vi "test Parse.vi"(11 "Test Case In":refnum<class "test EDS.lvclass">) -> (0 "error out":errorcluster, 3 "Test Case Out":refnum<class "test EDS.lvclass">)   [LabVIEW 2024, in "Test EDS.lvclass"]
uses:
  test EDS.lvclass
  C:/Program Files/National Instruments/LabVIEW 2024/vi.lib/Astemes/LUnit/Test Case.lvclass
  Core/EDS/EDS.lvclass
  <vilib>/PNR/JSONtext Object Serialization/Generic Object Serializer/Generic Object Serializer.lvclass
  C:/Program Files/National Instruments/LabVIEW 2024/vi.lib/JDP Science/JSONtext/LVClass Serializer/JSONtext LVClass Serializer.lvclass
  <vilib>/PNR/JSONtext Object Serialization/Generic Object Serializer/Type Name Handling.ctl
  <vilib>/PNR/JSONtext Object Serialization/Generic Object Serializer/Generic Object Serializer.lvclass/Generic Object Serializer.ctl
  Core/EDS/EDS.lvclass/EDS.ctl
  <vilib>/Astemes/LUnit/Test Case.lvclass/Test Case.ctl
  bdd25f00-0f07-479c-b713-0b173a884aa2.vi
  4993e8ee-a06a-463a-9684-69129f64d5ce.vi
  <vilib>/PNR/JSONtext Object Serialization/Generic Object Serializer/Write Type Name Handling.vi
  <vilib>/Astemes/LUnit/Append Pass Result.vi
  <vilib>/Astemes/LUnit/Append Fail Result.vi
  <vilib>/Astemes/LUnit/Describe Comparison.vi
  4993e8ee-a06a-463a-9684-69129f64d5ce.vi/9c5d11cd-9439-4240-a1ee-d9baace9c924.vi
  <vilib>/Astemes/LUnit/Run In UI.vi
  <vilib>/Utility/error.llb/Clear Errors.vi
  <vilib>/JDP Science/JSONtext/Variant to JSON Text.vi
  <vilib>/Astemes/LUnit/Describe Variant.vi
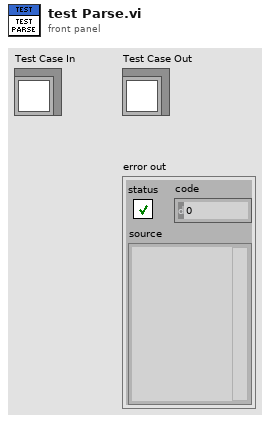
[diagram p1: front panel]
types:
  T1 = typedef "Generic Object Serializer.lvclass/Type Name Handling.ctl" = enum16{"None", "Inline"}
diagram:
  w9 = refnum<class "Generic Object Serializer.lvclass"> refnum  # Generic Object Serializer
  n1 = Current VI's Path() -> (path=w16:path)
  n2 = Strip Path(path=w16) -> (stripped path=w11:path)  [unwired: 1 out]
  n3 = Build Path(base path=w11, name or relative path=path "test.eds") -> (appended path=w12:path)
  n4 = Write to Text File(file (use dialog)=w12, text="[FileInfo]\nCreatedBy=Nanotec Electronic GmbH & Co. KG\nModifiedBy=Nanotec Electronic GmbH & Co. KG\nDescription=Motion controller\nCreationTime=00:00AM\nCreationDate=01-01-2000\nModificationTime=00:00AM\nModificationDate=01-01-2000\nFileName=C5-E-2-09.eds\nFileVersion=1\nFileRevision=1\nEDSVersion=4.0\n\n[DeviceInfo]\nVendorName=Nanotec Electronic GmbH & Co. KG\nVendorNumber=0x26C\nProductName=C5-E-2-09\nProductNumber=0x11\nRevisionNumber=0x8A50000\nOrderCode=na\nBaudRate_10=1\nBaudRate_20=1\nBaudRate_50=1\nBaudRate_125=1\nBaudRate_250=1\nBaudRate_500=1\nBaudRate_800=0\nBaudRate_1000=1\nSimpleBootUpMaster=0\nSimpleBootUpSlave=0\nGranularity=8\nDynamicChannelsSupported=0\nCompactPDO=0\nGroupMessaging=0\nNrOfRXPDO=8\nNrOfTXPDO=8\nLSS_Supported=0\n\n[DummyUsage]\nDummy0001=0\nDummy0002=1\nDummy0003=1\nDummy0004=1\nDummy0005=1\nDummy0006=1\nDummy0007=1\n\n[Comments]\nLines=0x00\n\n[MandatoryObjects]\nSupportedObjects=0x03\n1=0x1000\n2=0x1001\n3=0x1018\n\n[1000]\nParameterName=Device Type\nObjectType=0x7\nDataType=0x0007\nAccessType=ro\nDefaultValue=0x00060192\nPDOMapping=0\nObjFlags=1\n\n[1001]\nParameterName=Error Register\nObjectType=0x7\nDataType=0x0005\nAccessType=ro\nDefaultValue=0x00\nPDOMapping=1\nObjFlags=1\n\n[1018]\nParameterName=Identity Object\nObjectType=0x9\nSubNumber=0x05\n\n[1018sub0]\nParameterName=Number of entries\nObjectType=0x7\nDataType=0x0005\nAccessType=ro\nDefaultValue=0x04\nPDOMapping=0\nObjFlags=1\n\n[1018sub1]\nParameterName=Vendor-ID\nObjectType=0x7\nDataType=0x0007\nAccessType=ro\nDefaultValue=0x0000026C\nPDOMapping=0\nObjFlags=1\n\n[1018sub2]\nParameterName=Product code\nObjectType=0x7\nDataType=0x0007\nAccessType=ro\nDefaultValue=0x00000011\nPDOMapping=0\nObjFlags=1\n\n[1018sub3]\nParameterName=Revision number\nObjectType=0x7\nDataType=0x0007\nAccessType=ro\nDefaultValue=0x08A50000\nPDOMapping=0\nObjFlags=1\n\n[1018sub4]\nParameterName=Serial number\nObjectType=0x7\nDataType=0x0007\nAccessType=ro\nDefaultValue=\nPDOMapping=0\nObjFlags=1\n\n[OptionalObjects]\nSupportedObjects=0x91\n1=0x1003\n2=0x1005\n3=0x1006\n4=0x1007\n5=0x1008\n6=0x1009\n7=0x100A\n8=0x100C\n9=0x100D\n10=0x1010\n11=0x1011\n12=0x1014\n13=0x1016\n14=0x1017\n15=0x1019\n16=0x1020\n17=0x1029\n18=0x1400\n19=0x1401\n20=0x1402\n21=0x1403\n22=0x1404\n23=0x1405\n24=0x1406\n25=0x1407\n26=0x1600\n27=0x1601\n28=0x1602\n29=0x1603\n30=0x1604\n31=0x1605\n32=0x1606\n33=0x1607\n34=0x1800\n35=0x1801\n36=0x1802\n37=0x1803\n38=0x1804\n39=0x1805\n40=0x1806\n41=0x1807\n42=0x1A00\n43=0x1A01\n44=0x1A02\n45=0x1A03\n46=0x1A04\n47=0x1A05\n48=0x1A06\n49=0x1A07\n50=0x1F50\n51=0x1F51\n52=0x1F57\n53=0x1F80\n54=0x6007\n55=0x603F\n56=0x6040\n57=0x6041\n58=0x6042\n59=0x6043\n60=0x6044\n61=0x6046\n62=0x6048\n63=0x6049\n64=0x604A\n65=0x604C\n66=0x605A\n67=0x605B\n68=0x605C\n69=0x605D\n70=0x605E\n71=0x6060\n72=0x6061\n73=0x6062\n74=0x6063\n75=0x6064\n76=0x6065\n77=0x6066\n78=0x6067\n79=0x6068\n80=0x606B\n81=0x606C\n82=0x606D\n83=0x606E\n84=0x606F\n85=0x6070\n86=0x6071\n87=0x6072\n88=0x6073\n89=0x6074\n90=0x6075\n91=0x6077\n92=0x607A\n93=0x607B\n94=0x607C\n95=0x607D\n96=0x607E\n97=0x607F\n98=0x6080\n99=0x6081\n100=0x6082\n101=0x6083\n102=0x6084\n103=0x6085\n104=0x6086\n105=0x6087\n106=0x608F\n107=0x6090\n108=0x6091\n109=0x6092\n110=0x6096\n111=0x6097\n112=0x6098\n113=0x6099\n114=0x609A\n115=0x60A2\n116=0x60A4\n117=0x60A8\n118=0x60A9\n119=0x60B0\n120=0x60B1\n121=0x60B2\n122=0x60C1\n123=0x60C2\n124=0x60C4\n125=0x60C5\n126=0x60C6\n127=0x60E4\n128=0x60E5\n129=0x60E6\n130=0x60E8\n131=0x60E9\n132=0x60EB\n133=0x60ED\n134=0x60EE\n135=0x60F2\n136=0x60F4\n137=0x60F8\n138=0x60FA\n139=0x60FC\n140=0x60FD\n141=0x60FE\n142=0x60FF\n143=0x6502\n144=0x6503\n145=0x6505\n\n[1003]\nParameterName=Pre-defined error field\nObjectType=0x8\nSubNumber=0x09\n\n[1003sub0]\nParameterName=Number of errors\nObjectType=0x7\nDataType=0x0005\nAccessType=rw\nDefaultValue=0x00\nPDOMapping=0\nObjFlags=1\n\n[1003sub1]\nParameterName=1st Standard error field\nObjectType=0x7\nDataType=0x0007\nAccessType=ro\nPDOMapping=0\nObjFlags=1\n\n[1003sub2]\nParameterName=2nd Standard error field\nObjectType=0x7\nDataType=0x0007\nAccessType=ro\nPDOMapping=0\nObjFlags=1\n\n[1003sub3]\nParameterName=3th Standard error field\nObjectType=0x7\nDataType=0x0007\nAccessType=ro\nPDOMapping=0\nObjFlags=1\n\n[1003sub4]\nParameterName=4th Standard error field\nObjectType=0x7\nDataType=0x0007\nAccessType=ro\nPDOMapping=0\nObjFlags=1\n\n[1003sub5]\nParameterName=5th Standard error field\nObjectType=0x7\nDataType=0x0007\nAccessType=ro\nPDOMapping=0\nObjFlags=1\n\n[1003sub6]\nParameterName=6th Standard error field\nObjectType=0x7\nDataType=0x0007\nAccessType=ro\nPDOMapping=0\nObjFlags=1\n\n[1003sub7]\nParameterName=7th Standard error field\nObjectType=0x7\nDataType=0x0007\nAccessType=ro\nPDOMapping=0\nObjFlags=1\n\n[1003sub8]\nParameterName=8th Standard error field\nObjectType=0x7\nDataType=0x0007\nAccessType=ro\nPDOMapping=0\nObjFlags=1\n\n[1005]\nParameterName=COB-ID Sync\nObjectType=0x7\nDataType=0x0007\nAccessType=rw\nDefaultValue=0x00000080\nPDOMapping=0\n\n[1006]\nParameterName=Communication cycle period\nObjectType=0x7\nDataType=0x0007\nAccessType=rw\nDefaultValue=0x00000000\nPDOMapping=0\n\n[1007]\nParameterName=Synchronous Window Length\nObjectType=0x7\nDataType=0x0007\nAccessType=rw\nDefaultValue=0x00000000\nPDOMapping=0\n\n[1008]\nParameterName=Manufacturer Device Name\nObjectType=0x7\nDataType=0x0009\nAccessType=const\nDefaultValue=C5-E-2-09\nPDOMapping=0\nObjFlags=1\n\n[1009]\nParameterName=Manufacturer Hardware Version\nObjectType=0x7\nDataType=0x0009\nAccessType=const\nDefaultValue=\nPDOMapping=0\nObjFlags=1\n\n[100A]\nParameterName=Manufacturer Software Version\nObjectType=0x7\nDataType=0x0009\nAccessType=const\nDefaultValue=FIR-v2213-B1031134\nPDOMapping=0\nObjFlags=1\n\n[100C]\nParameterName=Guard Time\nObjectType=0x7\nDataType=0x0006\nAccessType=rw\nDefaultValue=0x0000\nPDOMapping=0\n\n[100D]\nParameterName=Live Time Factor\nObjectType=0x7\nDataType=0x0005\nAccessType=rw\nDefaultValue=0x00\nPDOMapping=0\n\n[1010]\nParameterName=Store parameters\nObjectType=0x8\nSubNumber=0x0E\n\n[1010sub0]\nParameterName=Number of entries\nObjectType=0x7\nDataType=0x0005\nAccessType=ro\nDefaultValue=0x0D\nPDOMapping=0\nObjFlags=1\n\n[1010sub1]\nParameterName=Save all parameters to non-volatile memory\nObjectType=0x7\nDataType=0x0007\nAccessType=rw\nDefaultValue=0x00000001\nPDOMapping=0\nObjFlags=1\n\n[1010sub2]\nParameterName=Save communication parameters to non-volatile memory\nObjectType=0x7\nDataType=0x0007\nAccessType=rw\nDefaultValue=0x00000001\nPDOMapping=0\nObjFlags=1\n\n[1010sub3]\nParameterName=Save application parameters to non-volatile memory\nObjectType=0x7\nDataType=0x0007\nAccessType=rw\nDefaultValue=0x00000001\nPDOMapping=0\nObjFlags=1\n\n[1010sub4]\nParameterName=Save customer parameters to non-volatile memory\nObjectType=0x7\nDataType=0x0007\nAccessType=rw\nDefaultValue=0x00000001\nPDOMapping=0\nObjFlags=1\n\n[1010sub5]\nParameterName=Save drive parameters to non-volatile memory\nObjectType=0x7\nDataType=0x0007\nAccessType=rw\nDefaultValue=0x00000001\nPDOMapping=0\nObjFlags=1\n\n[1010sub6]\nParameterName=Save tuning parameters to non-volatile memory\nObjectType=0x7\nDataType=0x0007\nAccessType=rw\nDefaultValue=0x00000001\nPDOMapping=0\nObjFlags=1\n\n[1010sub7]\nParameterName=Save miscellaneous configurations to non-volatile memory\nObjectType=0x7\nDataType=0x0007\nAccessType=rw\nDefaultValue=0x00000001\nPDOMapping=0\nObjFlags=1\n\n[1010sub8]\nParameterName=Save reserved1 configurations to non-volatile memory\nObjectType=0x7\nDataType=0x0007\nAccessType=rw\nDefaultValue=0x00000000\nPDOMapping=0\nObjFlags=1\n\n[1010sub9]\nParameterName=Save reserved2 configurations to non-volatile memory\nObjectType=0x7\nDataType=0x0007\nAccessType=rw\nDefaultValue=0x00000000\nPDOMapping=0\nObjFlags=1\n\n[1010subA]\nParameterName=Save CANopen configurations to non-volatile memory\nObjectType=0x7\nDataType=0x0007\nAccessType=rw\nDefaultValue=0x00000001\nPDOMapping=0\nObjFlags=1\n\n[1010subB]\nParameterName=Save Modbus RTU configurations to non-volatile memory\nObjectType=0x7\nDataType=0x0007\nAccessType=rw\nDefaultValue=0x00000001\nPDOMapping=0\nObjFlags=1\n\n[1010subC]\nParameterName=Save Ethernet configurations to non-volatile memory\nObjectType=0x7\nDataType=0x0007\nAccessType=rw\nDefaultValue=0x00000001\nPDOMapping=0\nObjFlags=1\n\n[1010subD]\nParameterName=Save Profibus configurations to non-volatile memory\nObjectType=0x7\nDataType=0x0007\nAccessType=rw\nDefaultValue=0x00000001\nPDOMapping=0\nObjFlags=1\n\n[1011]\nParameterName=Restore default parameters\nObjectType=0x8\nSubNumber=0x0E\n\n[1011sub0]\nParameterName=Number of entries\nObjectType=0x7\nDataType=0x0005\nAccessType=ro\nDefaultValue=0x0D\nPDOMapping=0\nObjFlags=1\n\n[1011sub1]\nParameterName=Restore all default parameters\nObjectType=0x7\nDataType=0x0007\nAccessType=rw\nDefaultValue=0x00000001\nPDOMapping=0\nObjFlags=1\n\n[1011sub2]\nParameterName=Restore communication default parameters\nObjectType=0x7\nDataType=0x0007\nAccessType=rw\nDefaultValue=0x00000001\nPDOMapping=0\nObjFlags=1\n\n[1011sub3]\nParameterName=Restore application default parameters\nObjectType=0x7\nDataType=0x0007\nAccessType=rw\nDefaultValue=0x00000001\nPDOMapping=0\nObjFlags=1\n\n[1011sub4]\nParameterName=Restore customer default parameters\nObjectType=0x7\nDataType=0x0007\nAccessType=rw\nDefaultValue=0x00000001\nPDOMapping=0\nObjFlags=1\n\n[1011sub5]\nParameterName=Restore drive default parameters\nObjectType=0x7\nDataType=0x0007\nAccessType=rw\nDefaultValue=0x00000001\nPDOMapping=0\nObjFlags=1\n\n[1011sub6]\nParameterName=Restore tuning default parameters\nObjectType=0x7\nDataType=0x0007\nAccessType=rw\nDefaultValue=0x00000001\nPDOMapping=0\nObjFlags=1\n\n[1011sub7]\nParameterName=Restore miscellaneous configurations\nObjectType=0x7\nDataType=0x0007\nAccessType=rw\nDefaultValue=0x00000001\nPDOMapping=0\nObjFlags=1\n\n[1011sub8]\nParameterName=Restore reserved1 configurations to non-volatile memory\nObjectType=0x7\nDataType=0x0007\nAccessType=rw\nDefaultValue=0x00000000\nPDOMapping=0\nObjFlags=1\n\n[1011sub9]\nParameterName=Restore reserved2 configurations to non-volatile memory\nObjectType=0x7\nDataType=0x0007\nAccessType=rw\nDefaultValue=0x00000000\nPDOMapping=0\nObjFlags=1\n\n[1011subA]\nParameterName=Restore CANopen configurations to non-volatile memory\nObjectType=0x7\nDataType=0x0007\nAccessType=rw\nDefaultValue=0x00000001\nPDOMapping=0\nObjFlags=1\n\n[1011subB]\nParameterName=Restore Modbus RTU configurations to non-volatile memory\nObjectType=0x7\nDataType=0x0007\nAccessType=rw\nDefaultValue=0x00000001\nPDOMapping=0\nObjFlags=1\n\n[1011subC]\nParameterName=Restore Ethernet configurations to non-volatile memory\nObjectType=0x7\nDataType=0x0007\nAccessType=rw\nDefaultValue=0x00000001\nPDOMapping=0\nObjFlags=1\n\n[1011subD]\nParameterName=Restore Profibus configurations to non-volatile memory\nObjectType=0x7\nDataType=0x0007\nAccessType=rw\nDefaultValue=0x00000001\nPDOMapping=0\nObjFlags=1\n\n[1014]\nParameterName=COB-ID EMCY\nObjectType=0x7\nDataType=0x0007\nAccessType=rw\nDefaultValue=$NODEID+0x80\nPDOMapping=0\n\n[1016]\nParameterName=Consumer heartbeat time\nObjectType=0x8\nSubNumber=0x02\n\n[1016sub0]\nParameterName=Number of entries\nObjectType=0x7\nDataType=0x0005\nAccessType=ro\nDefaultValue=0x01\nPDOMapping=0\n\n[1016sub1]\nParameterName=Consumer heartbeat time\nObjectType=0x7\nDataType=0x0007\nAccessType=rw\nDefaultValue=0x00000000\nPDOMapping=0\n\n[1017]\nParameterName=Producer heartbeat time\nObjectType=0x7\nDataType=0x0006\nAccessType=rw\nDefaultValue=0x0000\nPDOMapping=0\n\n[1019]\nParameterName=Synchronous counter overflow value\nObjectType=0x7\nDataType=0x0005\nAccessType=rw\nDefaultValue=0x00\nPDOMapping=0\n\n[1020]\nParameterName=Verify Configuration\nObjectType=0x8\nSubNumber=0x03\n\n[1020sub0]\nParameterName=Number of entries\nObjectType=0x7\nDataType=0x0005\nAccessType=ro\nDefaultValue=0x02\nPDOMapping=0\n\n[1020sub1]\nParameterName=Configuration date\nObjectType=0x7\nDataType=0x0007\nAccessType=rw\nDefaultValue=0x00000000\nPDOMapping=0\n\n[1020sub2]\nParameterName=Configuration time\nObjectType=0x7\nDataType=0x0007\nAccessType=rw\nDefaultValue=0x00000000\nPDOMapping=0\n\n[1029]\nParameterName=Error behavior\nObjectType=0x8\nSubNumber=0x03\n\n[1029sub0]\nParameterName=Number of entries\nObjectType=0x7\nDataType=0x0005\nAccessType=ro\nDefaultValue=0x02\nPDOMapping=0\n\n[1029sub1]\nParameterName=Communication error\nObjectType=0x7\nDataType=0x0005\nAccessType=rw\nDefaultValue=0x00\nPDOMapping=0\n\n[1029sub2]\nParameterName=Internal device error\nObjectType=0x7\nDataType=0x0005\nAccessType=rw\nDefaultValue=0x01\nPDOMapping=0\n\n[1400]\nParameterName=Receive PDO 1 Communication Parameter\nObjectType=0x9\nSubNumber=0x03\n\n[1400sub0]\nParameterName=Number of entries\nObjectType=0x7\nDataType=0x0005\nAccessType=ro\nDefaultValue=0x02\nPDOMapping=0\n\n[1400sub1]\nParameterName=COB-ID\nObjectType=0x7\nDataType=0x0007\nAccessType=rw\nDefaultValue=$NODEID+0x200\nPDOMapping=0\n\n[1400sub2]\nParameterName=Transmission Type\nObjectType=0x7\nDataType=0x0005\nAccessType=rw\nDefaultValue=0xFF\nPDOMapping=0\n\n[1401]\nParameterName=Receive PDO 2 Communication Parameter\nObjectType=0x9\nSubNumber=0x03\n\n[1401sub0]\nParameterName=Number of entries\nObjectType=0x7\nDataType=0x0005\nAccessType=ro\nDefaultValue=0x02\nPDOMapping=0\n\n[1401sub1]\nParameterName=COB-ID\nObjectType=0x7\nDataType=0x0007\nAccessType=rw\nDefaultValue=$NODEID+0x300\nPDOMapping=0\n\n[1401sub2]\nParameterName=Transmission Type\nObjectType=0x7\nDataType=0x0005\nAccessType=rw\nDefaultValue=0xFF\nPDOMapping=0\n\n[1402]\nParameterName=Receive PDO 3 Communication Parameter\nObjectType=0x9\nSubNumber=0x03\n\n[1402sub0]\nParameterName=Number of entries\nObjectType=0x7\nDataType=0x0005\nAccessType=ro\nDefaultValue=0x02\nPDOMapping=0\n\n[1402sub1]\nParameterName=COB-ID\nObjectType=0x7\nDataType=0x0007\nAccessType=rw\nDefaultValue=$NODEID+0x400\nPDOMapping=0\n\n[1402sub2]\nParameterName=Transmission Type\nObjectType=0x7\nDataType=0x0005\nAccessType=rw\nDefaultValue=0xFF\nPDOMapping=0\n\n[1403]\nParameterName=Receive PDO 4 Communication Parameter\nObjectType=0x9\nSubNumber=0x03\n\n[1403sub0]\nParameterName=Number of entries\nObjectType=0x7\nDataType=0x0005\nAccessType=ro\nDefaultValue=0x02\nPDOMapping=0\n\n[1403sub1]\nParameterName=COB-ID\nObjectType=0x7\nDataType=0x0007\nAccessType=rw\nDefaultValue=$NODEID+0x500\nPDOMapping=0\n\n[1403sub2]\nParameterName=Transmission Type\nObjectType=0x7\nDataType=0x0005\nAccessType=rw\nDefaultValue=0xFF\nPDOMapping=0\n\n[1404]\nParameterName=Receive PDO 5 Communication Parameter\nObjectType=0x9\nSubNumber=0x03\n\n[1404sub0]\nParameterName=Number of entries\nObjectType=0x7\nDataType=0x0005\nAccessType=ro\nDefaultValue=0x02\nPDOMapping=0\n\n[1404sub1]\nParameterName=COB-ID\nObjectType=0x7\nDataType=0x0007\nAccessType=rw\nDefaultValue=0x80000000\nPDOMapping=0\n\n[1404sub2]\nParameterName=Transmission Type\nObjectType=0x7\nDataType=0x0005\nAccessType=rw\nDefaultValue=0xFF\nPDOMapping=0\n\n[1405]\nParameterName=Receive PDO 6 Communication Parameter\nObjectType=0x9\nSubNumber=0x03\n\n[1405sub0]\nParameterName=Number of entries\nObjectType=0x7\nDataType=0x0005\nAccessType=ro\nDefaultValue=0x02\nPDOMapping=0\n\n[1405sub1]\nParameterName=COB-ID\nObjectType=0x7\nDataType=0x0007\nAccessType=rw\nDefaultValue=0x80000000\nPDOMapping=0\n\n[1405sub2]\nParameterName=Transmission Type\nObjectType=0x7\nDataType=0x0005\nAccessType=rw\nDefaultValue=0xFF\nPDOMapping=0\n\n[1406]\nParameterName=Receive PDO 7 Communication Parameter\nObjectType=0x9\nSubNumber=0x03\n\n[1406sub0]\nParameterName=Number of entries\nObjectType=0x7\nDataType=0x0005\nAccessType=ro\nDefaultValue=0x02\nPDOMapping=0\n\n[1406sub1]\nParameterName=COB-ID\nObjectType=0x7\nDataType=0x0007\nAccessType=rw\nDefaultValue=0x80000000\nPDOMapping=0\n\n[1406sub2]\nParameterName=Transmission Type\nObjectType=0x7\nDataType=0x0005\nAccessType=rw\nDefaultValue=0xFF\nPDOMapping=0\n\n[1407]\nParameterName=Receive PDO 8 Communication Parameter\nObjectType=0x9\nSubNumber=0x03\n\n[1407sub0]\nParameterName=Number of entries\nObjectType=0x7\nDataType=0x0005\nAccessType=ro\nDefaultValue=0x02\nPDOMapping=0\n\n[1407sub1]\nParameterName=COB-ID\nObjectType=0x7\nDataType=0x0007\nAccessType=rw\nDefaultValue=0x80000000\nPDOMapping=0\n\n[1407sub2]\nParameterName=Transmission Type\nObjectType=0x7\nDataType=0x0005\nAccessType=rw\nDefaultValue=0xFF\nPDOMapping=0\n\n[1600]\nParameterName=Receive PDO 1 Mapping Parameter\nObjectType=0x9\nSubNumber=0x09\n\n[1600sub0]\nParameterName=Number of entries\nObjectType=0x7\nDataType=0x0005\nAccessType=rw\nDefaultValue=0x02\nPDOMapping=0\n\n[1600sub1]\nParameterName=1st object to be mapped\nObjectType=0x7\nDataType=0x0007\nAccessType=rw\nDefaultValue=0x60400010\nPDOMapping=0\n\n[1600sub2]\nParameterName=2nd object to be mapped\nObjectType=0x7\nDataType=0x0007\nAccessType=rw\nDefaultValue=0x60600008\nPDOMapping=0\n\n[1600sub3]\nParameterName=3rd object to be mapped\nObjectType=0x7\nDataType=0x0007\nAccessType=rw\nDefaultValue=0x00000000\nPDOMapping=0\n\n[1600sub4]\nParameterName=4th object to be mapped\nObjectType=0x7\nDataType=0x0007\nAccessType=rw\nDefaultValue=0x00000000\nPDOMapping=0\n\n[1600sub5]\nParameterName=5th object to be mapped\nObjectType=0x7\nDataType=0x0007\nAccessType=rw\nDefaultValue=0x00000000\nPDOMapping=0\n\n[1600sub6]\nParameterName=6th object to be mapped\nObjectType=0x7\nDataType=0x0007\nAccessType=rw\nDefaultValue=0x00000000\nPDOMapping=0\n\n[1600sub7]\nParameterName=7th object to be mapped\nObjectType=0x7\nDataType=0x0007\nAccessType=rw\nDefaultValue=0x00000000\nPDOMapping=0\n\n[1600sub8]\nParameterName=8th object to be mapped\nObjectType=0x7\nDataType=0x0007\nAccessType=rw\nDefaultValue=0x00000000\nPDOMapping=0\n\n[1601]\nParameterName=Receive PDO 2 Mapping Parameter\nObjectType=0x9\nSubNumber=0x09\n\n[1601sub0]\nParameterName=Number of entries\nObjectType=0x7\nDataType=0x0005\nAccessType=rw\nDefaultValue=0x02\nPDOMapping=0\n\n[1601sub1]\nParameterName=1st object to be mapped\nObjectType=0x7\nDataType=0x0007\nAccessType=rw\nDefaultValue=0x607A0020\nPDOMapping=0\n\n[1601sub2]\nParameterName=2nd object to be mapped\nObjectType=0x7\nDataType=0x0007\nAccessType=rw\nDefaultValue=0x60810020\nPDOMapping=0\n\n[1601sub3]\nParameterName=3rd object to be mapped\nObjectType=0x7\nDataType=0x0007\nAccessType=rw\nDefaultValue=0x00000000\nPDOMapping=0\n\n[1601sub4]\nParameterName=4th object to be mapped\nObjectType=0x7\nDataType=0x0007\nAccessType=rw\nDefaultValue=0x00000000\nPDOMapping=0\n\n[1601sub5]\nParameterName=5th object to be mapped\nObjectType=0x7\nDataType=0x0007\nAccessType=rw\nDefaultValue=0x00000000\nPDOMapping=0\n\n[1601sub6]\nParameterName=6th object to be mapped\nObjectType=0x7\nDataType=0x0007\nAccessType=rw\nDefaultValue=0x00000000\nPDOMapping=0\n\n[1601sub7]\nParameterName=7th object to be mapped\nObjectType=0x7\nDataType=0x0007\nAccessType=rw\nDefaultValue=0x00000000\nPDOMapping=0\n\n[1601sub8]\nParameterName=8th object to be mapped\nObjectType=0x7\nDataType=0x0007\nAccessType=rw\nDefaultValue=0x00000000\nPDOMapping=0\n\n[1602]\nParameterName=Receive PDO 3 Mapping Parameter\nObjectType=0x9\nSubNumber=0x09\n\n[1602sub0]\nParameterName=Number of entries\nObjectType=0x7\nDataType=0x0005\nAccessType=rw\nDefaultValue=0x01\nPDOMapping=0\n\n[1602sub1]\nParameterName=1st object to be mapped\nObjectType=0x7\nDataType=0x0007\nAccessType=rw\nDefaultValue=0x60420010\nPDOMapping=0\n\n[1602sub2]\nParameterName=2nd object to be mapped\nObjectType=0x7\nDataType=0x0007\nAccessType=rw\nDefaultValue=0x00000000\nPDOMapping=0\n\n[1602sub3]\nParameterName=3rd object to be mapped\nObjectType=0x7\nDataType=0x0007\nAccessType=rw\nDefaultValue=0x00000000\nPDOMapping=0\n\n[1602sub4]\nParameterName=4th object to be mapped\nObjectType=0x7\nDataType=0x0007\nAccessType=rw\nDefaultValue=0x00000000\nPDOMapping=0\n\n[1602sub5]\nParameterName=5th object to be mapped\nObjectType=0x7\nDataType=0x0007\nAccessType=rw\nDefaultValue=0x00000000\nPDOMapping=0\n\n[1602sub6]\nParameterName=6th object to be mapped\nObjectType=0x7\nDataType=0x0007\nAccessType=rw\nDefaultValue=0x00000000\nPDOMapping=0\n\n[1602sub7]\nParameterName=7th object to be mapped\nObjectType=0x7\nDataType=0x0007\nAccessType=rw\nDefaultValue=0x00000000\nPDOMapping=0\n\n[1602sub8]\nParameterName=8th object to be mapped\nObjectType=0x7\nDataType=0x0007\nAccessType=rw\nDefaultValue=0x00000000\nPDOMapping=0\n\n[1603]\nParameterName=Receive PDO 4 Mapping Parameter\nObjectType=0x9\nSubNumber=0x09\n\n[1603sub0]\nParameterName=Number of entries\nObjectType=0x7\nDataType=0x0005\nAccessType=rw\nDefaultValue=0x01\nPDOMapping=0\n\n[1603sub1]\nParameterName=1st object to be mapped\nObjectType=0x7\nDataType=0x0007\nAccessType=rw\nDefaultValue=0x60FE0120\nPDOMapping=0\n\n[1603sub2]\nParameterName=2nd object to be mapped\nObjectType=0x7\nDataType=0x0007\nAccessType=rw\nDefaultValue=0x00000000\nPDOMapping=0\n\n[1603sub3]\nParameterName=3rd object to be mapped\nObjectType=0x7\nDataType=0x0007\nAccessType=rw\nDefaultValue=0x00000000\nPDOMapping=0\n\n[1603sub4]\nParameterName=4th object to be mapped\nObjectType=0x7\nDataType=0x0007\nAccessType=rw\nDefaultValue=0x00000000\nPDOMapping=0\n\n[1603sub5]\nParameterName=5th object to be mapped\nObjectType=0x7\nDataType=0x0007\nAccessType=rw\nDefaultValue=0x00000000\nPDOMapping=0\n\n[1603sub6]\nParameterName=6th object to be mapped\nObjectType=0x7\nDataType=0x0007\nAccessType=rw\nDefaultValue=0x00000000\nPDOMapping=0\n\n[1603sub7]\nParameterName=7th object to be mapped\nObjectType=0x7\nDataType=0x0007\nAccessType=rw\nDefaultValue=0x00000000\nPDOMapping=0\n\n[1603sub8]\nParameterName=8th object to be mapped\nObjectType=0x7\nDataType=0x0007\nAccessType=rw\nDefaultValue=0x00000000\nPDOMapping=0\n\n[1604]\nParameterName=Receive PDO 5 Mapping Parameter\nObjectType=0x9\nSubNumber=0x09\n\n[1604sub0]\nParameterName=Number of entries\nObjectType=0x7\nDataType=0x0005\nAccessType=rw\nDefaultValue=0x00\nPDOMapping=0\n\n[1604sub1]\nParameterName=1st object to be mapped\nObjectType=0x7\nDataType=0x0007\nAccessType=rw\nDefaultValue=0x00000000\nPDOMapping=0\n\n[1604sub2]\nParameterName=2nd object to be mapped\nObjectType=0x7\nDataType=0x0007\nAccessType=rw\nDefaultValue=0x00000000\nPDOMapping=0\n\n[1604sub3]\nParameterName=3rd object to be mapped\nObjectType=0x7\nDataType=0x0007\nAccessType=rw\nDefaultValue=0x00000000\nPDOMapping=0\n\n[1604sub4]\nParameterName=4th object to be mapped\nObjectType=0x7\nDataType=0x0007\nAccessType=rw\nDefaultValue=0x00000000\nPDOMapping=0\n\n[1604sub5]\nParameterName=5th object to be mapped\nObjectType=0x7\nDataType=0x0007\nAccessType=rw\nDefaultValue=0x00000000\nPDOMapping=0\n\n[1604sub6]\nParameterName=6th object to be mapped\nObjectType=0x7\nDataType=0x0007\nAccessType=rw\nDefaultValue=0x00000000\nPDOMapping=0\n\n[1604sub7]\nParameterName=7th object to be mapped\nObjectType=0x7\nDataType=0x0007\nAccessType=rw\nDefaultValue=0x00000000\nPDOMapping=0\n\n[1604sub8]\nParameterName=8th object to be mapped\nObjectType=0x7\nDataType=0x0007\nAccessType=rw\nDefaultValue=0x00000000\nPDOMapping=0\n\n[1605]\nParameterName=Receive PDO 6 Mapping Parameter\nObjectType=0x9\nSubNumber=0x09\n\n[1605sub0]\nParameterName=Number of entries\nObjectType=0x7\nDataType=0x0005\nAccessType=rw\nDefaultValue=0x00\nPDOMapping=0\n\n[1605sub1]\nParameterName=1st object to be mapped\nObjectType=0x7\nDataType=0x0007\nAccessType=rw\nDefaultValue=0x00000000\nPDOMapping=0\n\n[1605sub2]\nParameterName=2nd object to be mapped\nObjectType=0x7\nDataType=0x0007\nAccessType=rw\nDefaultValue=0x00000000\nPDOMapping=0\n\n[1605sub3]\nParameterName=3rd object to be mapped\nObjectType=0x7\nDataType=0x0007\nAccessType=rw\nDefaultValue=0x00000000\nPDOMapping=0\n\n[1605sub4]\nParameterName=4th object to be mapped\nObjectType=0x7\nDataType=0x0007\nAccessType=rw\nDefaultValue=0x00000000\nPDOMapping=0\n\n[1605sub5]\nParameterName=5th object to be mapped\nObjectType=0x7\nDataType=0x0007\nAccessType=rw\nDefaultValue=0x00000000\nPDOMapping=0\n\n[1605sub6]\nParameterName=6th object to be mapped\nObjectType=0x7\nDataType=0x0007\nAccessType=rw\nDefaultValue=0x00000000\nPDOMapping=0\n\n[1605sub7]\nParameterName=7th object to be mapped\nObjectType=0x7\nDataType=0x0007\nAccessType=rw\nDefaultValue=0x00000000\nPDOMapping=0\n\n[1605sub8]\nParameterName=8th object to be mapped\nObjectType=0x7\nDataType=0x0007\nAccessType=rw\nDefaultValue=0x00000000\nPDOMapping=0\n\n[1606]\nParameterName=Receive PDO 7 Mapping Parameter\nObjectType=0x9\nSubNumber=0x09\n\n[1606sub0]\nParameterName=Number of entries\nObjectType=0x7\nDataType=0x0005\nAccessType=rw\nDefaultValue=0x00\nPDOMapping=0\n\n[1606sub1]\nParameterName=1st object to be mapped\nObjectType=0x7\nDataType=0x0007\nAccessType=rw\nDefaultValue=0x00000000\nPDOMapping=0\n\n[1606sub2]\nParameterName=2nd object to be mapped\nObjectType=0x7\nDataType=0x0007\nAccessType=rw\nDefaultValue=0x00000000\nPDOMapping=0\n\n[1606sub3]\nParameterName=3rd object to be mapped\nObjectType=0x7\nDataType=0x0007\nAccessType=rw\nDefaultValue=0x00000000\nPDOMapping=0\n\n[1606sub4]\nParameterName=4th object to be mapped\nObjectType=0x7\nDataType=0x0007\nAccessType=rw\nDefaultValue=0x00000000\nPDOMapping=0\n\n[1606sub5]\nParameterName=5th object to be mapped\nObjectType=0x7\nDataType=0x0007\nAccessType=rw\nDefaultValue=0x00000000\nPDOMapping=0\n\n[1606sub6]\nParameterName=6th object to be mapped\nObjectType=0x7\nDataType=0x0007\nAccessType=rw\nDefaultValue=0x00000000\nPDOMapping=0\n\n[1606sub7]\nParameterName=7th object to be mapped\nObjectType=0x7\nDataType=0x0007\nAccessType=rw\nDefaultValue=0x00000000\nPDOMapping=0\n\n[1606sub8]\nParameterName=8th object to be mapped\nObjectType=0x7\nDataType=0x0007\nAccessType=rw\nDefaultValue=0x00000000\nPDOMapping=0\n\n[1607]\nParameterName=Receive PDO 8 Mapping Parameter\nObjectType=0x9\nSubNumber=0x09\n\n[1607sub0]\nParameterName=Number of entries\nObjectType=0x7\nDataType=0x0005\nAccessType=rw\nDefaultValue=0x00\nPDOMapping=0\n\n[1607sub1]\nParameterName=1st object to be mapped\nObjectType=0x7\nDataType=0x0007\nAccessType=rw\nDefaultValue=0x00000000\nPDOMapping=0\n\n[1607sub2]\nParameterName=2nd object to be mapped\nObjectType=0x7\nDataType=0x0007\nAccessType=rw\nDefaultValue=0x00000000\nPDOMapping=0\n\n[1607sub3]\nParameterName=3rd object to be mapped\nObjectType=0x7\nDataType=0x0007\nAccessType=rw\nDefaultValue=0x00000000\nPDOMapping=0\n\n[1607sub4]\nParameterName=4th object to be mapped\nObjectType=0x7\nDataType=0x0007\nAccessType=rw\nDefaultValue=0x00000000\nPDOMapping=0\n\n[1607sub5]\nParameterName=5th object to be mapped\nObjectType=0x7\nDataType=0x0007\nAccessType=rw\nDefaultValue=0x00000000\nPDOMapping=0\n\n[1607sub6]\nParameterName=6th object to be mapped\nObjectType=0x7\nDataType=0x0007\nAccessType=rw\nDefaultValue=0x00000000\nPDOMapping=0\n\n[1607sub7]\nParameterName=7th object to be mapped\nObjectType=0x7\nDataType=0x0007\nAccessType=rw\nDefaultValue=0x00000000\nPDOMapping=0\n\n[1607sub8]\nParameterName=8th object to be mapped\nObjectType=0x7\nDataType=0x0007\nAccessType=rw\nDefaultValue=0x00000000\nPDOMapping=0\n\n[1800]\nParameterName=Transmit PDO 1 Communication Parameter\nObjectType=0x9\nSubNumber=0x07\n\n[1800sub0]\nParameterName=Number of entries\nObjectType=0x7\nDataType=0x0005\nAccessType=ro\nDefaultValue=0x06\nPDOMapping=0\n\n[1800sub1]\nParameterName=COB-ID\nObjectType=0x7\nDataType=0x0007\nAccessType=rw\nDefaultValue=$NODEID+0x180\nPDOMapping=0\n\n[1800sub2]\nParameterName=Transmission Type\nObjectType=0x7\nDataType=0x0005\nAccessType=rw\nDefaultValue=0xFF\nPDOMapping=0\n\n[1800sub3]\nParameterName=Inhibit Time\nObjectType=0x7\nDataType=0x0006\nAccessType=rw\nDefaultValue=0x0064\nPDOMapping=0\n\n[1800sub4]\nParameterName=Compatibility Entry\nObjectType=0x7\nDataType=0x0005\nAccessType=rw\nDefaultValue=0x00\nPDOMapping=0\n\n[1800sub5]\nParameterName=Event Timer\nObjectType=0x7\nDataType=0x0006\nAccessType=rw\nDefaultValue=0x0000\nPDOMapping=0\n\n[1800sub6]\nParameterName=SYNC start value\nObjectType=0x7\nDataType=0x0005\nAccessType=rw\nDefaultValue=0x00\nPDOMapping=0\n\n[1801]\nParameterName=Transmit PDO 2 Communication Parameter\nObjectType=0x9\nSubNumber=0x07\n\n[1801sub0]\nParameterName=Number of entries\nObjectType=0x7\nDataType=0x0005\nAccessType=ro\nDefaultValue=0x06\nPDOMapping=0\n\n[1801sub1]\nParameterName=COB-ID\nObjectType=0x7\nDataType=0x0007\nAccessType=rw\nDefaultValue=$NODEID+0x280\nPDOMapping=0\n\n[1801sub2]\nParameterName=Transmission Type\nObjectType=0x7\nDataType=0x0005\nAccessType=rw\nDefaultValue=0xFF\nPDOMapping=0\n\n[1801sub3]\nParameterName=Inhibit Time\nObjectType=0x7\nDataType=0x0006\nAccessType=rw\nDefaultValue=0x0064\nPDOMapping=0\n\n[1801sub4]\nParameterName=Compatibility Entry\nObjectType=0x7\nDataType=0x0005\nAccessType=rw\nDefaultValue=0x00\nPDOMapping=0\n\n[1801sub5]\nParameterName=Event Timer\nObjectType=0x7\nDataType=0x0006\nAccessType=rw\nDefaultValue=0x0000\nPDOMapping=0\n\n[1801sub6]\nParameterName=SYNC start value\nObjectType=0x7\nDataType=0x0005\nAccessType=rw\nDefaultValue=0x00\nPDOMapping=0\n\n[1802]\nParameterName=Transmit PDO 3 Communication Parameter\nObjectType=0x9\nSubNumber=0x07\n\n[1802sub0]\nParameterName=Number of entries\nObjectType=0x7\nDataType=0x0005\nAccessType=ro\nDefaultValue=0x06\nPDOMapping=0\n\n[1802sub1]\nParameterName=COB-ID\nObjectType=0x7\nDataType=0x0007\nAccessType=rw\nDefaultValue=$NODEID+0x380\nPDOMapping=0\n\n[1802sub2]\nParameterName=Transmission Type\nObjectType=0x7\nDataType=0x0005\nAccessType=rw\nDefaultValue=0xFF\nPDOMapping=0\n\n[1802sub3]\nParameterName=Inhibit Time\nObjectType=0x7\nDataType=0x0006\nAccessType=rw\nDefaultValue=0x0064\nPDOMapping=0\n\n[1802sub4]\nParameterName=Compatibility Entry\nObjectType=0x7\nDataType=0x0005\nAccessType=rw\nDefaultValue=0x00\nPDOMapping=0\n\n[1802sub5]\nParameterName=Event Timer\nObjectType=0x7\nDataType=0x0006\nAccessType=rw\nDefaultValue=0x0000\nPDOMapping=0\n\n[1802sub6]\nParameterName=SYNC start value\nObjectType=0x7\nDataType=0x0005\nAccessType=rw\nDefaultValue=0x00\nPDOMapping=0\n\n[1803]\nParameterName=Transmit PDO 4 Communication Parameter\nObjectType=0x9\nSubNumber=0x07\n\n[1803sub0]\nParameterName=Number of entries\nObjectType=0x7\nDataType=0x0005\nAccessType=ro\nDefaultValue=0x06\nPDOMapping=0\n\n[1803sub1]\nParameterName=COB-ID\nObjectType=0x7\nDataType=0x0007\nAccessType=rw\nDefaultValue=$NODEID+0x480\nPDOMapping=0\n\n[1803sub2]\nParameterName=Transmission Type\nObjectType=0x7\nDataType=0x0005\nAccessType=rw\nDefaultValue=0xFF\nPDOMapping=0\n\n[1803sub3]\nParameterName=Inhibit Time\nObjectType=0x7\nDataType=0x0006\nAccessType=rw\nDefaultValue=0x0064\nPDOMapping=0\n\n[1803sub4]\nParameterName=Compatibility Entry\nObjectType=0x7\nDataType=0x0005\nAccessType=rw\nDefaultValue=0x00\nPDOMapping=0\n\n[1803sub5]\nParameterName=Event Timer\nObjectType=0x7\nDataType=0x0006\nAccessType=rw\nDefaultValue=0x0000\nPDOMapping=0\n\n[1803sub6]\nParameterName=SYNC start value\nObjectType=0x7\nDataType=0x0005\nAccessType=rw\nDefaultValue=0x00\nPDOMapping=0\n\n[1804]\nParameterName=Transmit PDO 5 Communication Parameter\nObjectType=0x9\nSubNumber=0x07\n\n[1804sub0]\nParameterName=Number of entries\nObjectType=0x7\nDataType=0x0005\nAccessType=ro\nDefaultValue=0x06\nPDOMapping=0\n\n[1804sub1]\nParameterName=COB-ID\nObjectType=0x7\nDataType=0x0007\nAccessType=rw\nDefaultValue=0xC0000000\nPDOMapping=0\n\n[1804sub2]\nParameterName=Transmission Type\nObjectType=0x7\nDataType=0x0005\nAccessType=rw\nDefaultValue=0xFF\nPDOMapping=0\n\n[1804sub3]\nParameterName=Inhibit Time\nObjectType=0x7\nDataType=0x0006\nAccessType=rw\nDefaultValue=0x0064\nPDOMapping=0\n\n[1804sub4]\nParameterName=Compatibility Entry\nObjectType=0x7\nDataType=0x0005\nAccessType=rw\nDefaultValue=0x00\nPDOMapping=0\n\n[1804sub5]\nParameterName=Event Timer\nObjectType=0x7\nDataType=0x0006\nAccessType=rw\nDefaultValue=0x0000\nPDOMapping=0\n\n[1804sub6]\nParameterName=SYNC start value\nObjectType=0x7\nDataType=0x0005\nAccessType=rw\nDefaultValue=0x00\nPDOMapping=0\n\n[1805]\nParameterName=Transmit PDO 6 Communication Parameter\nObjectType=0x9\nSubNumber=0x07\n\n[1805sub0]\nParameterName=Number of entries\nObjectType=0x7\nDataType=0x0005\nAccessType=ro\nDefaultValue=0x06\nPDOMapping=0\n\n[1805sub1]\nParameterName=COB-ID\nObjectType=0x7\nDataType=0x0007\nAccessType=rw\nDefaultValue=0xC0000000\nPDOMapping=0\n\n[1805sub2]\nParameterName=Transmission Type\nObjectType=0x7\nDataType=0x0005\nAccessType=rw\nDefaultValue=0xFF\nPDOMapping=0\n\n[1805sub3]\nParameterName=Inhibit Time\nObjectType=0x7\nDataType=0x0006\nAccessType=rw\nDefaultValue=0x0064\nPDOMapping=0\n\n[1805sub4]\nParameterName=Compatibility Entry\nObjectType=0x7\nDataType=0x0005\nAccessType=rw\nDefaultValue=0x00\nPDOMapping=0\n\n[1805sub5]\nParameterName=Event Timer\nObjectType=0x7\nDataType=0x0006\nAccessType=rw\nDefaultValue=0x0000\nPDOMapping=0\n\n[1805sub6]\nParameterName=SYNC start value\nObjectType=0x7\nDataType=0x0005\nAccessType=rw\nDefaultValue=0x00\nPDOMapping=0\n\n[1806]\nParameterName=Transmit PDO 7 Communication Parameter\nObjectType=0x9\nSubNumber=0x07\n\n[1806sub0]\nParameterName=Number of entries\nObjectType=0x7\nDataType=0x0005\nAccessType=ro\nDefaultValue=0x06\nPDOMapping=0\n\n[1806sub1]\nParameterName=COB-ID\nObjectType=0x7\nDataType=0x0007\nAccessType=rw\nDefaultValue=0xC0000000\nPDOMapping=0\n\n[1806sub2]\nParameterName=Transmission Type\nObjectType=0x7\nDataType=0x0005\nAccessType=rw\nDefaultValue=0xFF\nPDOMapping=0\n\n[1806sub3]\nParameterName=Inhibit Time\nObjectType=0x7\nDataType=0x0006\nAccessType=rw\nDefaultValue=0x0064\nPDOMapping=0\n\n[1806sub4]\nParameterName=Compatibility Entry\nObjectType=0x7\nDataType=0x0005\nAccessType=rw\nDefaultValue=0x00\nPDOMapping=0\n\n[1806sub5]\nParameterName=Event Timer\nObjectType=0x7\nDataType=0x0006\nAccessType=rw\nDefaultValue=0x0000\nPDOMapping=0\n\n[1806sub6]\nParameterName=SYNC start value\nObjectType=0x7\nDataType=0x0005\nAccessType=rw\nDefaultValue=0x00\nPDOMapping=0\n\n[1807]\nParameterName=Transmit PDO 8 Communication Parameter\nObjectType=0x9\nSubNumber=0x07\n\n[1807sub0]\nParameterName=Number of entries\nObjectType=0x7\nDataType=0x0005\nAccessType=ro\nDefaultValue=0x06\nPDOMapping=0\n\n[1807sub1]\nParameterName=COB-ID\nObjectType=0x7\nDataType=0x0007\nAccessType=rw\nDefaultValue=0xC0000000\nPDOMapping=0\n\n[1807sub2]\nParameterName=Transmission Type\nObjectType=0x7\nDataType=0x0005\nAccessType=rw\nDefaultValue=0xFF\nPDOMapping=0\n\n[1807sub3]\nParameterName=Inhibit Time\nObjectType=0x7\nDataType=0x0006\nAccessType=rw\nDefaultValue=0x0064\nPDOMapping=0\n\n[1807sub4]\nParameterName=Compatibility Entry\nObjectType=0x7\nDataType=0x0005\nAccessType=rw\nDefaultValue=0x00\nPDOMapping=0\n\n[1807sub5]\nParameterName=Event Timer\nObjectType=0x7\nDataType=0x0006\nAccessType=rw\nDefaultValue=0x0000\nPDOMapping=0\n\n[1807sub6]\nParameterName=SYNC start value\nObjectType=0x7\nDataType=0x0005\nAccessType=rw\nDefaultValue=0x00\nPDOMapping=0\n\n[1A00]\nParameterName=Transmit PDO 1 Mapping Parameter\nObjectType=0x9\nSubNumber=0x09\n\n[1A00sub0]\nParameterName=Number of entries\nObjectType=0x7\nDataType=0x0005\nAccessType=rw\nDefaultValue=0x02\nPDOMapping=0\n\n[1A00sub1]\nParameterName=1st object to be mapped\nObjectType=0x7\nDataType=0x0007\nAccessType=rw\nDefaultValue=0x60410010\nPDOMapping=0\n\n[1A00sub2]\nParameterName=2nd object to be mapped\nObjectType=0x7\nDataType=0x0007\nAccessType=rw\nDefaultValue=0x60610008\nPDOMapping=0\n\n[1A00sub3]\nParameterName=3rd object to be mapped\nObjectType=0x7\nDataType=0x0007\nAccessType=rw\nDefaultValue=0x00000000\nPDOMapping=0\n\n[1A00sub4]\nParameterName=4th object to be mapped\nObjectType=0x7\nDataType=0x0007\nAccessType=rw\nDefaultValue=0x00000000\nPDOMapping=0\n\n[1A00sub5]\nParameterName=5th object to be mapped\nObjectType=0x7\nDataType=0x0007\nAccessType=rw\nDefaultValue=0x00000000\nPDOMapping=0\n\n[1A00sub6]\nParameterName=6th object to be mapped\nObjectType=0x7\nDataType=0x0007\nAccessType=rw\nDefaultValue=0x00000000\nPDOMapping=0\n\n[1A00sub7]\nParameterName=7th object to be mapped\nObjectType=0x7\nDataType=0x0007\nAccessType=rw\nDefaultValue=0x00000000\nPDOMapping=0\n\n[1A00sub8]\nParameterName=8th object to be mapped\nObjectType=0x7\nDataType=0x0007\nAccessType=rw\nDefaultValue=0x00000000\nPDOMapping=0\n\n[1A01]\nParameterName=Transmit PDO 2 Mapping Parameter\nObjectType=0x9\nSubNumber=0x09\n\n[1A01sub0]\nParameterName=Number of entries\nObjectType=0x7\nDataType=0x0005\nAccessType=rw\nDefaultValue=0x01\nPDOMapping=0\n\n[1A01sub1]\nParameterName=1st object to be mapped\nObjectType=0x7\nDataType=0x0007\nAccessType=rw\nDefaultValue=0x60640020\nPDOMapping=0\n\n[1A01sub2]\nParameterName=2nd object to be mapped\nObjectType=0x7\nDataType=0x0007\nAccessType=rw\nDefaultValue=0x00000000\nPDOMapping=0\n\n[1A01sub3]\nParameterName=3rd object to be mapped\nObjectType=0x7\nDataType=0x0007\nAccessType=rw\nDefaultValue=0x00000000\nPDOMapping=0\n\n[1A01sub4]\nParameterName=4th object to be mapped\nObjectType=0x7\nDataType=0x0007\nAccessType=rw\nDefaultValue=0x00000000\nPDOMapping=0\n\n[1A01sub5]\nParameterName=5th object to be mapped\nObjectType=0x7\nDataType=0x0007\nAccessType=rw\nDefaultValue=0x00000000\nPDOMapping=0\n\n[1A01sub6]\nParameterName=6th object to be mapped\nObjectType=0x7\nDataType=0x0007\nAccessType=rw\nDefaultValue=0x00000000\nPDOMapping=0\n\n[1A01sub7]\nParameterName=7th object to be mapped\nObjectType=0x7\nDataType=0x0007\nAccessType=rw\nDefaultValue=0x00000000\nPDOMapping=0\n\n[1A01sub8]\nParameterName=8th object to be mapped\nObjectType=0x7\nDataType=0x0007\nAccessType=rw\nDefaultValue=0x00000000\nPDOMapping=0\n\n[1A02]\nParameterName=Transmit PDO 3 Mapping Parameter\nObjectType=0x9\nSubNumber=0x09\n\n[1A02sub0]\nParameterName=Number of entries\nObjectType=0x7\nDataType=0x0005\nAccessType=rw\nDefaultValue=0x01\nPDOMapping=0\n\n[1A02sub1]\nParameterName=1st object to be mapped\nObjectType=0x7\nDataType=0x0007\nAccessType=rw\nDefaultValue=0x60440010\nPDOMapping=0\n\n[1A02sub2]\nParameterName=2nd object to be mapped\nObjectType=0x7\nDataType=0x0007\nAccessType=rw\nDefaultValue=0x00000000\nPDOMapping=0\n\n[1A02sub3]\nParameterName=3rd object to be mapped\nObjectType=0x7\nDataType=0x0007\nAccessType=rw\nDefaultValue=0x00000000\nPDOMapping=0\n\n[1A02sub4]\nParameterName=4th object to be mapped\nObjectType=0x7\nDataType=0x0007\nAccessType=rw\nDefaultValue=0x00000000\nPDOMapping=0\n\n[1A02sub5]\nParameterName=5th object to be mapped\nObjectType=0x7\nDataType=0x0007\nAccessType=rw\nDefaultValue=0x00000000\nPDOMapping=0\n\n[1A02sub6]\nParameterName=6th object to be mapped\nObjectType=0x7\nDataType=0x0007\nAccessType=rw\nDefaultValue=0x00000000\nPDOMapping=0\n\n[1A02sub7]\nParameterName=7th object to be mapped\nObjectType=0x7\nDataType=0x0007\nAccessType=rw\nDefaultValue=0x00000000\nPDOMapping=0\n\n[1A02sub8]\nParameterName=8th object to be mapped\nObjectType=0x7\nDataType=0x0007\nAccessType=rw\nDefaultValue=0x00000000\nPDOMapping=0\n\n[1A03]\nParameterName=Transmit PDO 4 Mapping Parameter\nObjectType=0x9\nSubNumber=0x09\n\n[1A03sub0]\nParameterName=Number of entries\nObjectType=0x7\nDataType=0x0005\nAccessType=rw\nDefaultValue=0x01\nPDOMapping=0\n\n[1A03sub1]\nParameterName=1st object to be mapped\nObjectType=0x7\nDataType=0x0007\nAccessType=rw\nDefaultValue=0x60FD0020\nPDOMapping=0\n\n[1A03sub2]\nParameterName=2nd object to be mapped\nObjectType=0x7\nDataType=0x0007\nAccessType=rw\nDefaultValue=0x00000000\nPDOMapping=0\n\n[1A03sub3]\nParameterName=3rd object to be mapped\nObjectType=0x7\nDataType=0x0007\nAccessType=rw\nDefaultValue=0x00000000\nPDOMapping=0\n\n[1A03sub4]\nParameterName=4th object to be mapped\nObjectType=0x7\nDataType=0x0007\nAccessType=rw\nDefaultValue=0x00000000\nPDOMapping=0\n\n[1A03sub5]\nParameterName=5th object to be mapped\nObjectType=0x7\nDataType=0x0007\nAccessType=rw\nDefaultValue=0x00000000\nPDOMapping=0\n\n[1A03sub6]\nParameterName=6th object to be mapped\nObjectType=0x7\nDataType=0x0007\nAccessType=rw\nDefaultValue=0x00000000\nPDOMapping=0\n\n[1A03sub7]\nParameterName=7th object to be mapped\nObjectType=0x7\nDataType=0x0007\nAccessType=rw\nDefaultValue=0x00000000\nPDOMapping=0\n\n[1A03sub8]\nParameterName=8th object to be mapped\nObjectType=0x7\nDataType=0x0007\nAccessType=rw\nDefaultValue=0x00000000\nPDOMapping=0\n\n[1A04]\nParameterName=Transmit PDO 5 Mapping Parameter\nObjectType=0x9\nSubNumber=0x09\n\n[1A04sub0]\nParameterName=Number of entries\nObjectType=0x7\nDataType=0x0005\nAccessType=rw\nDefaultValue=0x00\nPDOMapping=0\n\n[1A04sub1]\nParameterName=1st object to be mapped\nObjectType=0x7\nDataType=0x0007\nAccessType=rw\nDefaultValue=0x00000000\nPDOMapping=0\n\n[1A04sub2]\nParameterName=2nd object to be mapped\nObjectType=0x7\nDataType=0x0007\nAccessType=rw\nDefaultValue=0x00000000\nPDOMapping=0\n\n[1A04sub3]\nParameterName=3rd object to be mapped\nObjectType=0x7\nDataType=0x0007\nAccessType=rw\nDefaultValue=0x00000000\nPDOMapping=0\n\n[1A04sub4]\nParameterName=4th object to be mapped\nObjectType=0x7\nDataType=0x0007\nAccessType=rw\nDefaultValue=0x00000000\nPDOMapping=0\n\n[1A04sub5]\nParameterName=5th object to be mapped\nObjectType=0x7\nDataType=0x0007\nAccessType=rw\nDefaultValue=0x00000000\nPDOMapping=0\n\n[1A04sub6]\nParameterName=6th object to be mapped\nObjectType=0x7\nDataType=0x0007\nAccessType=rw\nDefaultValue=0x00000000\nPDOMapping=0\n\n[1A04sub7]\nParameterName=7th object to be mapped\nObjectType=0x7\nDataType=0x0007\nAccessType=rw\nDefaultValue=0x00000000\nPDOMapping=0\n\n[1A04sub8]\nParameterName=8th object to be mapped\nObjectType=0x7\nDataType=0x0007\nAccessType=rw\nDefaultValue=0x00000000\nPDOMapping=0\n\n[1A05]\nParameterName=Transmit PDO 6 Mapping Parameter\nObjectType=0x9\nSubNumber=0x09\n\n[1A05sub0]\nParameterName=Number of entries\nObjectType=0x7\nDataType=0x0005\nAccessType=rw\nDefaultValue=0x00\nPDOMapping=0\n\n[1A05sub1]\nParameterName=1st object to be mapped\nObjectType=0x7\nDataType=0x0007\nAccessType=rw\nDefaultValue=0x00000000\nPDOMapping=0\n\n[1A05sub2]\nParameterName=2nd object to be mapped\nObjectType=0x7\nDataType=0x0007\nAccessType=rw\nDefaultValue=0x00000000\nPDOMapping=0\n\n[1A05sub3]\nParameterName=3rd object to be mapped\nObjectType=0x7\nDataType=0x0007\nAccessType=rw\nDefaultValue=0x00000000\nPDOMapping=0\n\n[1A05sub4]\nParameterName=4th object to be mapped\nObjectType=0x7\nDataType=0x0007\nAccessType=rw\nDefaultValue=0x00000000\nPDOMapping=0\n\n[1A05sub5]\nParameterName=5th object to be mapped\nObjectType=0x7\nDataType=0x0007\nAccessType=rw\nDefaultValue=0x00000000\nPDOMapping=0\n\n[1A05sub6]\nParameterName=6th object to be mapped\nObjectType=0x7\nDataType=0x0007\nAccessType=rw\nDefaultValue=0x00000000\nPDOMapping=0\n\n[1A05sub7]\nParameterName=7th object to be mapped\nObjectType=0x7\nDataType=0x0007\nAccessType=rw\nDefaultValue=0x00000000\nPDOMapping=0\n\n[1A05sub8]\nParameterName=8th object to be mapped\nObjectType=0x7\nDataType=0x0007\nAccessType=rw\nDefaultValue=0x00000000\nPDOMapping=0\n\n[1A06]\nParameterName=Transmit PDO 7 Mapping Parameter\nObjectType=0x9\nSubNumber=0x09\n\n[1A06sub0]\nParameterName=Number of entries\nObjectType=0x7\nDataType=0x0005\nAccessType=rw\nDefaultValue=0x00\nPDOMapping=0\n\n[1A06sub1]\nParameterName=1st object to be mapped\nObjectType=0x7\nDataType=0x0007\nAccessType=rw\nDefaultValue=0x00000000\nPDOMapping=0\n\n[1A06sub2]\nParameterName=2nd object to be mapped\nObjectType=0x7\nDataType=0x0007\nAccessType=rw\nDefaultValue=0x00000000\nPDOMapping=0\n\n[1A06sub3]\nParameterName=3rd object to be mapped\nObjectType=0x7\nDataType=0x0007\nAccessType=rw\nDefaultValue=0x00000000\nPDOMapping=0\n\n[1A06sub4]\nParameterName=4th object to be mapped\nObjectType=0x7\nDataType=0x0007\nAccessType=rw\nDefaultValue=0x00000000\nPDOMapping=0\n\n[1A06sub5]\nParameterName=5th object to be mapped\nObjectType=0x7\nDataType=0x0007\nAccessType=rw\nDefaultValue=0x00000000\nPDOMapping=0\n\n[1A06sub6]\nParameterName=6th object to be mapped\nObjectType=0x7\nDataType=0x0007\nAccessType=rw\nDefaultValue=0x00000000\nPDOMapping=0\n\n[1A06sub7]\nParameterName=7th object to be mapped\nObjectType=0x7\nDataType=0x0007\nAccessType=rw\nDefaultValue=0x00000000\nPDOMapping=0\n\n[1A06sub8]\nParameterName=8th object to be mapped\nObjectType=0x7\nDataType=0x0007\nAccessType=rw\nDefaultValue=0x00000000\nPDOMapping=0\n\n[1A07]\nParameterName=Transmit PDO 8 Mapping Parameter\nObjectType=0x9\nSubNumber=0x09\n\n[1A07sub0]\nParameterName=Number of entries\nObjectType=0x7\nDataType=0x0005\nAccessType=rw\nDefaultValue=0x00\nPDOMapping=0\n\n[1A07sub1]\nParameterName=1st object to be mapped\nObjectType=0x7\nDataType=0x0007\nAccessType=rw\nDefaultValue=0x00000000\nPDOMapping=0\n\n[1A07sub2]\nParameterName=2nd object to be mapped\nObjectType=0x7\nDataType=0x0007\nAccessType=rw\nDefaultValue=0x00000000\nPDOMapping=0\n\n[1A07sub3]\nParameterName=3rd object to be mapped\nObjectType=0x7\nDataType=0x0007\nAccessType=rw\nDefaultValue=0x00000000\nPDOMapping=0\n\n[1A07sub4]\nParameterName=4th object to be mapped\nObjectType=0x7\nDataType=0x0007\nAccessType=rw\nDefaultValue=0x00000000\nPDOMapping=0\n\n[1A07sub5]\nParameterName=5th object to be mapped\nObjectType=0x7\nDataType=0x0007\nAccessType=rw\nDefaultValue=0x00000000\nPDOMapping=0\n\n[1A07sub6]\nParameterName=6th object to be mapped\nObjectType=0x7\nDataType=0x0007\nAccessType=rw\nDefaultValue=0x00000000\nPDOMapping=0\n\n[1A07sub7]\nParameterName=7th object to be mapped\nObjectType=0x7\nDataType=0x0007\nAccessType=rw\nDefaultValue=0x00000000\nPDOMapping=0\n\n[1A07sub8]\nParameterName=8th object to be mapped\nObjectType=0x7\nDataType=0x0007\nAccessType=rw\nDefaultValue=0x00000000\nPDOMapping=0\n\n[1F50]\nParameterName=Program data\nObjectType=0x8\nSubNumber=0x03\n\n[1F50sub0]\nParameterName=Number of entries\nObjectType=0x7\nDataType=0x0005\nAccessType=ro\nDefaultValue=0x02\nPDOMapping=0\nObjFlags=1\n\n[1F50sub1]\nParameterName=Program data bootloader/firmware\nObjectType=0x7\nDataType=0x000F\nAccessType=rw\nDefaultValue=\nPDOMapping=0\nObjFlags=1\n\n[1F50sub2]\nParameterName=Program data NanoJ\nObjectType=0x7\nDataType=0x000F\nAccessType=rw\nDefaultValue=\nPDOMapping=0\nObjFlags=1\n\n[1F51]\nParameterName=Program control\nObjectType=0x8\nSubNumber=0x03\n\n[1F51sub0]\nParameterName=Number of entries\nObjectType=0x7\nDataType=0x0005\nAccessType=ro\nDefaultValue=0x02\nPDOMapping=0\nObjFlags=1\n\n[1F51sub1]\nParameterName=Program control bootloader/firmware\nObjectType=0x7\nDataType=0x0005\nAccessType=rw\nDefaultValue=0x00\nPDOMapping=0\nObjFlags=1\n\n[1F51sub2]\nParameterName=Program control NanoJ\nObjectType=0x7\nDataType=0x0005\nAccessType=rw\nDefaultValue=0x00\nPDOMapping=0\nObjFlags=1\n\n[1F57]\nParameterName=Program status\nObjectType=0x8\nSubNumber=0x03\n\n[1F57sub0]\nParameterName=Number of entries\nObjectType=0x7\nDataType=0x0005\nAccessType=ro\nDefaultValue=0x02\nPDOMapping=0\nObjFlags=1\n\n[1F57sub1]\nParameterName=Program status bootloader/firmware\nObjectType=0x7\nDataType=0x0007\nAccessType=ro\nDefaultValue=0x00000000\nPDOMapping=0\nObjFlags=1\n\n[1F57sub2]\nParameterName=Program status NanoJ\nObjectType=0x7\nDataType=0x0007\nAccessType=ro\nDefaultValue=0x00000000\nPDOMapping=0\nObjFlags=1\n\n[1F80]\nParameterName=NMT startup\nObjectType=0x7\nDataType=0x0007\nAccessType=rw\nDefaultValue=0x00000000\nPDOMapping=0\n\n[6007]\nParameterName=Abort connection option code\nObjectType=0x7\nDataType=0x0003\nAccessType=rw\nDefaultValue=0x0001\nPDOMapping=0\n\n[603F]\nParameterName=Error code\nObjectType=0x7\nDataType=0x0006\nAccessType=ro\nDefaultValue=\nPDOMapping=1\nObjFlags=1\n\n[6040]\nParameterName=Controlword\nObjectType=0x7\nDataType=0x0006\nAccessType=rww\nDefaultValue=0x0000\nPDOMapping=1\n\n[6041]\nParameterName=Statusword\nObjectType=0x7\nDataType=0x0006\nAccessType=ro\nDefaultValue=\nPDOMapping=1\nObjFlags=1\n\n[6042]\nParameterName=vl target velocity\nObjectType=0x7\nDataType=0x0003\nAccessType=rww\nDefaultValue=200\nPDOMapping=1\n\n[6043]\nParameterName=vl velocity demand\nObjectType=0x7\nDataType=0x0003\nAccessType=ro\nDefaultValue=0x0000\nPDOMapping=1\nObjFlags=1\n\n[6044]\nParameterName=vl velocity actual value\nObjectType=0x7\nDataType=0x0003\nAccessType=ro\nDefaultValue=0x0000\nPDOMapping=1\nObjFlags=1\n\n[6046]\nParameterName=vl velocity min max amount\nObjectType=0x8\nSubNumber=0x03\n\n[6046sub0]\nParameterName=Number of entries\nObjectType=0x7\nDataType=0x0005\nAccessType=const\nDefaultValue=2\nPDOMapping=0\n\n[6046sub1]\nParameterName=MinAmount\nObjectType=0x7\nDataType=0x0007\nAccessType=rww\nDefaultValue=0\nPDOMapping=1\n\n[6046sub2]\nParameterName=MaxAmount\nObjectType=0x7\nDataType=0x0007\nAccessType=rww\nDefaultValue=30000\nPDOMapping=1\n\n[6048]\nParameterName=vl velocity acceleration\nObjectType=0x9\nSubNumber=0x03\n\n[6048sub0]\nParameterName=Number of entries\nObjectType=0x7\nDataType=0x0005\nAccessType=const\nDefaultValue=2\nPDOMapping=0\n\n[6048sub1]\nParameterName=DeltaSpeed\nObjectType=0x7\nDataType=0x0007\nAccessType=rww\nDefaultValue=500\nPDOMapping=1\n\n[6048sub2]\nParameterName=DeltaTime\nObjectType=0x7\nDataType=0x0006\nAccessType=rww\nDefaultValue=1\nPDOMapping=1\n\n[6049]\nParameterName=vl velocity deceleration\nObjectType=0x9\nSubNumber=0x03\n\n[6049sub0]\nParameterName=Number of entries\nObjectType=0x7\nDataType=0x0005\nAccessType=const\nDefaultValue=2\nPDOMapping=0\n\n[6049sub1]\nParameterName=DeltaSpeed\nObjectType=0x7\nDataType=0x0007\nAccessType=rww\nDefaultValue=500\nPDOMapping=1\n\n[6049sub2]\nParameterName=DeltaTime\nObjectType=0x7\nDataType=0x0006\nAccessType=rww\nDefaultValue=1\nPDOMapping=1\n\n[604A]\nParameterName=vl velocity quick stop\nObjectType=0x9\nSubNumber=0x03\n\n[604Asub0]\nParameterName=Number of entries\nObjectType=0x7\nDataType=0x0005\nAccessType=const\nDefaultValue=2\nPDOMapping=0\n\n[604Asub1]\nParameterName=DeltaSpeed\nObjectType=0x7\nDataType=0x0007\nAccessType=rww\nDefaultValue=5000\nPDOMapping=1\n\n[604Asub2]\nParameterName=DeltaTime\nObjectType=0x7\nDataType=0x0006\nAccessType=rww\nDefaultValue=1\nPDOMapping=1\n\n[604C]\nParameterName=vl dimension factor\nObjectType=0x8\nSubNumber=0x03\n\n[604Csub0]\nParameterName=Number of entries\nObjectType=0x7\nDataType=0x0005\nAccessType=const\nDefaultValue=2\nPDOMapping=0\n\n[604Csub1]\nParameterName=vl dimension factor numerator\nObjectType=0x7\nDataType=0x0004\nAccessType=rww\nDefaultValue=1\nPDOMapping=1\n\n[604Csub2]\nParameterName=vl dimension factor denominator\nObjectType=0x7\nDataType=0x0004\nAccessType=rww\nDefaultValue=1\nPDOMapping=1\n\n[605A]\nParameterName=Quick stop option code\nObjectType=0x7\nDataType=0x0003\nAccessType=rw\nDefaultValue=2\nPDOMapping=0\n\n[605B]\nParameterName=Shutdown option code\nObjectType=0x7\nDataType=0x0003\nAccessType=rw\nDefaultValue=1\nPDOMapping=0\n\n[605C]\nParameterName=Disable option code\nObjectType=0x7\nDataType=0x0003\nAccessType=rw\nDefaultValue=1\nPDOMapping=0\n\n[605D]\nParameterName=Halt option code\nObjectType=0x7\nDataType=0x0003\nAccessType=rw\nDefaultValue=1\nPDOMapping=0\n\n[605E]\nParameterName=Fault option code\nObjectType=0x7\nDataType=0x0003\nAccessType=rw\nDefaultValue=2\nPDOMapping=0\n\n[6060]\nParameterName=Modes of operation\nObjectType=0x7\nDataType=0x0002\nAccessType=rww\nDefaultValue=0x00\nPDOMapping=1\n\n[6061]\nParameterName=Modes of operation display\nObjectType=0x7\nDataType=0x0002\nAccessType=ro\nDefaultValue=0x00\nPDOMapping=1\nObjFlags=1\n\n[6062]\nParameterName=Position demand value\nObjectType=0x7\nDataType=0x0004\nAccessType=ro\nDefaultValue=0x00000000\nPDOMapping=1\nObjFlags=1\n\n[6063]\nParameterName=Position actual internal value\nObjectType=0x7\nDataType=0x0004\nAccessType=ro\nDefaultValue=\nPDOMapping=1\nObjFlags=1\n\n[6064]\nParameterName=Position actual value\nObjectType=0x7\nDataType=0x0004\nAccessType=ro\nDefaultValue=\nPDOMapping=1\nObjFlags=1\n\n[6065]\nParameterName=Following error window\nObjectType=0x7\nDataType=0x0007\nAccessType=rww\nDefaultValue=256\nPDOMapping=1\n\n[6066]\nParameterName=Following error time out\nObjectType=0x7\nDataType=0x0006\nAccessType=rww\nDefaultValue=100\nPDOMapping=1\n\n[6067]\nParameterName=Position window\nObjectType=0x7\nDataType=0x0007\nAccessType=rww\nDefaultValue=10\nPDOMapping=1\n\n[6068]\nParameterName=Position window time\nObjectType=0x7\nDataType=0x0006\nAccessType=rww\nDefaultValue=100\nPDOMapping=1\n\n[606B]\nParameterName=Velocity demand value\nObjectType=0x7\nDataType=0x0004\nAccessType=ro\nDefaultValue=0x00000000\nPDOMapping=1\nObjFlags=1\n\n[606C]\nParameterName=Velocity actual value\nObjectType=0x7\nDataType=0x0004\nAccessType=ro\nDefaultValue=0x00000000\nPDOMapping=1\nObjFlags=1\n\n[606D]\nParameterName=Velocity window\nObjectType=0x7\nDataType=0x0006\nAccessType=rww\nDefaultValue=30\nPDOMapping=1\n\n[606E]\nParameterName=Velocity window time\nObjectType=0x7\nDataType=0x0006\nAccessType=rww\nDefaultValue=0x0000\nPDOMapping=1\n\n[606F]\nParameterName=Velocity threshold\nObjectType=0x7\nDataType=0x0006\nAccessType=rww\nDefaultValue=0x0000\nPDOMapping=1\n\n[6070]\nParameterName=Velocity threshold time\nObjectType=0x7\nDataType=0x0006\nAccessType=rww\nDefaultValue=0x0000\nPDOMapping=1\n\n[6071]\nParameterName=Target torque\nObjectType=0x7\nDataType=0x0003\nAccessType=rww\nDefaultValue=0x0000\nPDOMapping=1\n\n[6072]\nParameterName=Max torque\nObjectType=0x7\nDataType=0x0006\nAccessType=rww\nDefaultValue=0x0064\nPDOMapping=1\n\n[6073]\nParameterName=Max current\nObjectType=0x7\nDataType=0x0006\nAccessType=rww\nDefaultValue=0x03E8\nPDOMapping=1\n\n[6074]\nParameterName=Torque demand\nObjectType=0x7\nDataType=0x0003\nAccessType=ro\nDefaultValue=0x0000\nPDOMapping=1\nObjFlags=1\n\n[6075]\nParameterName=Motor rated current\nObjectType=0x7\nDataType=0x0007\nAccessType=rw\nDefaultValue=\nPDOMapping=0\n\n[6077]\nParameterName=Torque actual value\nObjectType=0x7\nDataType=0x0003\nAccessType=ro\nDefaultValue=0x0000\nPDOMapping=1\nObjFlags=1\n\n[607A]\nParameterName=Target Position\nObjectType=0x7\nDataType=0x0004\nAccessType=rww\nDefaultValue=4000\nPDOMapping=1\n\n[607B]\nParameterName=Position range limit\nObjectType=0x8\nSubNumber=0x03\n\n[607Bsub0]\nParameterName=Number of entries\nObjectType=0x7\nDataType=0x0005\nAccessType=const\nDefaultValue=0x02\nPDOMapping=0\n\n[607Bsub1]\nParameterName=Min position range limit\nObjectType=0x7\nDataType=0x0004\nAccessType=rww\nDefaultValue=0x00000000\nPDOMapping=1\n\n[607Bsub2]\nParameterName=Max position range limit\nObjectType=0x7\nDataType=0x0004\nAccessType=rww\nDefaultValue=0x00000000\nPDOMapping=1\n\n[607C]\nParameterName=Home offset\nObjectType=0x7\nDataType=0x0004\nAccessType=rww\nDefaultValue=0x00000000\nPDOMapping=1\n\n[607D]\nParameterName=Software position limit\nObjectType=0x8\nSubNumber=0x03\n\n[607Dsub0]\nParameterName=Number of entries\nObjectType=0x7\nDataType=0x0005\nAccessType=const\nDefaultValue=0x02\nPDOMapping=0\n\n[607Dsub1]\nParameterName=Min position limit\nObjectType=0x7\nDataType=0x0004\nAccessType=rww\nDefaultValue=0x00000000\nPDOMapping=1\n\n[607Dsub2]\nParameterName=Max position limit\nObjectType=0x7\nDataType=0x0004\nAccessType=rww\nDefaultValue=0x00000000\nPDOMapping=1\n\n[607E]\nParameterName=Polarity\nObjectType=0x7\nDataType=0x0005\nAccessType=rww\nDefaultValue=0x00\nPDOMapping=1\n\n[607F]\nParameterName=Max profile velocity\nObjectType=0x7\nDataType=0x0007\nAccessType=rww\nDefaultValue=30000\nPDOMapping=1\n\n[6080]\nParameterName=Max motor speed\nObjectType=0x7\nDataType=0x0007\nAccessType=rww\nDefaultValue=30000\nPDOMapping=1\n\n[6081]\nParameterName=Profile velocity\nObjectType=0x7\nDataType=0x0007\nAccessType=rww\nDefaultValue=500\nPDOMapping=1\n\n[6082]\nParameterName=End velocity\nObjectType=0x7\nDataType=0x0007\nAccessType=rww\nDefaultValue=0\nPDOMapping=1\n\n[6083]\nParameterName=Profile acceleration\nObjectType=0x7\nDataType=0x0007\nAccessType=rww\nDefaultValue=500\nPDOMapping=1\n\n[6084]\nParameterName=Profile deceleration\nObjectType=0x7\nDataType=0x0007\nAccessType=rww\nDefaultValue=500\nPDOMapping=1\n\n[6085]\nParameterName=Quick stop deceleration\nObjectType=0x7\nDataType=0x0007\nAccessType=rww\nDefaultValue=5000\nPDOMapping=1\n\n[6086]\nParameterName=Motion profile type\nObjectType=0x7\nDataType=0x0003\nAccessType=rww\nDefaultValue=0x0000\nPDOMapping=1\n\n[6087]\nParameterName=Torque slope\nObjectType=0x7\nDataType=0x0007\nAccessType=rww\nDefaultValue=0x00000064\nPDOMapping=1\n\n[608F]\nParameterName=Position encoder resolution\nObjectType=0x8\nSubNumber=0x03\n\n[608Fsub0]\nParameterName=Number of entries\nObjectType=0x7\nDataType=0x0005\nAccessType=const\nDefaultValue=2\nPDOMapping=0\n\n[608Fsub1]\nParameterName=Encoder increments\nObjectType=0x7\nDataType=0x0004\nAccessType=rww\nDefaultValue=\nPDOMapping=1\n\n[608Fsub2]\nParameterName=Motor revolutions\nObjectType=0x7\nDataType=0x0004\nAccessType=rww\nDefaultValue=1\nPDOMapping=1\n\n[6090]\nParameterName=Velocity encoder resolution\nObjectType=0x8\nSubNumber=0x03\n\n[6090sub0]\nParameterName=Number of entries\nObjectType=0x7\nDataType=0x0005\nAccessType=const\nDefaultValue=2\nPDOMapping=0\n\n[6090sub1]\nParameterName=Encoder increments per second\nObjectType=0x7\nDataType=0x0004\nAccessType=rww\nDefaultValue=\nPDOMapping=1\n\n[6090sub2]\nParameterName=Motor revolutions per second\nObjectType=0x7\nDataType=0x0004\nAccessType=rww\nDefaultValue=1\nPDOMapping=1\n\n[6091]\nParameterName=Gear ratio\nObjectType=0x8\nSubNumber=0x03\n\n[6091sub0]\nParameterName=Number of entries\nObjectType=0x7\nDataType=0x0005\nAccessType=const\nDefaultValue=2\nPDOMapping=0\n\n[6091sub1]\nParameterName=Motor revolutions\nObjectType=0x7\nDataType=0x0007\nAccessType=rww\nDefaultValue=1\nPDOMapping=1\n\n[6091sub2]\nParameterName=Shaft revolutions\nObjectType=0x7\nDataType=0x0007\nAccessType=rww\nDefaultValue=1\nPDOMapping=1\n\n[6092]\nParameterName=Feed constant\nObjectType=0x8\nSubNumber=0x03\n\n[6092sub0]\nParameterName=Number of entries\nObjectType=0x7\nDataType=0x0005\nAccessType=const\nDefaultValue=2\nPDOMapping=0\n\n[6092sub1]\nParameterName=Feed\nObjectType=0x7\nDataType=0x0007\nAccessType=rww\nDefaultValue=1\nPDOMapping=1\n\n[6092sub2]\nParameterName=Shaft revolutions\nObjectType=0x7\nDataType=0x0007\nAccessType=rww\nDefaultValue=1\nPDOMapping=1\n\n[6096]\nParameterName=Velocity factor\nObjectType=0x8\nSubNumber=0x03\n\n[6096sub0]\nParameterName=Number of entries\nObjectType=0x7\nDataType=0x0005\nAccessType=const\nDefaultValue=2\nPDOMapping=0\n\n[6096sub1]\nParameterName=Numerator\nObjectType=0x7\nDataType=0x0007\nAccessType=rww\nDefaultValue=1\nPDOMapping=1\n\n[6096sub2]\nParameterName=Divisor\nObjectType=0x7\nDataType=0x0007\nAccessType=rww\nDefaultValue=1\nPDOMapping=1\n\n[6097]\nParameterName=Acceleration factor\nObjectType=0x8\nSubNumber=0x03\n\n[6097sub0]\nParameterName=Number of entries\nObjectType=0x7\nDataType=0x0005\nAccessType=const\nDefaultValue=2\nPDOMapping=0\n\n[6097sub1]\nParameterName=Numerator\nObjectType=0x7\nDataType=0x0007\nAccessType=rww\nDefaultValue=1\nPDOMapping=1\n\n[6097sub2]\nParameterName=Divisor\nObjectType=0x7\nDataType=0x0007\nAccessType=rww\nDefaultValue=1\nPDOMapping=1\n\n[6098]\nParameterName=Homing method\nObjectType=0x7\nDataType=0x0002\nAccessType=rww\nDefaultValue=35\nPDOMapping=1\n\n[6099]\nParameterName=Homing speed\nObjectType=0x8\nSubNumber=0x03\n\n[6099sub0]\nParameterName=Number of entries\nObjectType=0x7\nDataType=0x0005\nAccessType=const\nDefaultValue=2\nPDOMapping=0\n\n[6099sub1]\nParameterName=Speed during search for switch\nObjectType=0x7\nDataType=0x0007\nAccessType=rww\nDefaultValue=50\nPDOMapping=1\n\n[6099sub2]\nParameterName=Speed during search for zero\nObjectType=0x7\nDataType=0x0007\nAccessType=rww\nDefaultValue=10\nPDOMapping=1\n\n[609A]\nParameterName=Homing acceleration\nObjectType=0x7\nDataType=0x0007\nAccessType=rww\nDefaultValue=500\nPDOMapping=1\n\n[60A2]\nParameterName=Jerk factor\nObjectType=0x8\nSubNumber=0x03\n\n[60A2sub0]\nParameterName=Number of entries\nObjectType=0x7\nDataType=0x0005\nAccessType=const\nDefaultValue=2\nPDOMapping=0\n\n[60A2sub1]\nParameterName=Numerator\nObjectType=0x7\nDataType=0x0007\nAccessType=rww\nDefaultValue=1\nPDOMapping=1\n\n[60A2sub2]\nParameterName=Divisor\nObjectType=0x7\nDataType=0x0007\nAccessType=rww\nDefaultValue=1\nPDOMapping=1\n\n[60A4]\nParameterName=Profile Jerk\nObjectType=0x8\nSubNumber=0x05\n\n[60A4sub0]\nParameterName=Number of entries\nObjectType=0x7\nDataType=0x0005\nAccessType=const\nDefaultValue=4\nPDOMapping=0\n\n[60A4sub1]\nParameterName=Begin Acceleration Jerk\nObjectType=0x7\nDataType=0x0007\nAccessType=rw\nDefaultValue=1000\nPDOMapping=0\n\n[60A4sub2]\nParameterName=Begin Deceleration Jerk\nObjectType=0x7\nDataType=0x0007\nAccessType=rw\nDefaultValue=1000\nPDOMapping=0\n\n[60A4sub3]\nParameterName=End Acceleration Jerk\nObjectType=0x7\nDataType=0x0007\nAccessType=rw\nDefaultValue=1000\nPDOMapping=0\n\n[60A4sub4]\nParameterName=End Deceleration Jerk\nObjectType=0x7\nDataType=0x0007\nAccessType=rw\nDefaultValue=1000\nPDOMapping=0\n\n[60A8]\nParameterName=SI unit position\nObjectType=0x7\nDataType=0x0007\nAccessType=rw\nDefaultValue=0xFF410000\nPDOMapping=0\n\n[60A9]\nParameterName=SI unit velocity\nObjectType=0x7\nDataType=0x0007\nAccessType=rw\nDefaultValue=0x00B44700\nPDOMapping=0\n\n[60B0]\nParameterName=Position offset\nObjectType=0x7\nDataType=0x0004\nAccessType=rww\nDefaultValue=0x00000000\nPDOMapping=1\n\n[60B1]\nParameterName=Velocity offset\nObjectType=0x7\nDataType=0x0004\nAccessType=rww\nDefaultValue=0x00000000\nPDOMapping=1\n\n[60B2]\nParameterName=Torque offset\nObjectType=0x7\nDataType=0x0003\nAccessType=rww\nDefaultValue=0x0000\nPDOMapping=1\n\n[60C1]\nParameterName=Interpolation data record\nObjectType=0x8\nSubNumber=0x02\n\n[60C1sub0]\nParameterName=Number of entries\nObjectType=0x7\nDataType=0x0005\nAccessType=const\nDefaultValue=1\nPDOMapping=0\n\n[60C1sub1]\nParameterName=1st set-point\nObjectType=0x7\nDataType=0x0004\nAccessType=rww\nDefaultValue=0\nPDOMapping=1\n\n[60C2]\nParameterName=Interpolation time period\nObjectType=0x9\nSubNumber=0x03\n\n[60C2sub0]\nParameterName=Number of entries\nObjectType=0x7\nDataType=0x0005\nAccessType=const\nDefaultValue=2\nPDOMapping=0\n\n[60C2sub1]\nParameterName=Interpolation time period value\nObjectType=0x7\nDataType=0x0005\nAccessType=rw\nDefaultValue=1\nPDOMapping=0\n\n[60C2sub2]\nParameterName=Interpolation time index\nObjectType=0x7\nDataType=0x0002\nAccessType=rw\nDefaultValue=-3\nPDOMapping=0\n\n[60C4]\nParameterName=Interpolation data configuration\nObjectType=0x9\nSubNumber=0x07\n\n[60C4sub0]\nParameterName=Number of entries\nObjectType=0x7\nDataType=0x0005\nAccessType=const\nDefaultValue=6\nPDOMapping=0\n\n[60C4sub1]\nParameterName=MaximumBufferSize\nObjectType=0x7\nDataType=0x0007\nAccessType=ro\nDefaultValue=1\nPDOMapping=0\n\n[60C4sub2]\nParameterName=ActualBufferSize\nObjectType=0x7\nDataType=0x0007\nAccessType=rw\nDefaultValue=1\nPDOMapping=0\n\n[60C4sub3]\nParameterName=BufferOrganization\nObjectType=0x7\nDataType=0x0005\nAccessType=rw\nDefaultValue=0\nPDOMapping=0\n\n[60C4sub4]\nParameterName=BufferPosition\nObjectType=0x7\nDataType=0x0006\nAccessType=rw\nDefaultValue=1\nPDOMapping=0\n\n[60C4sub5]\nParameterName=SizeOfDataRecord\nObjectType=0x7\nDataType=0x0005\nAccessType=wo\nDefaultValue=4\nPDOMapping=0\n\n[60C4sub6]\nParameterName=BufferClear\nObjectType=0x7\nDataType=0x0005\nAccessType=wo\nDefaultValue=0\nPDOMapping=0\n\n[60C5]\nParameterName=Max acceleration\nObjectType=0x7\nDataType=0x0007\nAccessType=rww\nDefaultValue=5000\nPDOMapping=1\n\n[60C6]\nParameterName=Max deceleration\nObjectType=0x7\nDataType=0x0007\nAccessType=rww\nDefaultValue=5000\nPDOMapping=1\n\n[60E4]\nParameterName=Additional position actual value\nObjectType=0x8\nSubNumber=0x04\n\n[60E4sub0]\nParameterName=Number of entries\nObjectType=0x7\nDataType=0x0005\nAccessType=ro\nDefaultValue=3\nPDOMapping=1\nObjFlags=1\n\n[60E4sub1]\nParameterName=Additional position actual value #1\nObjectType=0x7\nDataType=0x0004\nAccessType=ro\nDefaultValue=0\nPDOMapping=1\nObjFlags=1\n\n[60E4sub2]\nParameterName=Additional position actual value #2\nObjectType=0x7\nDataType=0x0004\nAccessType=ro\nDefaultValue=0\nPDOMapping=1\nObjFlags=1\n\n[60E4sub3]\nParameterName=Additional position actual value #3\nObjectType=0x7\nDataType=0x0004\nAccessType=ro\nDefaultValue=0\nPDOMapping=1\nObjFlags=1\n\n[60E5]\nParameterName=Additional velocity actual value\nObjectType=0x8\nSubNumber=0x04\n\n[60E5sub0]\nParameterName=Number of entries\nObjectType=0x7\nDataType=0x0005\nAccessType=ro\nDefaultValue=3\nPDOMapping=1\nObjFlags=1\n\n[60E5sub1]\nParameterName=Additional velocity actual value #1\nObjectType=0x7\nDataType=0x0004\nAccessType=ro\nDefaultValue=0\nPDOMapping=1\nObjFlags=1\n\n[60E5sub2]\nParameterName=Additional velocity actual value #2\nObjectType=0x7\nDataType=0x0004\nAccessType=ro\nDefaultValue=0\nPDOMapping=1\nObjFlags=1\n\n[60E5sub3]\nParameterName=Additional velocity actual value #3\nObjectType=0x7\nDataType=0x0004\nAccessType=ro\nDefaultValue=0\nPDOMapping=1\nObjFlags=1\n\n[60E6]\nParameterName=Additional position encoder resolution - encoder increments\nObjectType=0x8\nSubNumber=0x04\n\n[60E6sub0]\nParameterName=Number of entries\nObjectType=0x7\nDataType=0x0005\nAccessType=ro\nDefaultValue=3\nPDOMapping=1\n\n[60E6sub1]\nParameterName=Additional position encoder resolution - encoder increments feedback interface #1\nObjectType=0x7\nDataType=0x0004\nAccessType=rww\nDefaultValue=\nPDOMapping=1\n\n[60E6sub2]\nParameterName=Additional position encoder resolution - encoder increments feedback interface #2\nObjectType=0x7\nDataType=0x0004\nAccessType=rww\nDefaultValue=\nPDOMapping=1\n\n[60E6sub3]\nParameterName=Additional position encoder resolution - encoder increments feedback interface #3\nObjectType=0x7\nDataType=0x0004\nAccessType=rww\nDefaultValue=0\nPDOMapping=1\n\n[60E8]\nParameterName=Additional gear ratio - motor shaft revolutions\nObjectType=0x8\nSubNumber=0x04\n\n[60E8sub0]\nParameterName=Number of entries\nObjectType=0x7\nDataType=0x0005\nAccessType=ro\nDefaultValue=3\nPDOMapping=1\n\n[60E8sub1]\nParameterName=Additional gear ratio - motor shaft revolutions feedback interface #1\nObjectType=0x7\nDataType=0x0007\nAccessType=rww\nDefaultValue=1\nPDOMapping=1\n\n[60E8sub2]\nParameterName=Additional gear ratio - motor shaft revolutions feedback interface #2\nObjectType=0x7\nDataType=0x0007\nAccessType=rww\nDefaultValue=1\nPDOMapping=1\n\n[60E8sub3]\nParameterName=Additional gear ratio - motor shaft revolutions feedback interface #3\nObjectType=0x7\nDataType=0x0007\nAccessType=rww\nDefaultValue=1\nPDOMapping=1\n\n[60E9]\nParameterName=Additional feed constant - feed\nObjectType=0x8\nSubNumber=0x04\n\n[60E9sub0]\nParameterName=Number of entries\nObjectType=0x7\nDataType=0x0005\nAccessType=ro\nDefaultValue=3\nPDOMapping=1\n\n[60E9sub1]\nParameterName=Additional feed constant - feed feedback interface #1\nObjectType=0x7\nDataType=0x0007\nAccessType=rww\nDefaultValue=1\nPDOMapping=1\n\n[60E9sub2]\nParameterName=Additional feed constant - feed feedback interface #2\nObjectType=0x7\nDataType=0x0007\nAccessType=rww\nDefaultValue=1\nPDOMapping=1\n\n[60E9sub3]\nParameterName=Additional feed constant - feed feedback interface #3\nObjectType=0x7\nDataType=0x0007\nAccessType=rww\nDefaultValue=1\nPDOMapping=1\n\n[60EB]\nParameterName=Additional position encoder resolution - motor revolutions\nObjectType=0x8\nSubNumber=0x04\n\n[60EBsub0]\nParameterName=Number of entries\nObjectType=0x7\nDataType=0x0005\nAccessType=ro\nDefaultValue=3\nPDOMapping=1\n\n[60EBsub1]\nParameterName=Additional position encoder resolution - motor revolutions feedback interface #1\nObjectType=0x7\nDataType=0x0007\nAccessType=rww\nDefaultValue=1\nPDOMapping=1\n\n[60EBsub2]\nParameterName=Additional position encoder resolution - motor revolutions feedback interface #2\nObjectType=0x7\nDataType=0x0007\nAccessType=rww\nDefaultValue=1\nPDOMapping=1\n\n[60EBsub3]\nParameterName=Additional position encoder resolution - motor revolutions feedback interface #3\nObjectType=0x7\nDataType=0x0007\nAccessType=rww\nDefaultValue=1\nPDOMapping=1\n\n[60ED]\nParameterName=Additional gear ratio - driving shaft revolutions\nObjectType=0x8\nSubNumber=0x04\n\n[60EDsub0]\nParameterName=Number of entries\nObjectType=0x7\nDataType=0x0005\nAccessType=ro\nDefaultValue=3\nPDOMapping=1\n\n[60EDsub1]\nParameterName=Additional gear ratio - driving shaft revolutions feedback interface #1\nObjectType=0x7\nDataType=0x0007\nAccessType=rww\nDefaultValue=1\nPDOMapping=1\n\n[60EDsub2]\nParameterName=Additional gear ratio - driving shaft revolutions feedback interface #2\nObjectType=0x7\nDataType=0x0007\nAccessType=rww\nDefaultValue=1\nPDOMapping=1\n\n[60EDsub3]\nParameterName=Additional gear ratio - driving shaft revolutions feedback interface #3\nObjectType=0x7\nDataType=0x0007\nAccessType=rww\nDefaultValue=1\nPDOMapping=1\n\n[60EE]\nParameterName=Additional feed constant - driving shaft revolutions\nObjectType=0x8\nSubNumber=0x04\n\n[60EEsub0]\nParameterName=Number of entries\nObjectType=0x7\nDataType=0x0005\nAccessType=ro\nDefaultValue=3\nPDOMapping=1\n\n[60EEsub1]\nParameterName=Additional feed constant - driving shaft revolutions feedback interface #1\nObjectType=0x7\nDataType=0x0007\nAccessType=rww\nDefaultValue=1\nPDOMapping=1\n\n[60EEsub2]\nParameterName=Additional feed constant - driving shaft revolutions feedback interface #2\nObjectType=0x7\nDataType=0x0007\nAccessType=rww\nDefaultValue=1\nPDOMapping=1\n\n[60EEsub3]\nParameterName=Additional feed constant - driving shaft revolutions feedback interface #3\nObjectType=0x7\nDataType=0x0007\nAccessType=rww\nDefaultValue=1\nPDOMapping=1\n\n[60F2]\nParameterName=Positioning option code\nObjectType=0x7\nDataType=0x0006\nAccessType=rww\nDefaultValue=1\nPDOMapping=1\n\n[60F4]\nParameterName=Following error actual value\nObjectType=0x7\nDataType=0x0004\nAccessType=ro\nDefaultValue=0x00000000\nPDOMapping=1\nObjFlags=1\n\n[60F8]\nParameterName=Max slippage\nObjectType=0x7\nDataType=0x0004\nAccessType=rww\nDefaultValue=0x00000190\nPDOMapping=1\n\n[60FA]\nParameterName=Control Effort\nObjectType=0x7\nDataType=0x0004\nAccessType=ro\nDefaultValue=\nPDOMapping=1\nObjFlags=1\n\n[60FC]\nParameterName=Position demand internal value\nObjectType=0x7\nDataType=0x0004\nAccessType=ro\nDefaultValue=\nPDOMapping=1\nObjFlags=1\n\n[60FD]\nParameterName=Digital Inputs\nObjectType=0x7\nDataType=0x0007\nAccessType=ro\nDefaultValue=0x00000000\nPDOMapping=1\nObjFlags=1\n\n[60FE]\nParameterName=Digital Outputs\nObjectType=0x8\nSubNumber=0x02\n\n[60FEsub0]\nParameterName=Number of entries\nObjectType=0x7\nDataType=0x0005\nAccessType=const\nDefaultValue=0x01\nPDOMapping=0\n\n[60FEsub1]\nParameterName=Physical outputs\nObjectType=0x7\nDataType=0x0007\nAccessType=rww\nDefaultValue=0x00000001\nPDOMapping=1\n\n[60FF]\nParameterName=Target velocity\nObjectType=0x7\nDataType=0x0004\nAccessType=rww\nDefaultValue=0x00000000\nPDOMapping=1\n\n[6502]\nParameterName=Supported drive modes\nObjectType=0x7\nDataType=0x0007\nAccessType=ro\nDefaultValue=0x000003EF\nPDOMapping=1\nObjFlags=1\n\n[6503]\nParameterName=Drive catalogue number\nObjectType=0x7\nDataType=0x0009\nAccessType=const\nDefaultValue=\nPDOMapping=0\nObjFlags=1\n\n[6505]\nParameterName=http drive catalogue address\nObjectType=0x7\nDataType=0x0009\nAccessType=const\nDefaultValue=\nPDOMapping=0\nObjFlags=1\n\n[ManufacturerObjects]\nSupportedObjects=0x4F\n1=0x2005\n2=0x2007\n3=0x2009\n4=0x2030\n5=0x2031\n6=0x2034\n7=0x2035\n8=0x2036\n9=0x2037\n10=0x2038\n11=0x2039\n12=0x203A\n13=0x203B\n14=0x203D\n15=0x203E\n16=0x203F\n17=0x2057\n18=0x2058\n19=0x2059\n20=0x205A\n21=0x205B\n22=0x2084\n23=0x2101\n24=0x2102\n25=0x2103\n26=0x2290\n27=0x2291\n28=0x2292\n29=0x2300\n30=0x2301\n31=0x2302\n32=0x230E\n33=0x230F\n34=0x2310\n35=0x2320\n36=0x2330\n37=0x2400\n38=0x2410\n39=0x2500\n40=0x2600\n41=0x2701\n42=0x2800\n43=0x3202\n44=0x3203\n45=0x3204\n46=0x320D\n47=0x3210\n48=0x3212\n49=0x321A\n50=0x321B\n51=0x321C\n52=0x321D\n53=0x321E\n54=0x3220\n55=0x3221\n56=0x3225\n57=0x3240\n58=0x3242\n59=0x3243\n60=0x3250\n61=0x3252\n62=0x3320\n63=0x3321\n64=0x3322\n65=0x3323\n66=0x3380\n67=0x3390\n68=0x33A0\n69=0x3502\n70=0x3602\n71=0x3700\n72=0x3701\n73=0x4012\n74=0x4013\n75=0x4014\n76=0x4021\n77=0x4040\n78=0x4041\n79=0x4042\n\n[2005]\nParameterName=CANopen Baudrate\nObjectType=0x7\nDataType=0x0005\nAccessType=rw\nDefaultValue=136\nPDOMapping=0\n\n[2007]\nParameterName=CANopen Config\nObjectType=0x8\nSubNumber=0x02\n\n[2007sub0]\nParameterName=Number of entries\nObjectType=0x7\nDataType=0x0005\nAccessType=const\nDefaultValue=0x01\nPDOMapping=0\n\n[2007sub1]\nParameterName=BL Config\nObjectType=0x7\nDataType=0x0007\nAccessType=rw\nDefaultValue=0x00000000\nPDOMapping=0\n\n[2009]\nParameterName=CANopen NodeID\nObjectType=0x7\nDataType=0x0005\nAccessType=rw\nDefaultValue=0x7F\nPDOMapping=0\n\n[2030]\nParameterName=Pole pair count\nObjectType=0x7\nDataType=0x0007\nAccessType=rw\nDefaultValue=50\nPDOMapping=0\n\n[2031]\nParameterName=Max motor current\nObjectType=0x7\nDataType=0x0007\nAccessType=rw\nDefaultValue=1000\nPDOMapping=0\n\n[2034]\nParameterName=Upper voltage warning level\nObjectType=0x7\nDataType=0x0007\nAccessType=rw\nDefaultValue=49677\nPDOMapping=0\n\n[2035]\nParameterName=Lower voltage warning level\nObjectType=0x7\nDataType=0x0007\nAccessType=rw\nDefaultValue=10000\nPDOMapping=0\n\n[2036]\nParameterName=Open loop current reduction idle time\nObjectType=0x7\nDataType=0x0007\nAccessType=rw\nDefaultValue=1000\nPDOMapping=0\n\n[2037]\nParameterName=Open loop current reduction value/factor\nObjectType=0x7\nDataType=0x0004\nAccessType=rw\nDefaultValue=-50\nPDOMapping=0\n\n[2038]\nParameterName=Brake controller timing\nObjectType=0x8\nSubNumber=0x07\n\n[2038sub0]\nParameterName=Number of entries\nObjectType=0x7\nDataType=0x0005\nAccessType=ro\nDefaultValue=6\nPDOMapping=0\n\n[2038sub1]\nParameterName=Close Brake idle time\nObjectType=0x7\nDataType=0x0007\nAccessType=rw\nDefaultValue=1000\nPDOMapping=0\n\n[2038sub2]\nParameterName=Shutdown power idle time\nObjectType=0x7\nDataType=0x0007\nAccessType=rw\nDefaultValue=1000\nPDOMapping=0\n\n[2038sub3]\nParameterName=Open Brake delay time\nObjectType=0x7\nDataType=0x0007\nAccessType=rw\nDefaultValue=1000\nPDOMapping=0\n\n[2038sub4]\nParameterName=Start Operation delay time\nObjectType=0x7\nDataType=0x0007\nAccessType=rw\nDefaultValue=0\nPDOMapping=0\n\n[2038sub5]\nParameterName=PWM frequency\nObjectType=0x7\nDataType=0x0007\nAccessType=rw\nDefaultValue=0\nPDOMapping=0\n\n[2038sub6]\nParameterName=PWM duty cycle\nObjectType=0x7\nDataType=0x0007\nAccessType=rw\nDefaultValue=0\nPDOMapping=0\n\n[2039]\nParameterName=Motor Currents\nObjectType=0x8\nSubNumber=0x06\n\n[2039sub0]\nParameterName=Number of entries\nObjectType=0x7\nDataType=0x0005\nAccessType=ro\nDefaultValue=0x05\nPDOMapping=0\nObjFlags=1\n\n[2039sub1]\nParameterName=Id\nObjectType=0x7\nDataType=0x0004\nAccessType=ro\nDefaultValue=\nPDOMapping=1\nObjFlags=1\n\n[2039sub2]\nParameterName=Iq\nObjectType=0x7\nDataType=0x0004\nAccessType=ro\nDefaultValue=\nPDOMapping=1\nObjFlags=1\n\n[2039sub3]\nParameterName=I?\nObjectType=0x7\nDataType=0x0004\nAccessType=ro\nDefaultValue=\nPDOMapping=1\nObjFlags=1\n\n[2039sub4]\nParameterName=I?\nObjectType=0x7\nDataType=0x0004\nAccessType=ro\nDefaultValue=\nPDOMapping=1\nObjFlags=1\n\n[2039sub5]\nParameterName=Actual current\nObjectType=0x7\nDataType=0x0004\nAccessType=ro\nDefaultValue=0x00000000\nPDOMapping=1\nObjFlags=1\n\n[203A]\nParameterName=Homing on block configuration\nObjectType=0x8\nSubNumber=0x03\n\n[203Asub0]\nParameterName=Number of entries\nObjectType=0x7\nDataType=0x0005\nAccessType=ro\nDefaultValue=2\nPDOMapping=0\n\n[203Asub1]\nParameterName=Minimum current for block detection\nObjectType=0x7\nDataType=0x0004\nAccessType=rw\nDefaultValue=2500\nPDOMapping=0\n\n[203Asub2]\nParameterName=Block detection time\nObjectType=0x7\nDataType=0x0004\nAccessType=rw\nDefaultValue=200\nPDOMapping=0\n\n[203B]\nParameterName=I2t Parameters\nObjectType=0x8\nSubNumber=0x07\n\n[203Bsub0]\nParameterName=Number of entries\nObjectType=0x7\nDataType=0x0005\nAccessType=ro\nDefaultValue=6\nPDOMapping=0\n\n[203Bsub1]\nParameterName=Motor rated current\nObjectType=0x7\nDataType=0x0007\nAccessType=rw\nDefaultValue=1000\nPDOMapping=0\n\n[203Bsub2]\nParameterName=Maximum duration of max current\nObjectType=0x7\nDataType=0x0007\nAccessType=rw\nDefaultValue=0\nPDOMapping=0\n\n[203Bsub3]\nParameterName=Threshold\nObjectType=0x7\nDataType=0x0007\nAccessType=rw\nDefaultValue=0\nPDOMapping=0\n\n[203Bsub4]\nParameterName=CalcValue\nObjectType=0x7\nDataType=0x0007\nAccessType=rw\nDefaultValue=0\nPDOMapping=0\n\n[203Bsub5]\nParameterName=LimitedCurrent\nObjectType=0x7\nDataType=0x0007\nAccessType=rw\nDefaultValue=\nPDOMapping=0\n\n[203Bsub6]\nParameterName=Status\nObjectType=0x7\nDataType=0x0007\nAccessType=rw\nDefaultValue=0\nPDOMapping=0\n\n[203D]\nParameterName=Torque window\nObjectType=0x7\nDataType=0x0006\nAccessType=rww\nDefaultValue=0x0000\nPDOMapping=1\n\n[203E]\nParameterName=Torque window time out\nObjectType=0x7\nDataType=0x0006\nAccessType=rww\nDefaultValue=0x0000\nPDOMapping=1\n\n[203F]\nParameterName=Max slippage time out\nObjectType=0x7\nDataType=0x0006\nAccessType=rww\nDefaultValue=0x0064\nPDOMapping=1\n\n[2057]\nParameterName=Clock Direction Multiplier\nObjectType=0x7\nDataType=0x0004\nAccessType=rw\nDefaultValue=128\nPDOMapping=0\n\n[2058]\nParameterName=Clock Direction Divider\nObjectType=0x7\nDataType=0x0004\nAccessType=rw\nDefaultValue=1\nPDOMapping=0\n\n[2059]\nParameterName=Encoder Configuration\nObjectType=0x7\nDataType=0x0007\nAccessType=rw\nDefaultValue=0x00000000\nPDOMapping=0\n\n[205A]\nParameterName=Absolute Sensor Boot Value (in user units)\nObjectType=0x7\nDataType=0x0004\nAccessType=ro\nDefaultValue=\nPDOMapping=0\nObjFlags=1\n\n[205B]\nParameterName=Clock Direction or Clockwise/Counter Clockwise Mode\nObjectType=0x7\nDataType=0x0007\nAccessType=rw\nDefaultValue=0x00000000\nPDOMapping=0\n\n[2084]\nParameterName=Bootup Delay\nObjectType=0x7\nDataType=0x0007\nAccessType=rw\nDefaultValue=0\nPDOMapping=0\n\n[2101]\nParameterName=Fieldbus Module Availability\nObjectType=0x7\nDataType=0x0007\nAccessType=ro\nDefaultValue=0x00190009\nPDOMapping=0\nObjFlags=1\n\n[2102]\nParameterName=Fieldbus Module Control\nObjectType=0x7\nDataType=0x0007\nAccessType=rw\nDefaultValue=0x00190009\nPDOMapping=0\n\n[2103]\nParameterName=Fieldbus Module Status\nObjectType=0x8\nSubNumber=0x03\n\n[2103sub0]\nParameterName=Number of entries\nObjectType=0x7\nDataType=0x0005\nAccessType=ro\nDefaultValue=0x02\nPDOMapping=0\nObjFlags=1\n\n[2103sub1]\nParameterName=Fieldbus Module Disable Mask\nObjectType=0x7\nDataType=0x0007\nAccessType=ro\nDefaultValue=0x00000008\nPDOMapping=0\nObjFlags=1\n\n[2103sub2]\nParameterName=Fieldbus Module Enabled\nObjectType=0x7\nDataType=0x0007\nAccessType=ro\nDefaultValue=\nPDOMapping=0\nObjFlags=1\n\n[2290]\nParameterName=PDI Control\nObjectType=0x7\nDataType=0x0005\nAccessType=rw\nDefaultValue=0x01\nPDOMapping=0\n\n[2291]\nParameterName=PDI Input\nObjectType=0x9\nSubNumber=0x05\n\n[2291sub0]\nParameterName=Number of entries\nObjectType=0x7\nDataType=0x0005\nAccessType=ro\nDefaultValue=4\nPDOMapping=1\nObjFlags=1\n\n[2291sub1]\nParameterName=PDI Set Value 1\nObjectType=0x7\nDataType=0x0004\nAccessType=rww\nDefaultValue=0\nPDOMapping=1\nObjFlags=1\n\n[2291sub2]\nParameterName=PDI Set Value 2\nObjectType=0x7\nDataType=0x0003\nAccessType=rww\nDefaultValue=0\nPDOMapping=1\nObjFlags=1\n\n[2291sub3]\nParameterName=PDI Set Value 3\nObjectType=0x7\nDataType=0x0002\nAccessType=rww\nDefaultValue=0\nPDOMapping=1\nObjFlags=1\n\n[2291sub4]\nParameterName=PDI Command\nObjectType=0x7\nDataType=0x0002\nAccessType=rww\nDefaultValue=0\nPDOMapping=1\nObjFlags=1\n\n[2292]\nParameterName=PDI Output\nObjectType=0x9\nSubNumber=0x03\n\n[2292sub0]\nParameterName=Number of entries\nObjectType=0x7\nDataType=0x0005\nAccessType=ro\nDefaultValue=2\nPDOMapping=1\nObjFlags=1\n\n[2292sub1]\nParameterName=PDI Status\nObjectType=0x7\nDataType=0x0003\nAccessType=ro\nDefaultValue=0\nPDOMapping=1\nObjFlags=1\n\n[2292sub2]\nParameterName=PDI Return Value\nObjectType=0x7\nDataType=0x0004\nAccessType=ro\nDefaultValue=0\nPDOMapping=1\nObjFlags=1\n\n[2300]\nParameterName=NanoJ Control\nObjectType=0x7\nDataType=0x0007\nAccessType=rww\nDefaultValue=0x00000000\nPDOMapping=1\n\n[2301]\nParameterName=NanoJ Status\nObjectType=0x7\nDataType=0x0007\nAccessType=ro\nDefaultValue=0x00000000\nPDOMapping=1\nObjFlags=1\n\n[2302]\nParameterName=NanoJ Error Code\nObjectType=0x7\nDataType=0x0007\nAccessType=ro\nDefaultValue=0x00000000\nPDOMapping=1\nObjFlags=1\n\n[230E]\nParameterName=Timer\nObjectType=0x8\nSubNumber=0x02\n\n[230Esub0]\nParameterName=Number of entries\nObjectType=0x7\nDataType=0x0005\nAccessType=ro\nDefaultValue=0x01\nPDOMapping=0\nObjFlags=1\n\n[230Esub1]\nParameterName=1ms Timer\nObjectType=0x7\nDataType=0x0007\nAccessType=ro\nDefaultValue=\nPDOMapping=0\nObjFlags=1\n\n[230F]\nParameterName=Uptime Seconds\nObjectType=0x7\nDataType=0x0007\nAccessType=ro\nDefaultValue=\nPDOMapping=1\nObjFlags=1\n\n[2310]\nParameterName=NanoJ input data selection\nObjectType=0x8\nSubNumber=0x11\n\n[2310sub0]\nParameterName=Number of entries\nObjectType=0x7\nDataType=0x0005\nAccessType=ro\nDefaultValue=0x10\nPDOMapping=0\nObjFlags=1\n\n[2310sub1]\nParameterName=Mapping #1\nObjectType=0x7\nDataType=0x0007\nAccessType=ro\nDefaultValue=0x00000000\nPDOMapping=0\nObjFlags=1\n\n[2310sub2]\nParameterName=Mapping #2\nObjectType=0x7\nDataType=0x0007\nAccessType=ro\nDefaultValue=0x00000000\nPDOMapping=0\nObjFlags=1\n\n[2310sub3]\nParameterName=Mapping #3\nObjectType=0x7\nDataType=0x0007\nAccessType=ro\nDefaultValue=0x00000000\nPDOMapping=0\nObjFlags=1\n\n[2310sub4]\nParameterName=Mapping #4\nObjectType=0x7\nDataType=0x0007\nAccessType=ro\nDefaultValue=0x00000000\nPDOMapping=0\nObjFlags=1\n\n[2310sub5]\nParameterName=Mapping #5\nObjectType=0x7\nDataType=0x0007\nAccessType=ro\nDefaultValue=0x00000000\nPDOMapping=0\nObjFlags=1\n\n[2310sub6]\nParameterName=Mapping #6\nObjectType=0x7\nDataType=0x0007\nAccessType=ro\nDefaultValue=0x00000000\nPDOMapping=0\nObjFlags=1\n\n[2310sub7]\nParameterName=Mapping #7\nObjectType=0x7\nDataType=0x0007\nAccessType=ro\nDefaultValue=0x00000000\nPDOMapping=0\nObjFlags=1\n\n[2310sub8]\nParameterName=Mapping #8\nObjectType=0x7\nDataType=0x0007\nAccessType=ro\nDefaultValue=0x00000000\nPDOMapping=0\nObjFlags=1\n\n[2310sub9]\nParameterName=Mapping #9\nObjectType=0x7\nDataType=0x0007\nAccessType=ro\nDefaultValue=0x00000000\nPDOMapping=0\nObjFlags=1\n\n[2310subA]\nParameterName=Mapping #10\nObjectType=0x7\nDataType=0x0007\nAccessType=ro\nDefaultValue=0x00000000\nPDOMapping=0\nObjFlags=1\n\n[2310subB]\nParameterName=Mapping #11\nObjectType=0x7\nDataType=0x0007\nAccessType=ro\nDefaultValue=0x00000000\nPDOMapping=0\nObjFlags=1\n\n[2310subC]\nParameterName=Mapping #12\nObjectType=0x7\nDataType=0x0007\nAccessType=ro\nDefaultValue=0x00000000\nPDOMapping=0\nObjFlags=1\n\n[2310subD]\nParameterName=Mapping #13\nObjectType=0x7\nDataType=0x0007\nAccessType=ro\nDefaultValue=0x00000000\nPDOMapping=0\nObjFlags=1\n\n[2310subE]\nParameterName=Mapping #14\nObjectType=0x7\nDataType=0x0007\nAccessType=ro\nDefaultValue=0x00000000\nPDOMapping=0\nObjFlags=1\n\n[2310subF]\nParameterName=Mapping #15\nObjectType=0x7\nDataType=0x0007\nAccessType=ro\nDefaultValue=0x00000000\nPDOMapping=0\nObjFlags=1\n\n[2310sub10]\nParameterName=Mapping #16\nObjectType=0x7\nDataType=0x0007\nAccessType=ro\nDefaultValue=0x00000000\nPDOMapping=0\nObjFlags=1\n\n[2320]\nParameterName=NanoJ output data selection\nObjectType=0x8\nSubNumber=0x11\n\n[2320sub0]\nParameterName=Number of entries\nObjectType=0x7\nDataType=0x0005\nAccessType=ro\nDefaultValue=0x10\nPDOMapping=0\nObjFlags=1\n\n[2320sub1]\nParameterName=Mapping #1\nObjectType=0x7\nDataType=0x0007\nAccessType=ro\nDefaultValue=0x00000000\nPDOMapping=0\nObjFlags=1\n\n[2320sub2]\nParameterName=Mapping #2\nObjectType=0x7\nDataType=0x0007\nAccessType=ro\nDefaultValue=0x00000000\nPDOMapping=0\nObjFlags=1\n\n[2320sub3]\nParameterName=Mapping #3\nObjectType=0x7\nDataType=0x0007\nAccessType=ro\nDefaultValue=0x00000000\nPDOMapping=0\nObjFlags=1\n\n[2320sub4]\nParameterName=Mapping #4\nObjectType=0x7\nDataType=0x0007\nAccessType=ro\nDefaultValue=0x00000000\nPDOMapping=0\nObjFlags=1\n\n[2320sub5]\nParameterName=Mapping #5\nObjectType=0x7\nDataType=0x0007\nAccessType=ro\nDefaultValue=0x00000000\nPDOMapping=0\nObjFlags=1\n\n[2320sub6]\nParameterName=Mapping #6\nObjectType=0x7\nDataType=0x0007\nAccessType=ro\nDefaultValue=0x00000000\nPDOMapping=0\nObjFlags=1\n\n[2320sub7]\nParameterName=Mapping #7\nObjectType=0x7\nDataType=0x0007\nAccessType=ro\nDefaultValue=0x00000000\nPDOMapping=0\nObjFlags=1\n\n[2320sub8]\nParameterName=Mapping #8\nObjectType=0x7\nDataType=0x0007\nAccessType=ro\nDefaultValue=0x00000000\nPDOMapping=0\nObjFlags=1\n\n[2320sub9]\nParameterName=Mapping #9\nObjectType=0x7\nDataType=0x0007\nAccessType=ro\nDefaultValue=0x00000000\nPDOMapping=0\nObjFlags=1\n\n[2320subA]\nParameterName=Mapping #10\nObjectType=0x7\nDataType=0x0007\nAccessType=ro\nDefaultValue=0x00000000\nPDOMapping=0\nObjFlags=1\n\n[2320subB]\nParameterName=Mapping #11\nObjectType=0x7\nDataType=0x0007\nAccessType=ro\nDefaultValue=0x00000000\nPDOMapping=0\nObjFlags=1\n\n[2320subC]\nParameterName=Mapping #12\nObjectType=0x7\nDataType=0x0007\nAccessType=ro\nDefaultValue=0x00000000\nPDOMapping=0\nObjFlags=1\n\n[2320subD]\nParameterName=Mapping #13\nObjectType=0x7\nDataType=0x0007\nAccessType=ro\nDefaultValue=0x00000000\nPDOMapping=0\nObjFlags=1\n\n[2320subE]\nParameterName=Mapping #14\nObjectType=0x7\nDataType=0x0007\nAccessType=ro\nDefaultValue=0x00000000\nPDOMapping=0\nObjFlags=1\n\n[2320subF]\nParameterName=Mapping #15\nObjectType=0x7\nDataType=0x0007\nAccessType=ro\nDefaultValue=0x00000000\nPDOMapping=0\nObjFlags=1\n\n[2320sub10]\nParameterName=Mapping #16\nObjectType=0x7\nDataType=0x0007\nAccessType=ro\nDefaultValue=0x00000000\nPDOMapping=0\nObjFlags=1\n\n[2330]\nParameterName=NanoJ in/output data selection\nObjectType=0x8\nSubNumber=0x11\n\n[2330sub0]\nParameterName=Number of entries\nObjectType=0x7\nDataType=0x0005\nAccessType=ro\nDefaultValue=0x10\nPDOMapping=0\nObjFlags=1\n\n[2330sub1]\nParameterName=Mapping #1\nObjectType=0x7\nDataType=0x0007\nAccessType=ro\nDefaultValue=0x00000000\nPDOMapping=0\nObjFlags=1\n\n[2330sub2]\nParameterName=Mapping #2\nObjectType=0x7\nDataType=0x0007\nAccessType=ro\nDefaultValue=0x00000000\nPDOMapping=0\nObjFlags=1\n\n[2330sub3]\nParameterName=Mapping #3\nObjectType=0x7\nDataType=0x0007\nAccessType=ro\nDefaultValue=0x00000000\nPDOMapping=0\nObjFlags=1\n\n[2330sub4]\nParameterName=Mapping #4\nObjectType=0x7\nDataType=0x0007\nAccessType=ro\nDefaultValue=0x00000000\nPDOMapping=0\nObjFlags=1\n\n[2330sub5]\nParameterName=Mapping #5\nObjectType=0x7\nDataType=0x0007\nAccessType=ro\nDefaultValue=0x00000000\nPDOMapping=0\nObjFlags=1\n\n[2330sub6]\nParameterName=Mapping #6\nObjectType=0x7\nDataType=0x0007\nAccessType=ro\nDefaultValue=0x00000000\nPDOMapping=0\nObjFlags=1\n\n[2330sub7]\nParameterName=Mapping #7\nObjectType=0x7\nDataType=0x0007\nAccessType=ro\nDefaultValue=0x00000000\nPDOMapping=0\nObjFlags=1\n\n[2330sub8]\nParameterName=Mapping #8\nObjectType=0x7\nDataType=0x0007\nAccessType=ro\nDefaultValue=0x00000000\nPDOMapping=0\nObjFlags=1\n\n[2330sub9]\nParameterName=Mapping #9\nObjectType=0x7\nDataType=0x0007\nAccessType=ro\nDefaultValue=0x00000000\nPDOMapping=0\nObjFlags=1\n\n[2330subA]\nParameterName=Mapping #10\nObjectType=0x7\nDataType=0x0007\nAccessType=ro\nDefaultValue=0x00000000\nPDOMapping=0\nObjFlags=1\n\n[2330subB]\nParameterName=Mapping #11\nObjectType=0x7\nDataType=0x0007\nAccessType=ro\nDefaultValue=0x00000000\nPDOMapping=0\nObjFlags=1\n\n[2330subC]\nParameterName=Mapping #12\nObjectType=0x7\nDataType=0x0007\nAccessType=ro\nDefaultValue=0x00000000\nPDOMapping=0\nObjFlags=1\n\n[2330subD]\nParameterName=Mapping #13\nObjectType=0x7\nDataType=0x0007\nAccessType=ro\nDefaultValue=0x00000000\nPDOMapping=0\nObjFlags=1\n\n[2330subE]\nParameterName=Mapping #14\nObjectType=0x7\nDataType=0x0007\nAccessType=ro\nDefaultValue=0x00000000\nPDOMapping=0\nObjFlags=1\n\n[2330subF]\nParameterName=Mapping #15\nObjectType=0x7\nDataType=0x0007\nAccessType=ro\nDefaultValue=0x00000000\nPDOMapping=0\nObjFlags=1\n\n[2330sub10]\nParameterName=Mapping #16\nObjectType=0x7\nDataType=0x0007\nAccessType=ro\nDefaultValue=0x00000000\nPDOMapping=0\nObjFlags=1\n\n[2400]\nParameterName=NanoJ Inputs\nObjectType=0x8\nSubNumber=0x21\n\n[2400sub0]\nParameterName=Number of entries\nObjectType=0x7\nDataType=0x0005\nAccessType=ro\nDefaultValue=0x20\nPDOMapping=0\nObjFlags=1\n\n[2400sub1]\nParameterName=NanoJ Input #1\nObjectType=0x7\nDataType=0x0004\nAccessType=rww\nDefaultValue=0x00000000\nPDOMapping=1\nObjFlags=1\n\n[2400sub2]\nParameterName=NanoJ Input #2\nObjectType=0x7\nDataType=0x0004\nAccessType=rww\nDefaultValue=0x00000000\nPDOMapping=1\nObjFlags=1\n\n[2400sub3]\nParameterName=NanoJ Input #3\nObjectType=0x7\nDataType=0x0004\nAccessType=rww\nDefaultValue=0x00000000\nPDOMapping=1\nObjFlags=1\n\n[2400sub4]\nParameterName=NanoJ Input #4\nObjectType=0x7\nDataType=0x0004\nAccessType=rww\nDefaultValue=0x00000000\nPDOMapping=1\nObjFlags=1\n\n[2400sub5]\nParameterName=NanoJ Input #5\nObjectType=0x7\nDataType=0x0004\nAccessType=rww\nDefaultValue=0x00000000\nPDOMapping=1\nObjFlags=1\n\n[2400sub6]\nParameterName=NanoJ Input #6\nObjectType=0x7\nDataType=0x0004\nAccessType=rww\nDefaultValue=0x00000000\nPDOMapping=1\nObjFlags=1\n\n[2400sub7]\nParameterName=NanoJ Input #7\nObjectType=0x7\nDataType=0x0004\nAccessType=rww\nDefaultValue=0x00000000\nPDOMapping=1\nObjFlags=1\n\n[2400sub8]\nParameterName=NanoJ Input #8\nObjectType=0x7\nDataType=0x0004\nAccessType=rww\nDefaultValue=0x00000000\nPDOMapping=1\nObjFlags=1\n\n[2400sub9]\nParameterName=NanoJ Input #9\nObjectType=0x7\nDataType=0x0004\nAccessType=rww\nDefaultValue=0x00000000\nPDOMapping=1\nObjFlags=1\n\n[2400subA]\nParameterName=NanoJ Input #10\nObjectType=0x7\nDataType=0x0004\nAccessType=rww\nDefaultValue=0x00000000\nPDOMapping=1\nObjFlags=1\n\n[2400subB]\nParameterName=NanoJ Input #11\nObjectType=0x7\nDataType=0x0004\nAccessType=rww\nDefaultValue=0x00000000\nPDOMapping=1\nObjFlags=1\n\n[2400subC]\nParameterName=NanoJ Input #12\nObjectType=0x7\nDataType=0x0004\nAccessType=rww\nDefaultValue=0x00000000\nPDOMapping=1\nObjFlags=1\n\n[2400subD]\nParameterName=NanoJ Input #13\nObjectType=0x7\nDataType=0x0004\nAccessType=rww\nDefaultValue=0x00000000\nPDOMapping=1\nObjFlags=1\n\n[2400subE]\nParameterName=NanoJ Input #14\nObjectType=0x7\nDataType=0x0004\nAccessType=rww\nDefaultValue=0x00000000\nPDOMapping=1\nObjFlags=1\n\n[2400subF]\nParameterName=NanoJ Input #15\nObjectType=0x7\nDataType=0x0004\nAccessType=rww\nDefaultValue=0x00000000\nPDOMapping=1\nObjFlags=1\n\n[2400sub10]\nParameterName=NanoJ Input #16\nObjectType=0x7\nDataType=0x0004\nAccessType=rww\nDefaultValue=0x00000000\nPDOMapping=1\nObjFlags=1\n\n[2400sub11]\nParameterName=NanoJ Input #17\nObjectType=0x7\nDataType=0x0004\nAccessType=rww\nDefaultValue=0x00000000\nPDOMapping=1\nObjFlags=1\n\n[2400sub12]\nParameterName=NanoJ Input #18\nObjectType=0x7\nDataType=0x0004\nAccessType=rww\nDefaultValue=0x00000000\nPDOMapping=1\nObjFlags=1\n\n[2400sub13]\nParameterName=NanoJ Input #19\nObjectType=0x7\nDataType=0x0004\nAccessType=rww\nDefaultValue=0x00000000\nPDOMapping=1\nObjFlags=1\n\n[2400sub14]\nParameterName=NanoJ Input #20\nObjectType=0x7\nDataType=0x0004\nAccessType=rww\nDefaultValue=0x00000000\nPDOMapping=1\nObjFlags=1\n\n[2400sub15]\nParameterName=NanoJ Input #21\nObjectType=0x7\nDataType=0x0004\nAccessType=rww\nDefaultValue=0x00000000\nPDOMapping=1\nObjFlags=1\n\n[2400sub16]\nParameterName=NanoJ Input #22\nObjectType=0x7\nDataType=0x0004\nAccessType=rww\nDefaultValue=0x00000000\nPDOMapping=1\nObjFlags=1\n\n[2400sub17]\nParameterName=NanoJ Input #23\nObjectType=0x7\nDataType=0x0004\nAccessType=rww\nDefaultValue=0x00000000\nPDOMapping=1\nObjFlags=1\n\n[2400sub18]\nParameterName=NanoJ Input #24\nObjectType=0x7\nDataType=0x0004\nAccessType=rww\nDefaultValue=0x00000000\nPDOMapping=1\nObjFlags=1\n\n[2400sub19]\nParameterName=NanoJ Input #25\nObjectType=0x7\nDataType=0x0004\nAccessType=rww\nDefaultValue=0x00000000\nPDOMapping=1\nObjFlags=1\n\n[2400sub1A]\nParameterName=NanoJ Input #26\nObjectType=0x7\nDataType=0x0004\nAccessType=rww\nDefaultValue=0x00000000\nPDOMapping=1\nObjFlags=1\n\n[2400sub1B]\nParameterName=NanoJ Input #27\nObjectType=0x7\nDataType=0x0004\nAccessType=rww\nDefaultValue=0x00000000\nPDOMapping=1\nObjFlags=1\n\n[2400sub1C]\nParameterName=NanoJ Input #28\nObjectType=0x7\nDataType=0x0004\nAccessType=rww\nDefaultValue=0x00000000\nPDOMapping=1\nObjFlags=1\n\n[2400sub1D]\nParameterName=NanoJ Input #29\nObjectType=0x7\nDataType=0x0004\nAccessType=rww\nDefaultValue=0x00000000\nPDOMapping=1\nObjFlags=1\n\n[2400sub1E]\nParameterName=NanoJ Input #30\nObjectType=0x7\nDataType=0x0004\nAccessType=rww\nDefaultValue=0x00000000\nPDOMapping=1\nObjFlags=1\n\n[2400sub1F]\nParameterName=NanoJ Input #31\nObjectType=0x7\nDataType=0x0004\nAccessType=rww\nDefaultValue=0x00000000\nPDOMapping=1\nObjFlags=1\n\n[2400sub20]\nParameterName=NanoJ Input #32\nObjectType=0x7\nDataType=0x0004\nAccessType=rww\nDefaultValue=0x00000000\nPDOMapping=1\nObjFlags=1\n\n[2410]\nParameterName=NanoJ Init Parameters\nObjectType=0x8\nSubNumber=0x21\n\n[2410sub0]\nParameterName=Number of entries\nObjectType=0x7\nDataType=0x0005\nAccessType=ro\nDefaultValue=0x20\nPDOMapping=0\n\n[2410sub1]\nParameterName=NanoJ Init Parameter #1\nObjectType=0x7\nDataType=0x0004\nAccessType=rww\nDefaultValue=0x00000000\nPDOMapping=1\n\n[2410sub2]\nParameterName=NanoJ Init Parameter #2\nObjectType=0x7\nDataType=0x0004\nAccessType=rww\nDefaultValue=0x00000000\nPDOMapping=1\n\n[2410sub3]\nParameterName=NanoJ Init Parameter #3\nObjectType=0x7\nDataType=0x0004\nAccessType=rww\nDefaultValue=0x00000000\nPDOMapping=1\n\n[2410sub4]\nParameterName=NanoJ Init Parameter #4\nObjectType=0x7\nDataType=0x0004\nAccessType=rww\nDefaultValue=0x00000000\nPDOMapping=1\n\n[2410sub5]\nParameterName=NanoJ Init Parameter #5\nObjectType=0x7\nDataType=0x0004\nAccessType=rww\nDefaultValue=0x00000000\nPDOMapping=1\n\n[2410sub6]\nParameterName=NanoJ Init Parameter #6\nObjectType=0x7\nDataType=0x0004\nAccessType=rww\nDefaultValue=0x00000000\nPDOMapping=1\n\n[2410sub7]\nParameterName=NanoJ Init Parameter #7\nObjectType=0x7\nDataType=0x0004\nAccessType=rww\nDefaultValue=0x00000000\nPDOMapping=1\n\n[2410sub8]\nParameterName=NanoJ Init Parameter #8\nObjectType=0x7\nDataType=0x0004\nAccessType=rww\nDefaultValue=0x00000000\nPDOMapping=1\n\n[2410sub9]\nParameterName=NanoJ Init Parameter #9\nObjectType=0x7\nDataType=0x0004\nAccessType=rww\nDefaultValue=0x00000000\nPDOMapping=1\n\n[2410subA]\nParameterName=NanoJ Init Parameter #10\nObjectType=0x7\nDataType=0x0004\nAccessType=rww\nDefaultValue=0x00000000\nPDOMapping=1\n\n[2410subB]\nParameterName=NanoJ Init Parameter #11\nObjectType=0x7\nDataType=0x0004\nAccessType=rww\nDefaultValue=0x00000000\nPDOMapping=1\n\n[2410subC]\nParameterName=NanoJ Init Parameter #12\nObjectType=0x7\nDataType=0x0004\nAccessType=rww\nDefaultValue=0x00000000\nPDOMapping=1\n\n[2410subD]\nParameterName=NanoJ Init Parameter #13\nObjectType=0x7\nDataType=0x0004\nAccessType=rww\nDefaultValue=0x00000000\nPDOMapping=1\n\n[2410subE]\nParameterName=NanoJ Init Parameter #14\nObjectType=0x7\nDataType=0x0004\nAccessType=rww\nDefaultValue=0x00000000\nPDOMapping=1\n\n[2410subF]\nParameterName=NanoJ Init Parameter #15\nObjectType=0x7\nDataType=0x0004\nAccessType=rww\nDefaultValue=0x00000000\nPDOMapping=1\n\n[2410sub10]\nParameterName=NanoJ Init Parameter #16\nObjectType=0x7\nDataType=0x0004\nAccessType=rww\nDefaultValue=0x00000000\nPDOMapping=1\n\n[2410sub11]\nParameterName=NanoJ Init Parameter #17\nObjectType=0x7\nDataType=0x0004\nAccessType=rww\nDefaultValue=0x00000000\nPDOMapping=1\n\n[2410sub12]\nParameterName=NanoJ Init Parameter #18\nObjectType=0x7\nDataType=0x0004\nAccessType=rww\nDefaultValue=0x00000000\nPDOMapping=1\n\n[2410sub13]\nParameterName=NanoJ Init Parameter #19\nObjectType=0x7\nDataType=0x0004\nAccessType=rww\nDefaultValue=0x00000000\nPDOMapping=1\n\n[2410sub14]\nParameterName=NanoJ Init Parameter #20\nObjectType=0x7\nDataType=0x0004\nAccessType=rww\nDefaultValue=0x00000000\nPDOMapping=1\n\n[2410sub15]\nParameterName=NanoJ Init Parameter #21\nObjectType=0x7\nDataType=0x0004\nAccessType=rww\nDefaultValue=0x00000000\nPDOMapping=1\n\n[2410sub16]\nParameterName=NanoJ Init Parameter #22\nObjectType=0x7\nDataType=0x0004\nAccessType=rww\nDefaultValue=0x00000000\nPDOMapping=1\n\n[2410sub17]\nParameterName=NanoJ Init Parameter #23\nObjectType=0x7\nDataType=0x0004\nAccessType=rww\nDefaultValue=0x00000000\nPDOMapping=1\n\n[2410sub18]\nParameterName=NanoJ Init Parameter #24\nObjectType=0x7\nDataType=0x0004\nAccessType=rww\nDefaultValue=0x00000000\nPDOMapping=1\n\n[2410sub19]\nParameterName=NanoJ Init Parameter #25\nObjectType=0x7\nDataType=0x0004\nAccessType=rww\nDefaultValue=0x00000000\nPDOMapping=1\n\n[2410sub1A]\nParameterName=NanoJ Init Parameter #26\nObjectType=0x7\nDataType=0x0004\nAccessType=rww\nDefaultValue=0x00000000\nPDOMapping=1\n\n[2410sub1B]\nParameterName=NanoJ Init Parameter #27\nObjectType=0x7\nDataType=0x0004\nAccessType=rww\nDefaultValue=0x00000000\nPDOMapping=1\n\n[2410sub1C]\nParameterName=NanoJ Init Parameter #28\nObjectType=0x7\nDataType=0x0004\nAccessType=rww\nDefaultValue=0x00000000\nPDOMapping=1\n\n[2410sub1D]\nParameterName=NanoJ Init Parameter #29\nObjectType=0x7\nDataType=0x0004\nAccessType=rww\nDefaultValue=0x00000000\nPDOMapping=1\n\n[2410sub1E]\nParameterName=NanoJ Init Parameter #30\nObjectType=0x7\nDataType=0x0004\nAccessType=rww\nDefaultValue=0x00000000\nPDOMapping=1\n\n[2410sub1F]\nParameterName=NanoJ Init Parameter #31\nObjectType=0x7\nDataType=0x0004\nAccessType=rww\nDefaultValue=0x00000000\nPDOMapping=1\n\n[2410sub20]\nParameterName=NanoJ Init Parameter #32\nObjectType=0x7\nDataType=0x0004\nAccessType=rww\nDefaultValue=0x00000000\nPDOMapping=1\n\n[2500]\nParameterName=NanoJ Outputs\nObjectType=0x8\nSubNumber=0x21\n\n[2500sub0]\nParameterName=Number of entries\nObjectType=0x7\nDataType=0x0005\nAccessType=ro\nDefaultValue=0x20\nPDOMapping=0\nObjFlags=1\n\n[2500sub1]\nParameterName=NanoJ Output #1\nObjectType=0x7\nDataType=0x0004\nAccessType=rwr\nDefaultValue=0x00000000\nPDOMapping=1\nObjFlags=1\n\n[2500sub2]\nParameterName=NanoJ Output #2\nObjectType=0x7\nDataType=0x0004\nAccessType=rwr\nDefaultValue=0x00000000\nPDOMapping=1\nObjFlags=1\n\n[2500sub3]\nParameterName=NanoJ Output #3\nObjectType=0x7\nDataType=0x0004\nAccessType=rwr\nDefaultValue=0x00000000\nPDOMapping=1\nObjFlags=1\n\n[2500sub4]\nParameterName=NanoJ Output #4\nObjectType=0x7\nDataType=0x0004\nAccessType=rwr\nDefaultValue=0x00000000\nPDOMapping=1\nObjFlags=1\n\n[2500sub5]\nParameterName=NanoJ Output #5\nObjectType=0x7\nDataType=0x0004\nAccessType=rwr\nDefaultValue=0x00000000\nPDOMapping=1\nObjFlags=1\n\n[2500sub6]\nParameterName=NanoJ Output #6\nObjectType=0x7\nDataType=0x0004\nAccessType=rwr\nDefaultValue=0x00000000\nPDOMapping=1\nObjFlags=1\n\n[2500sub7]\nParameterName=NanoJ Output #7\nObjectType=0x7\nDataType=0x0004\nAccessType=rwr\nDefaultValue=0x00000000\nPDOMapping=1\nObjFlags=1\n\n[2500sub8]\nParameterName=NanoJ Output #8\nObjectType=0x7\nDataType=0x0004\nAccessType=rwr\nDefaultValue=0x00000000\nPDOMapping=1\nObjFlags=1\n\n[2500sub9]\nParameterName=NanoJ Output #9\nObjectType=0x7\nDataType=0x0004\nAccessType=rwr\nDefaultValue=0x00000000\nPDOMapping=1\nObjFlags=1\n\n[2500subA]\nParameterName=NanoJ Output #10\nObjectType=0x7\nDataType=0x0004\nAccessType=rwr\nDefaultValue=0x00000000\nPDOMapping=1\nObjFlags=1\n\n[2500subB]\nParameterName=NanoJ Output #11\nObjectType=0x7\nDataType=0x0004\nAccessType=rwr\nDefaultValue=0x00000000\nPDOMapping=1\nObjFlags=1\n\n[2500subC]\nParameterName=NanoJ Output #12\nObjectType=0x7\nDataType=0x0004\nAccessType=rwr\nDefaultValue=0x00000000\nPDOMapping=1\nObjFlags=1\n\n[2500subD]\nParameterName=NanoJ Output #13\nObjectType=0x7\nDataType=0x0004\nAccessType=rwr\nDefaultValue=0x00000000\nPDOMapping=1\nObjFlags=1\n\n[2500subE]\nParameterName=NanoJ Output #14\nObjectType=0x7\nDataType=0x0004\nAccessType=rwr\nDefaultValue=0x00000000\nPDOMapping=1\nObjFlags=1\n\n[2500subF]\nParameterName=NanoJ Output #15\nObjectType=0x7\nDataType=0x0004\nAccessType=rwr\nDefaultValue=0x00000000\nPDOMapping=1\nObjFlags=1\n\n[2500sub10]\nParameterName=NanoJ Output #16\nObjectType=0x7\nDataType=0x0004\nAccessType=rwr\nDefaultValue=0x00000000\nPDOMapping=1\nObjFlags=1\n\n[2500sub11]\nParameterName=NanoJ Output #17\nObjectType=0x7\nDataType=0x0004\nAccessType=rwr\nDefaultValue=0x00000000\nPDOMapping=1\nObjFlags=1\n\n[2500sub12]\nParameterName=NanoJ Output #18\nObjectType=0x7\nDataType=0x0004\nAccessType=rwr\nDefaultValue=0x00000000\nPDOMapping=1\nObjFlags=1\n\n[2500sub13]\nParameterName=NanoJ Output #19\nObjectType=0x7\nDataType=0x0004\nAccessType=rwr\nDefaultValue=0x00000000\nPDOMapping=1\nObjFlags=1\n\n[2500sub14]\nParameterName=NanoJ Output #20\nObjectType=0x7\nDataType=0x0004\nAccessType=rwr\nDefaultValue=0x00000000\nPDOMapping=1\nObjFlags=1\n\n[2500sub15]\nParameterName=NanoJ Output #21\nObjectType=0x7\nDataType=0x0004\nAccessType=rwr\nDefaultValue=0x00000000\nPDOMapping=1\nObjFlags=1\n\n[2500sub16]\nParameterName=NanoJ Output #22\nObjectType=0x7\nDataType=0x0004\nAccessType=rwr\nDefaultValue=0x00000000\nPDOMapping=1\nObjFlags=1\n\n[2500sub17]\nParameterName=NanoJ Output #23\nObjectType=0x7\nDataType=0x0004\nAccessType=rwr\nDefaultValue=0x00000000\nPDOMapping=1\nObjFlags=1\n\n[2500sub18]\nParameterName=NanoJ Output #24\nObjectType=0x7\nDataType=0x0004\nAccessType=rwr\nDefaultValue=0x00000000\nPDOMapping=1\nObjFlags=1\n\n[2500sub19]\nParameterName=NanoJ Output #25\nObjectType=0x7\nDataType=0x0004\nAccessType=rwr\nDefaultValue=0x00000000\nPDOMapping=1\nObjFlags=1\n\n[2500sub1A]\nParameterName=NanoJ Output #26\nObjectType=0x7\nDataType=0x0004\nAccessType=rwr\nDefaultValue=0x00000000\nPDOMapping=1\nObjFlags=1\n\n[2500sub1B]\nParameterName=NanoJ Output #27\nObjectType=0x7\nDataType=0x0004\nAccessType=rwr\nDefaultValue=0x00000000\nPDOMapping=1\nObjFlags=1\n\n[2500sub1C]\nParameterName=NanoJ Output #28\nObjectType=0x7\nDataType=0x0004\nAccessType=rwr\nDefaultValue=0x00000000\nPDOMapping=1\nObjFlags=1\n\n[2500sub1D]\nParameterName=NanoJ Output #29\nObjectType=0x7\nDataType=0x0004\nAccessType=rwr\nDefaultValue=0x00000000\nPDOMapping=1\nObjFlags=1\n\n[2500sub1E]\nParameterName=NanoJ Output #30\nObjectType=0x7\nDataType=0x0004\nAccessType=rwr\nDefaultValue=0x00000000\nPDOMapping=1\nObjFlags=1\n\n[2500sub1F]\nParameterName=NanoJ Output #31\nObjectType=0x7\nDataType=0x0004\nAccessType=rwr\nDefaultValue=0x00000000\nPDOMapping=1\nObjFlags=1\n\n[2500sub20]\nParameterName=NanoJ Output #32\nObjectType=0x7\nDataType=0x0004\nAccessType=rwr\nDefaultValue=0x00000000\nPDOMapping=1\nObjFlags=1\n\n[2600]\nParameterName=NanoJ Debug Output\nObjectType=0x8\nSubNumber=0x41\n\n[2600sub0]\nParameterName=Number of entries\nObjectType=0x7\nDataType=0x0005\nAccessType=rw\nDefaultValue=0x00\nPDOMapping=0\nObjFlags=1\n\n[2600sub1]\nParameterName=Value #1\nObjectType=0x7\nDataType=0x0005\nAccessType=ro\nDefaultValue=0x00\nPDOMapping=0\nObjFlags=1\n\n[2600sub2]\nParameterName=Value #2\nObjectType=0x7\nDataType=0x0005\nAccessType=ro\nDefaultValue=0x00\nPDOMapping=0\nObjFlags=1\n\n[2600sub3]\nParameterName=Value #3\nObjectType=0x7\nDataType=0x0005\nAccessType=ro\nDefaultValue=0x00\nPDOMapping=0\nObjFlags=1\n\n[2600sub4]\nParameterName=Value #4\nObjectType=0x7\nDataType=0x0005\nAccessType=ro\nDefaultValue=0x00\nPDOMapping=0\nObjFlags=1\n\n[2600sub5]\nParameterName=Value #5\nObjectType=0x7\nDataType=0x0005\nAccessType=ro\nDefaultValue=0x00\nPDOMapping=0\nObjFlags=1\n\n[2600sub6]\nParameterName=Value #6\nObjectType=0x7\nDataType=0x0005\nAccessType=ro\nDefaultValue=0x00\nPDOMapping=0\nObjFlags=1\n\n[2600sub7]\nParameterName=Value #7\nObjectType=0x7\nDataType=0x0005\nAccessType=ro\nDefaultValue=0x00\nPDOMapping=0\nObjFlags=1\n\n[2600sub8]\nParameterName=Value #8\nObjectType=0x7\nDataType=0x0005\nAccessType=ro\nDefaultValue=0x00\nPDOMapping=0\nObjFlags=1\n\n[2600sub9]\nParameterName=Value #9\nObjectType=0x7\nDataType=0x0005\nAccessType=ro\nDefaultValue=0x00\nPDOMapping=0\nObjFlags=1\n\n[2600subA]\nParameterName=Value #10\nObjectType=0x7\nDataType=0x0005\nAccessType=ro\nDefaultValue=0x00\nPDOMapping=0\nObjFlags=1\n\n[2600subB]\nParameterName=Value #11\nObjectType=0x7\nDataType=0x0005\nAccessType=ro\nDefaultValue=0x00\nPDOMapping=0\nObjFlags=1\n\n[2600subC]\nParameterName=Value #12\nObjectType=0x7\nDataType=0x0005\nAccessType=ro\nDefaultValue=0x00\nPDOMapping=0\nObjFlags=1\n\n[2600subD]\nParameterName=Value #13\nObjectType=0x7\nDataType=0x0005\nAccessType=ro\nDefaultValue=0x00\nPDOMapping=0\nObjFlags=1\n\n[2600subE]\nParameterName=Value #14\nObjectType=0x7\nDataType=0x0005\nAccessType=ro\nDefaultValue=0x00\nPDOMapping=0\nObjFlags=1\n\n[2600subF]\nParameterName=Value #15\nObjectType=0x7\nDataType=0x0005\nAccessType=ro\nDefaultValue=0x00\nPDOMapping=0\nObjFlags=1\n\n[2600sub10]\nParameterName=Value #16\nObjectType=0x7\nDataType=0x0005\nAccessType=ro\nDefaultValue=0x00\nPDOMapping=0\nObjFlags=1\n\n[2600sub11]\nParameterName=Value #17\nObjectType=0x7\nDataType=0x0005\nAccessType=ro\nDefaultValue=0x00\nPDOMapping=0\nObjFlags=1\n\n[2600sub12]\nParameterName=Value #18\nObjectType=0x7\nDataType=0x0005\nAccessType=ro\nDefaultValue=0x00\nPDOMapping=0\nObjFlags=1\n\n[2600sub13]\nParameterName=Value #19\nObjectType=0x7\nDataType=0x0005\nAccessType=ro\nDefaultValue=0x00\nPDOMapping=0\nObjFlags=1\n\n[2600sub14]\nParameterName=Value #20\nObjectType=0x7\nDataType=0x0005\nAccessType=ro\nDefaultValue=0x00\nPDOMapping=0\nObjFlags=1\n\n[2600sub15]\nParameterName=Value #21\nObjectType=0x7\nDataType=0x0005\nAccessType=ro\nDefaultValue=0x00\nPDOMapping=0\nObjFlags=1\n\n[2600sub16]\nParameterName=Value #22\nObjectType=0x7\nDataType=0x0005\nAccessType=ro\nDefaultValue=0x00\nPDOMapping=0\nObjFlags=1\n\n[2600sub17]\nParameterName=Value #23\nObjectType=0x7\nDataType=0x0005\nAccessType=ro\nDefaultValue=0x00\nPDOMapping=0\nObjFlags=1\n\n[2600sub18]\nParameterName=Value #24\nObjectType=0x7\nDataType=0x0005\nAccessType=ro\nDefaultValue=0x00\nPDOMapping=0\nObjFlags=1\n\n[2600sub19]\nParameterName=Value #25\nObjectType=0x7\nDataType=0x0005\nAccessType=ro\nDefaultValue=0x00\nPDOMapping=0\nObjFlags=1\n\n[2600sub1A]\nParameterName=Value #26\nObjectType=0x7\nDataType=0x0005\nAccessType=ro\nDefaultValue=0x00\nPDOMapping=0\nObjFlags=1\n\n[2600sub1B]\nParameterName=Value #27\nObjectType=0x7\nDataType=0x0005\nAccessType=ro\nDefaultValue=0x00\nPDOMapping=0\nObjFlags=1\n\n[2600sub1C]\nParameterName=Value #28\nObjectType=0x7\nDataType=0x0005\nAccessType=ro\nDefaultValue=0x00\nPDOMapping=0\nObjFlags=1\n\n[2600sub1D]\nParameterName=Value #29\nObjectType=0x7\nDataType=0x0005\nAccessType=ro\nDefaultValue=0x00\nPDOMapping=0\nObjFlags=1\n\n[2600sub1E]\nParameterName=Value #30\nObjectType=0x7\nDataType=0x0005\nAccessType=ro\nDefaultValue=0x00\nPDOMapping=0\nObjFlags=1\n\n[2600sub1F]\nParameterName=Value #31\nObjectType=0x7\nDataType=0x0005\nAccessType=ro\nDefaultValue=0x00\nPDOMapping=0\nObjFlags=1\n\n[2600sub20]\nParameterName=Value #32\nObjectType=0x7\nDataType=0x0005\nAccessType=ro\nDefaultValue=0x00\nPDOMapping=0\nObjFlags=1\n\n[2600sub21]\nParameterName=Value #33\nObjectType=0x7\nDataType=0x0005\nAccessType=ro\nDefaultValue=0x00\nPDOMapping=0\nObjFlags=1\n\n[2600sub22]\nParameterName=Value #34\nObjectType=0x7\nDataType=0x0005\nAccessType=ro\nDefaultValue=0x00\nPDOMapping=0\nObjFlags=1\n\n[2600sub23]\nParameterName=Value #35\nObjectType=0x7\nDataType=0x0005\nAccessType=ro\nDefaultValue=0x00\nPDOMapping=0\nObjFlags=1\n\n[2600sub24]\nParameterName=Value #36\nObjectType=0x7\nDataType=0x0005\nAccessType=ro\nDefaultValue=0x00\nPDOMapping=0\nObjFlags=1\n\n[2600sub25]\nParameterName=Value #37\nObjectType=0x7\nDataType=0x0005\nAccessType=ro\nDefaultValue=0x00\nPDOMapping=0\nObjFlags=1\n\n[2600sub26]\nParameterName=Value #38\nObjectType=0x7\nDataType=0x0005\nAccessType=ro\nDefaultValue=0x00\nPDOMapping=0\nObjFlags=1\n\n[2600sub27]\nParameterName=Value #39\nObjectType=0x7\nDataType=0x0005\nAccessType=ro\nDefaultValue=0x00\nPDOMapping=0\nObjFlags=1\n\n[2600sub28]\nParameterName=Value #40\nObjectType=0x7\nDataType=0x0005\nAccessType=ro\nDefaultValue=0x00\nPDOMapping=0\nObjFlags=1\n\n[2600sub29]\nParameterName=Value #41\nObjectType=0x7\nDataType=0x0005\nAccessType=ro\nDefaultValue=0x00\nPDOMapping=0\nObjFlags=1\n\n[2600sub2A]\nParameterName=Value #42\nObjectType=0x7\nDataType=0x0005\nAccessType=ro\nDefaultValue=0x00\nPDOMapping=0\nObjFlags=1\n\n[2600sub2B]\nParameterName=Value #43\nObjectType=0x7\nDataType=0x0005\nAccessType=ro\nDefaultValue=0x00\nPDOMapping=0\nObjFlags=1\n\n[2600sub2C]\nParameterName=Value #44\nObjectType=0x7\nDataType=0x0005\nAccessType=ro\nDefaultValue=0x00\nPDOMapping=0\nObjFlags=1\n\n[2600sub2D]\nParameterName=Value #45\nObjectType=0x7\nDataType=0x0005\nAccessType=ro\nDefaultValue=0x00\nPDOMapping=0\nObjFlags=1\n\n[2600sub2E]\nParameterName=Value #46\nObjectType=0x7\nDataType=0x0005\nAccessType=ro\nDefaultValue=0x00\nPDOMapping=0\nObjFlags=1\n\n[2600sub2F]\nParameterName=Value #47\nObjectType=0x7\nDataType=0x0005\nAccessType=ro\nDefaultValue=0x00\nPDOMapping=0\nObjFlags=1\n\n[2600sub30]\nParameterName=Value #48\nObjectType=0x7\nDataType=0x0005\nAccessType=ro\nDefaultValue=0x00\nPDOMapping=0\nObjFlags=1\n\n[2600sub31]\nParameterName=Value #49\nObjectType=0x7\nDataType=0x0005\nAccessType=ro\nDefaultValue=0x00\nPDOMapping=0\nObjFlags=1\n\n[2600sub32]\nParameterName=Value #50\nObjectType=0x7\nDataType=0x0005\nAccessType=ro\nDefaultValue=0x00\nPDOMapping=0\nObjFlags=1\n\n[2600sub33]\nParameterName=Value #51\nObjectType=0x7\nDataType=0x0005\nAccessType=ro\nDefaultValue=0x00\nPDOMapping=0\nObjFlags=1\n\n[2600sub34]\nParameterName=Value #52\nObjectType=0x7\nDataType=0x0005\nAccessType=ro\nDefaultValue=0x00\nPDOMapping=0\nObjFlags=1\n\n[2600sub35]\nParameterName=Value #53\nObjectType=0x7\nDataType=0x0005\nAccessType=ro\nDefaultValue=0x00\nPDOMapping=0\nObjFlags=1\n\n[2600sub36]\nParameterName=Value #54\nObjectType=0x7\nDataType=0x0005\nAccessType=ro\nDefaultValue=0x00\nPDOMapping=0\nObjFlags=1\n\n[2600sub37]\nParameterName=Value #55\nObjectType=0x7\nDataType=0x0005\nAccessType=ro\nDefaultValue=0x00\nPDOMapping=0\nObjFlags=1\n\n[2600sub38]\nParameterName=Value #56\nObjectType=0x7\nDataType=0x0005\nAccessType=ro\nDefaultValue=0x00\nPDOMapping=0\nObjFlags=1\n\n[2600sub39]\nParameterName=Value #57\nObjectType=0x7\nDataType=0x0005\nAccessType=ro\nDefaultValue=0x00\nPDOMapping=0\nObjFlags=1\n\n[2600sub3A]\nParameterName=Value #58\nObjectType=0x7\nDataType=0x0005\nAccessType=ro\nDefaultValue=0x00\nPDOMapping=0\nObjFlags=1\n\n[2600sub3B]\nParameterName=Value #59\nObjectType=0x7\nDataType=0x0005\nAccessType=ro\nDefaultValue=0x00\nPDOMapping=0\nObjFlags=1\n\n[2600sub3C]\nParameterName=Value #60\nObjectType=0x7\nDataType=0x0005\nAccessType=ro\nDefaultValue=0x00\nPDOMapping=0\nObjFlags=1\n\n[2600sub3D]\nParameterName=Value #61\nObjectType=0x7\nDataType=0x0005\nAccessType=ro\nDefaultValue=0x00\nPDOMapping=0\nObjFlags=1\n\n[2600sub3E]\nParameterName=Value #62\nObjectType=0x7\nDataType=0x0005\nAccessType=ro\nDefaultValue=0x00\nPDOMapping=0\nObjFlags=1\n\n[2600sub3F]\nParameterName=Value #63\nObjectType=0x7\nDataType=0x0005\nAccessType=ro\nDefaultValue=0x00\nPDOMapping=0\nObjFlags=1\n\n[2600sub40]\nParameterName=Value #64\nObjectType=0x7\nDataType=0x0005\nAccessType=ro\nDefaultValue=0x00\nPDOMapping=0\nObjFlags=1\n\n[2701]\nParameterName=Customer storage area\nObjectType=0x8\nSubNumber=0xFF\n\n[2701sub0]\nParameterName=Number of entries\nObjectType=0x7\nDataType=0x0005\nAccessType=ro\nDefaultValue=0xFE\nPDOMapping=0\n\n[2701sub1]\nParameterName=Storage #1\nObjectType=0x7\nDataType=0x0007\nAccessType=rw\nDefaultValue=0x00000000\nPDOMapping=0\n\n[2701sub2]\nParameterName=Storage #2\nObjectType=0x7\nDataType=0x0007\nAccessType=rw\nDefaultValue=0x00000000\nPDOMapping=0\n\n[2701sub3]\nParameterName=Storage #3\nObjectType=0x7\nDataType=0x0007\nAccessType=rw\nDefaultValue=0x00000000\nPDOMapping=0\n\n[2701sub4]\nParameterName=Storage #4\nObjectType=0x7\nDataType=0x0007\nAccessType=rw\nDefaultValue=0x00000000\nPDOMapping=0\n\n[2701sub5]\nParameterName=Storage #5\nObjectType=0x7\nDataType=0x0007\nAccessType=rw\nDefaultValue=0x00000000\nPDOMapping=0\n\n[2701sub6]\nParameterName=Storage #6\nObjectType=0x7\nDataType=0x0007\nAccessType=rw\nDefaultValue=0x00000000\nPDOMapping=0\n\n[2701sub7]\nParameterName=Storage #7\nObjectType=0x7\nDataType=0x0007\nAccessType=rw\nDefaultValue=0x00000000\nPDOMapping=0\n\n[2701sub8]\nParameterName=Storage #8\nObjectType=0x7\nDataType=0x0007\nAccessType=rw\nDefaultValue=0x00000000\nPDOMapping=0\n\n[2701sub9]\nParameterName=Storage #9\nObjectType=0x7\nDataType=0x0007\nAccessType=rw\nDefaultValue=0x00000000\nPDOMapping=0\n\n[2701subA]\nParameterName=Storage #10\nObjectType=0x7\nDataType=0x0007\nAccessType=rw\nDefaultValue=0x00000000\nPDOMapping=0\n\n[2701subB]\nParameterName=Storage #11\nObjectType=0x7\nDataType=0x0007\nAccessType=rw\nDefaultValue=0x00000000\nPDOMapping=0\n\n[2701subC]\nParameterName=Storage #12\nObjectType=0x7\nDataType=0x0007\nAccessType=rw\nDefaultValue=0x00000000\nPDOMapping=0\n\n[2701subD]\nParameterName=Storage #13\nObjectType=0x7\nDataType=0x0007\nAccessType=rw\nDefaultValue=0x00000000\nPDOMapping=0\n\n[2701subE]\nParameterName=Storage #14\nObjectType=0x7\nDataType=0x0007\nAccessType=rw\nDefaultValue=0x00000000\nPDOMapping=0\n\n[2701subF]\nParameterName=Storage #15\nObjectType=0x7\nDataType=0x0007\nAccessType=rw\nDefaultValue=0x00000000\nPDOMapping=0\n\n[2701sub10]\nParameterName=Storage #16\nObjectType=0x7\nDataType=0x0007\nAccessType=rw\nDefaultValue=0x00000000\nPDOMapping=0\n\n[2701sub11]\nParameterName=Storage #17\nObjectType=0x7\nDataType=0x0007\nAccessType=rw\nDefaultValue=0x00000000\nPDOMapping=0\n\n[2701sub12]\nParameterName=Storage #18\nObjectType=0x7\nDataType=0x0007\nAccessType=rw\nDefaultValue=0x00000000\nPDOMapping=0\n\n[2701sub13]\nParameterName=Storage #19\nObjectType=0x7\nDataType=0x0007\nAccessType=rw\nDefaultValue=0x00000000\nPDOMapping=0\n\n[2701sub14]\nParameterName=Storage #20\nObjectType=0x7\nDataType=0x0007\nAccessType=rw\nDefaultValue=0x00000000\nPDOMapping=0\n\n[2701sub15]\nParameterName=Storage #21\nObjectType=0x7\nDataType=0x0007\nAccessType=rw\nDefaultValue=0x00000000\nPDOMapping=0\n\n[2701sub16]\nParameterName=Storage #22\nObjectType=0x7\nDataType=0x0007\nAccessType=rw\nDefaultValue=0x00000000\nPDOMapping=0\n\n[2701sub17]\nParameterName=Storage #23\nObjectType=0x7\nDataType=0x0007\nAccessType=rw\nDefaultValue=0x00000000\nPDOMapping=0\n\n[2701sub18]\nParameterName=Storage #24\nObjectType=0x7\nDataType=0x0007\nAccessType=rw\nDefaultValue=0x00000000\nPDOMapping=0\n\n[2701sub19]\nParameterName=Storage #25\nObjectType=0x7\nDataType=0x0007\nAccessType=rw\nDefaultValue=0x00000000\nPDOMapping=0\n\n[2701sub1A]\nParameterName=Storage #26\nObjectType=0x7\nDataType=0x0007\nAccessType=rw\nDefaultValue=0x00000000\nPDOMapping=0\n\n[2701sub1B]\nParameterName=Storage #27\nObjectType=0x7\nDataType=0x0007\nAccessType=rw\nDefaultValue=0x00000000\nPDOMapping=0\n\n[2701sub1C]\nParameterName=Storage #28\nObjectType=0x7\nDataType=0x0007\nAccessType=rw\nDefaultValue=0x00000000\nPDOMapping=0\n\n[2701sub1D]\nParameterName=Storage #29\nObjectType=0x7\nDataType=0x0007\nAccessType=rw\nDefaultValue=0x00000000\nPDOMapping=0\n\n[2701sub1E]\nParameterName=Storage #30\nObjectType=0x7\nDataType=0x0007\nAccessType=rw\nDefaultValue=0x00000000\nPDOMapping=0\n\n[2701sub1F]\nParameterName=Storage #31\nObjectType=0x7\nDataType=0x0007\nAccessType=rw\nDefaultValue=0x00000000\nPDOMapping=0\n\n[2701sub20]\nParameterName=Storage #32\nObjectType=0x7\nDataType=0x0007\nAccessType=rw\nDefaultValue=0x00000000\nPDOMapping=0\n\n[2701sub21]\nParameterName=Storage #33\nObjectType=0x7\nDataType=0x0007\nAccessType=rw\nDefaultValue=0x00000000\nPDOMapping=0\n\n[2701sub22]\nParameterName=Storage #34\nObjectType=0x7\nDataType=0x0007\nAccessType=rw\nDefaultValue=0x00000000\nPDOMapping=0\n\n[2701sub23]\nParameterName=Storage #35\nObjectType=0x7\nDataType=0x0007\nAccessType=rw\nDefaultValue=0x00000000\nPDOMapping=0\n\n[2701sub24]\nParameterName=Storage #36\nObjectType=0x7\nDataType=0x0007\nAccessType=rw\nDefaultValue=0x00000000\nPDOMapping=0\n\n[2701sub25]\nParameterName=Storage #37\nObjectType=0x7\nDataType=0x0007\nAccessType=rw\nDefaultValue=0x00000000\nPDOMapping=0\n\n[2701sub26]\nParameterName=Storage #38\nObjectType=0x7\nDataType=0x0007\nAccessType=rw\nDefaultValue=0x00000000\nPDOMapping=0\n\n[2701sub27]\nParameterName=Storage #39\nObjectType=0x7\nDataType=0x0007\nAccessType=rw\nDefaultValue=0x00000000\nPDOMapping=0\n\n[2701sub28]\nParameterName=Storage #40\nObjectType=0x7\nDataType=0x0007\nAccessType=rw\nDefaultValue=0x00000000\nPDOMapping=0\n\n[2701sub29]\nParameterName=Storage #41\nObjectType=0x7\nDataType=0x0007\nAccessType=rw\nDefaultValue=0x00000000\nPDOMapping=0\n\n[2701sub2A]\nParameterName=Storage #42\nObjectType=0x7\nDataType=0x0007\nAccessType=rw\nDefaultValue=0x00000000\nPDOMapping=0\n\n[2701sub2B]\nParameterName=Storage #43\nObjectType=0x7\nDataType=0x0007\nAccessType=rw\nDefaultValue=0x00000000\nPDOMapping=0\n\n[2701sub2C]\nParameterName=Storage #44\nObjectType=0x7\nDataType=0x0007\nAccessType=rw\nDefaultValue=0x00000000\nPDOMapping=0\n\n[2701sub2D]\nParameterName=Storage #45\nObjectType=0x7\nDataType=0x0007\nAccessType=rw\nDefaultValue=0x00000000\nPDOMapping=0\n\n[2701sub2E]\nParameterName=Storage #46\nObjectType=0x7\nDataType=0x0007\nAccessType=rw\nDefaultValue=0x00000000\nPDOMapping=0\n\n[2701sub2F]\nParameterName=Storage #47\nObjectType=0x7\nDataType=0x0007\nAccessType=rw\nDefaultValue=0x00000000\nPDOMapping=0\n\n[2701sub30]\nParameterName=Storage #48\nObjectType=0x7\nDataType=0x0007\nAccessType=rw\nDefaultValue=0x00000000\nPDOMapping=0\n\n[2701sub31]\nParameterName=Storage #49\nObjectType=0x7\nDataType=0x0007\nAccessType=rw\nDefaultValue=0x00000000\nPDOMapping=0\n\n[2701sub32]\nParameterName=Storage #50\nObjectType=0x7\nDataType=0x0007\nAccessType=rw\nDefaultValue=0x00000000\nPDOMapping=0\n\n[2701sub33]\nParameterName=Storage #51\nObjectType=0x7\nDataType=0x0007\nAccessType=rw\nDefaultValue=0x00000000\nPDOMapping=0\n\n[2701sub34]\nParameterName=Storage #52\nObjectType=0x7\nDataType=0x0007\nAccessType=rw\nDefaultValue=0x00000000\nPDOMapping=0\n\n[2701sub35]\nParameterName=Storage #53\nObjectType=0x7\nDataType=0x0007\nAccessType=rw\nDefaultValue=0x00000000\nPDOMapping=0\n\n[2701sub36]\nParameterName=Storage #54\nObjectType=0x7\nDataType=0x0007\nAccessType=rw\nDefaultValue=0x00000000\nPDOMapping=0\n\n[2701sub37]\nParameterName=Storage #55\nObjectType=0x7\nDataType=0x0007\nAccessType=rw\nDefaultValue=0x00000000\nPDOMapping=0\n\n[2701sub38]\nParameterName=Storage #56\nObjectType=0x7\nDataType=0x0007\nAccessType=rw\nDefaultValue=0x00000000\nPDOMapping=0\n\n[2701sub39]\nParameterName=Storage #57\nObjectType=0x7\nDataType=0x0007\nAccessType=rw\nDefaultValue=0x00000000\nPDOMapping=0\n\n[2701sub3A]\nParameterName=Storage #58\nObjectType=0x7\nDataType=0x0007\nAccessType=rw\nDefaultValue=0x00000000\nPDOMapping=0\n\n[2701sub3B]\nParameterName=Storage #59\nObjectType=0x7\nDataType=0x0007\nAccessType=rw\nDefaultValue=0x00000000\nPDOMapping=0\n\n[2701sub3C]\nParameterName=Storage #60\nObjectType=0x7\nDataType=0x0007\nAccessType=rw\nDefaultValue=0x00000000\nPDOMapping=0\n\n[2701sub3D]\nParameterName=Storage #61\nObjectType=0x7\nDataType=0x0007\nAccessType=rw\nDefaultValue=0x00000000\nPDOMapping=0\n\n[2701sub3E]\nParameterName=Storage #62\nObjectType=0x7\nDataType=0x0007\nAccessType=rw\nDefaultValue=0x00000000\nPDOMapping=0\n\n[2701sub3F]\nParameterName=Storage #63\nObjectType=0x7\nDataType=0x0007\nAccessType=rw\nDefaultValue=0x00000000\nPDOMapping=0\n\n[2701sub40]\nParameterName=Storage #64\nObjectType=0x7\nDataType=0x0007\nAccessType=rw\nDefaultValue=0x00000000\nPDOMapping=0\n\n[2701sub41]\nParameterName=Storage #65\nObjectType=0x7\nDataType=0x0007\nAccessType=rw\nDefaultValue=0x00000000\nPDOMapping=0\n\n[2701sub42]\nParameterName=Storage #66\nObjectType=0x7\nDataType=0x0007\nAccessType=rw\nDefaultValue=0x00000000\nPDOMapping=0\n\n[2701sub43]\nParameterName=Storage #67\nObjectType=0x7\nDataType=0x0007\nAccessType=rw\nDefaultValue=0x00000000\nPDOMapping=0\n\n[2701sub44]\nParameterName=Storage #68\nObjectType=0x7\nDataType=0x0007\nAccessType=rw\nDefaultValue=0x00000000\nPDOMapping=0\n\n[2701sub45]\nParameterName=Storage #69\nObjectType=0x7\nDataType=0x0007\nAccessType=rw\nDefaultValue=0x00000000\nPDOMapping=0\n\n[2701sub46]\nParameterName=Storage #70\nObjectType=0x7\nDataType=0x0007\nAccessType=rw\nDefaultValue=0x00000000\nPDOMapping=0\n\n[2701sub47]\nParameterName=Storage #71\nObjectType=0x7\nDataType=0x0007\nAccessType=rw\nDefaultValue=0x00000000\nPDOMapping=0\n\n[2701sub48]\nParameterName=Storage #72\nObjectType=0x7\nDataType=0x0007\nAccessType=rw\nDefaultValue=0x00000000\nPDOMapping=0\n\n[2701sub49]\nParameterName=Storage #73\nObjectType=0x7\nDataType=0x0007\nAccessType=rw\nDefaultValue=0x00000000\nPDOMapping=0\n\n[2701sub4A]\nParameterName=Storage #74\nObjectType=0x7\nDataType=0x0007\nAccessType=rw\nDefaultValue=0x00000000\nPDOMapping=0\n\n[2701sub4B]\nParameterName=Storage #75\nObjectType=0x7\nDataType=0x0007\nAccessType=rw\nDefaultValue=0x00000000\nPDOMapping=0\n\n[2701sub4C]\nParameterName=Storage #76\nObjectType=0x7\nDataType=0x0007\nAccessType=rw\nDefaultValue=0x00000000\nPDOMapping=0\n\n[2701sub4D]\nParameterName=Storage #77\nObjectType=0x7\nDataType=0x0007\nAccessType=rw\nDefaultValue=0x00000000\nPDOMapping=0\n\n[2701sub4E]\nParameterName=Storage #78\nObjectType=0x7\nDataType=0x0007\nAccessType=rw\nDefaultValue=0x00000000\nPDOMapping=0\n\n[2701sub4F]\nParameterName=Storage #79\nObjectType=0x7\nDataType=0x0007\nAccessType=rw\nDefaultValue=0x00000000\nPDOMapping=0\n\n[2701sub50]\nParameterName=Storage #80\nObjectType=0x7\nDataType=0x0007\nAccessType=rw\nDefaultValue=0x00000000\nPDOMapping=0\n\n[2701sub51]\nParameterName=Storage #81\nObjectType=0x7\nDataType=0x0007\nAccessType=rw\nDefaultValue=0x00000000\nPDOMapping=0\n\n[2701sub52]\nParameterName=Storage #82\nObjectType=0x7\nDataType=0x0007\nAccessType=rw\nDefaultValue=0x00000000\nPDOMapping=0\n\n[2701sub53]\nParameterName=Storage #83\nObjectType=0x7\nDataType=0x0007\nAccessType=rw\nDefaultValue=0x00000000\nPDOMapping=0\n\n[2701sub54]\nParameterName=Storage #84\nObjectType=0x7\nDataType=0x0007\nAccessType=rw\nDefaultValue=0x00000000\nPDOMapping=0\n\n[2701sub55]\nParameterName=Storage #85\nObjectType=0x7\nDataType=0x0007\nAccessType=rw\nDefaultValue=0x00000000\nPDOMapping=0\n\n[2701sub56]\nParameterName=Storage #86\nObjectType=0x7\nDataType=0x0007\nAccessType=rw\nDefaultValue=0x00000000\nPDOMapping=0\n\n[2701sub57]\nParameterName=Storage #87\nObjectType=0x7\nDataType=0x0007\nAccessType=rw\nDefaultValue=0x00000000\nPDOMapping=0\n\n[2701sub58]\nParameterName=Storage #88\nObjectType=0x7\nDataType=0x0007\nAccessType=rw\nDefaultValue=0x00000000\nPDOMapping=0\n\n[2701sub59]\nParameterName=Storage #89\nObjectType=0x7\nDataType=0x0007\nAccessType=rw\nDefaultValue=0x00000000\nPDOMapping=0\n\n[2701sub5A]\nParameterName=Storage #90\nObjectType=0x7\nDataType=0x0007\nAccessType=rw\nDefaultValue=0x00000000\nPDOMapping=0\n\n[2701sub5B]\nParameterName=Storage #91\nObjectType=0x7\nDataType=0x0007\nAccessType=rw\nDefaultValue=0x00000000\nPDOMapping=0\n\n[2701sub5C]\nParameterName=Storage #92\nObjectType=0x7\nDataType=0x0007\nAccessType=rw\nDefaultValue=0x00000000\nPDOMapping=0\n\n[2701sub5D]\nParameterName=Storage #93\nObjectType=0x7\nDataType=0x0007\nAccessType=rw\nDefaultValue=0x00000000\nPDOMapping=0\n\n[2701sub5E]\nParameterName=Storage #94\nObjectType=0x7\nDataType=0x0007\nAccessType=rw\nDefaultValue=0x00000000\nPDOMapping=0\n\n[2701sub5F]\nParameterName=Storage #95\nObjectType=0x7\nDataType=0x0007\nAccessType=rw\nDefaultValue=0x00000000\nPDOMapping=0\n\n[2701sub60]\nParameterName=Storage #96\nObjectType=0x7\nDataType=0x0007\nAccessType=rw\nDefaultValue=0x00000000\nPDOMapping=0\n\n[2701sub61]\nParameterName=Storage #97\nObjectType=0x7\nDataType=0x0007\nAccessType=rw\nDefaultValue=0x00000000\nPDOMapping=0\n\n[2701sub62]\nParameterName=Storage #98\nObjectType=0x7\nDataType=0x0007\nAccessType=rw\nDefaultValue=0x00000000\nPDOMapping=0\n\n[2701sub63]\nParameterName=Storage #99\nObjectType=0x7\nDataType=0x0007\nAccessType=rw\nDefaultValue=0x00000000\nPDOMapping=0\n\n[2701sub64]\nParameterName=Storage #100\nObjectType=0x7\nDataType=0x0007\nAccessType=rw\nDefaultValue=0x00000000\nPDOMapping=0\n\n[2701sub65]\nParameterName=Storage #101\nObjectType=0x7\nDataType=0x0007\nAccessType=rw\nDefaultValue=0x00000000\nPDOMapping=0\n\n[2701sub66]\nParameterName=Storage #102\nObjectType=0x7\nDataType=0x0007\nAccessType=rw\nDefaultValue=0x00000000\nPDOMapping=0\n\n[2701sub67]\nParameterName=Storage #103\nObjectType=0x7\nDataType=0x0007\nAccessType=rw\nDefaultValue=0x00000000\nPDOMapping=0\n\n[2701sub68]\nParameterName=Storage #104\nObjectType=0x7\nDataType=0x0007\nAccessType=rw\nDefaultValue=0x00000000\nPDOMapping=0\n\n[2701sub69]\nParameterName=Storage #105\nObjectType=0x7\nDataType=0x0007\nAccessType=rw\nDefaultValue=0x00000000\nPDOMapping=0\n\n[2701sub6A]\nParameterName=Storage #106\nObjectType=0x7\nDataType=0x0007\nAccessType=rw\nDefaultValue=0x00000000\nPDOMapping=0\n\n[2701sub6B]\nParameterName=Storage #107\nObjectType=0x7\nDataType=0x0007\nAccessType=rw\nDefaultValue=0x00000000\nPDOMapping=0\n\n[2701sub6C]\nParameterName=Storage #108\nObjectType=0x7\nDataType=0x0007\nAccessType=rw\nDefaultValue=0x00000000\nPDOMapping=0\n\n[2701sub6D]\nParameterName=Storage #109\nObjectType=0x7\nDataType=0x0007\nAccessType=rw\nDefaultValue=0x00000000\nPDOMapping=0\n\n[2701sub6E]\nParameterName=Storage #110\nObjectType=0x7\nDataType=0x0007\nAccessType=rw\nDefaultValue=0x00000000\nPDOMapping=0\n\n[2701sub6F]\nParameterName=Storage #111\nObjectType=0x7\nDataType=0x0007\nAccessType=rw\nDefaultValue=0x00000000\nPDOMapping=0\n\n[2701sub70]\nParameterName=Storage #112\nObjectType=0x7\nDataType=0x0007\nAccessType=rw\nDefaultValue=0x00000000\nPDOMapping=0\n\n[2701sub71]\nParameterName=Storage #113\nObjectType=0x7\nDataType=0x0007\nAccessType=rw\nDefaultValue=0x00000000\nPDOMapping=0\n\n[2701sub72]\nParameterName=Storage #114\nObjectType=0x7\nDataType=0x0007\nAccessType=rw\nDefaultValue=0x00000000\nPDOMapping=0\n\n[2701sub73]\nParameterName=Storage #115\nObjectType=0x7\nDataType=0x0007\nAccessType=rw\nDefaultValue=0x00000000\nPDOMapping=0\n\n[2701sub74]\nParameterName=Storage #116\nObjectType=0x7\nDataType=0x0007\nAccessType=rw\nDefaultValue=0x00000000\nPDOMapping=0\n\n[2701sub75]\nParameterName=Storage #117\nObjectType=0x7\nDataType=0x0007\nAccessType=rw\nDefaultValue=0x00000000\nPDOMapping=0\n\n[2701sub76]\nParameterName=Storage #118\nObjectType=0x7\nDataType=0x0007\nAccessType=rw\nDefaultValue=0x00000000\nPDOMapping=0\n\n[2701sub77]\nParameterName=Storage #119\nObjectType=0x7\nDataType=0x0007\nAccessType=rw\nDefaultValue=0x00000000\nPDOMapping=0\n\n[2701sub78]\nParameterName=Storage #120\nObjectType=0x7\nDataType=0x0007\nAccessType=rw\nDefaultValue=0x00000000\nPDOMapping=0\n\n[2701sub79]\nParameterName=Storage #121\nObjectType=0x7\nDataType=0x0007\nAccessType=rw\nDefaultValue=0x00000000\nPDOMapping=0\n\n[2701sub7A]\nParameterName=Storage #122\nObjectType=0x7\nDataType=0x0007\nAccessType=rw\nDefaultValue=0x00000000\nPDOMapping=0\n\n[2701sub7B]\nParameterName=Storage #123\nObjectType=0x7\nDataType=0x0007\nAccessType=rw\nDefaultValue=0x00000000\nPDOMapping=0\n\n[2701sub7C]\nParameterName=Storage #124\nObjectType=0x7\nDataType=0x0007\nAccessType=rw\nDefaultValue=0x00000000\nPDOMapping=0\n\n[2701sub7D]\nParameterName=Storage #125\nObjectType=0x7\nDataType=0x0007\nAccessType=rw\nDefaultValue=0x00000000\nPDOMapping=0\n\n[2701sub7E]\nParameterName=Storage #126\nObjectType=0x7\nDataType=0x0007\nAccessType=rw\nDefaultValue=0x00000000\nPDOMapping=0\n\n[2701sub7F]\nParameterName=Storage #127\nObjectType=0x7\nDataType=0x0007\nAccessType=rw\nDefaultValue=0x00000000\nPDOMapping=0\n\n[2701sub80]\nParameterName=Storage #128\nObjectType=0x7\nDataType=0x0007\nAccessType=rw\nDefaultValue=0x00000000\nPDOMapping=0\n\n[2701sub81]\nParameterName=Storage #129\nObjectType=0x7\nDataType=0x0007\nAccessType=rw\nDefaultValue=0x00000000\nPDOMapping=0\n\n[2701sub82]\nParameterName=Storage #130\nObjectType=0x7\nDataType=0x0007\nAccessType=rw\nDefaultValue=0x00000000\nPDOMapping=0\n\n[2701sub83]\nParameterName=Storage #131\nObjectType=0x7\nDataType=0x0007\nAccessType=rw\nDefaultValue=0x00000000\nPDOMapping=0\n\n[2701sub84]\nParameterName=Storage #132\nObjectType=0x7\nDataType=0x0007\nAccessType=rw\nDefaultValue=0x00000000\nPDOMapping=0\n\n[2701sub85]\nParameterName=Storage #133\nObjectType=0x7\nDataType=0x0007\nAccessType=rw\nDefaultValue=0x00000000\nPDOMapping=0\n\n[2701sub86]\nParameterName=Storage #134\nObjectType=0x7\nDataType=0x0007\nAccessType=rw\nDefaultValue=0x00000000\nPDOMapping=0\n\n[2701sub87]\nParameterName=Storage #135\nObjectType=0x7\nDataType=0x0007\nAccessType=rw\nDefaultValue=0x00000000\nPDOMapping=0\n\n[2701sub88]\nParameterName=Storage #136\nObjectType=0x7\nDataType=0x0007\nAccessType=rw\nDefaultValue=0x00000000\nPDOMapping=0\n\n[2701sub89]\nParameterName=Storage #137\nObjectType=0x7\nDataType=0x0007\nAccessType=rw\nDefaultValue=0x00000000\nPDOMapping=0\n\n[2701sub8A]\nParameterName=Storage #138\nObjectType=0x7\nDataType=0x0007\nAccessType=rw\nDefaultValue=0x00000000\nPDOMapping=0\n\n[2701sub8B]\nParameterName=Storage #139\nObjectType=0x7\nDataType=0x0007\nAccessType=rw\nDefaultValue=0x00000000\nPDOMapping=0\n\n[2701sub8C]\nParameterName=Storage #140\nObjectType=0x7\nDataType=0x0007\nAccessType=rw\nDefaultValue=0x00000000\nPDOMapping=0\n\n[2701sub8D]\nParameterName=Storage #141\nObjectType=0x7\nDataType=0x0007\nAccessType=rw\nDefaultValue=0x00000000\nPDOMapping=0\n\n[2701sub8E]\nParameterName=Storage #142\nObjectType=0x7\nDataType=0x0007\nAccessType=rw\nDefaultValue=0x00000000\nPDOMapping=0\n\n[2701sub8F]\nParameterName=Storage #143\nObjectType=0x7\nDataType=0x0007\nAccessType=rw\nDefaultValue=0x00000000\nPDOMapping=0\n\n[2701sub90]\nParameterName=Storage #144\nObjectType=0x7\nDataType=0x0007\nAccessType=rw\nDefaultValue=0x00000000\nPDOMapping=0\n\n[2701sub91]\nParameterName=Storage #145\nObjectType=0x7\nDataType=0x0007\nAccessType=rw\nDefaultValue=0x00000000\nPDOMapping=0\n\n[2701sub92]\nParameterName=Storage #146\nObjectType=0x7\nDataType=0x0007\nAccessType=rw\nDefaultValue=0x00000000\nPDOMapping=0\n\n[2701sub93]\nParameterName=Storage #147\nObjectType=0x7\nDataType=0x0007\nAccessType=rw\nDefaultValue=0x00000000\nPDOMapping=0\n\n[2701sub94]\nParameterName=Storage #148\nObjectType=0x7\nDataType=0x0007\nAccessType=rw\nDefaultValue=0x00000000\nPDOMapping=0\n\n[2701sub95]\nParameterName=Storage #149\nObjectType=0x7\nDataType=0x0007\nAccessType=rw\nDefaultValue=0x00000000\nPDOMapping=0\n\n[2701sub96]\nParameterName=Storage #150\nObjectType=0x7\nDataType=0x0007\nAccessType=rw\nDefaultValue=0x00000000\nPDOMapping=0\n\n[2701sub97]\nParameterName=Storage #151\nObjectType=0x7\nDataType=0x0007\nAccessType=rw\nDefaultValue=0x00000000\nPDOMapping=0\n\n[2701sub98]\nParameterName=Storage #152\nObjectType=0x7\nDataType=0x0007\nAccessType=rw\nDefaultValue=0x00000000\nPDOMapping=0\n\n[2701sub99]\nParameterName=Storage #153\nObjectType=0x7\nDataType=0x0007\nAccessType=rw\nDefaultValue=0x00000000\nPDOMapping=0\n\n[2701sub9A]\nParameterName=Storage #154\nObjectType=0x7\nDataType=0x0007\nAccessType=rw\nDefaultValue=0x00000000\nPDOMapping=0\n\n[2701sub9B]\nParameterName=Storage #155\nObjectType=0x7\nDataType=0x0007\nAccessType=rw\nDefaultValue=0x00000000\nPDOMapping=0\n\n[2701sub9C]\nParameterName=Storage #156\nObjectType=0x7\nDataType=0x0007\nAccessType=rw\nDefaultValue=0x00000000\nPDOMapping=0\n\n[2701sub9D]\nParameterName=Storage #157\nObjectType=0x7\nDataType=0x0007\nAccessType=rw\nDefaultValue=0x00000000\nPDOMapping=0\n\n[2701sub9E]\nParameterName=Storage #158\nObjectType=0x7\nDataType=0x0007\nAccessType=rw\nDefaultValue=0x00000000\nPDOMapping=0\n\n[2701sub9F]\nParameterName=Storage #159\nObjectType=0x7\nDataType=0x0007\nAccessType=rw\nDefaultValue=0x00000000\nPDOMapping=0\n\n[2701subA0]\nParameterName=Storage #160\nObjectType=0x7\nDataType=0x0007\nAccessType=rw\nDefaultValue=0x00000000\nPDOMapping=0\n\n[2701subA1]\nParameterName=Storage #161\nObjectType=0x7\nDataType=0x0007\nAccessType=rw\nDefaultValue=0x00000000\nPDOMapping=0\n\n[2701subA2]\nParameterName=Storage #162\nObjectType=0x7\nDataType=0x0007\nAccessType=rw\nDefaultValue=0x00000000\nPDOMapping=0\n\n[2701subA3]\nParameterName=Storage #163\nObjectType=0x7\nDataType=0x0007\nAccessType=rw\nDefaultValue=0x00000000\nPDOMapping=0\n\n[2701subA4]\nParameterName=Storage #164\nObjectType=0x7\nDataType=0x0007\nAccessType=rw\nDefaultValue=0x00000000\nPDOMapping=0\n\n[2701subA5]\nParameterName=Storage #165\nObjectType=0x7\nDataType=0x0007\nAccessType=rw\nDefaultValue=0x00000000\nPDOMapping=0\n\n[2701subA6]\nParameterName=Storage #166\nObjectType=0x7\nDataType=0x0007\nAccessType=rw\nDefaultValue=0x00000000\nPDOMapping=0\n\n[2701subA7]\nParameterName=Storage #167\nObjectType=0x7\nDataType=0x0007\nAccessType=rw\nDefaultValue=0x00000000\nPDOMapping=0\n\n[2701subA8]\nParameterName=Storage #168\nObjectType=0x7\nDataType=0x0007\nAccessType=rw\nDefaultValue=0x00000000\nPDOMapping=0\n\n[2701subA9]\nParameterName=Storage #169\nObjectType=0x7\nDataType=0x0007\nAccessType=rw\nDefaultValue=0x00000000\nPDOMapping=0\n\n[2701subAA]\nParameterName=Storage #170\nObjectType=0x7\nDataType=0x0007\nAccessType=rw\nDefaultValue=0x00000000\nPDOMapping=0\n\n[2701subAB]\nParameterName=Storage #171\nObjectType=0x7\nDataType=0x0007\nAccessType=rw\nDefaultValue=0x00000000\nPDOMapping=0\n\n[2701subAC]\nParameterName=Storage #172\nObjectType=0x7\nDataType=0x0007\nAccessType=rw\nDefaultValue=0x00000000\nPDOMapping=0\n\n[2701subAD]\nParameterName=Storage #173\nObjectType=0x7\nDataType=0x0007\nAccessType=rw\nDefaultValue=0x00000000\nPDOMapping=0\n\n[2701subAE]\nParameterName=Storage #174\nObjectType=0x7\nDataType=0x0007\nAccessType=rw\nDefaultValue=0x00000000\nPDOMapping=0\n\n[2701subAF]\nParameterName=Storage #175\nObjectType=0x7\nDataType=0x0007\nAccessType=rw\nDefaultValue=0x00000000\nPDOMapping=0\n\n[2701subB0]\nParameterName=Storage #176\nObjectType=0x7\nDataType=0x0007\nAccessType=rw\nDefaultValue=0x00000000\nPDOMapping=0\n\n[2701subB1]\nParameterName=Storage #177\nObjectType=0x7\nDataType=0x0007\nAccessType=rw\nDefaultValue=0x00000000\nPDOMapping=0\n\n[2701subB2]\nParameterName=Storage #178\nObjectType=0x7\nDataType=0x0007\nAccessType=rw\nDefaultValue=0x00000000\nPDOMapping=0\n\n[2701subB3]\nParameterName=Storage #179\nObjectType=0x7\nDataType=0x0007\nAccessType=rw\nDefaultValue=0x00000000\nPDOMapping=0\n\n[2701subB4]\nParameterName=Storage #180\nObjectType=0x7\nDataType=0x0007\nAccessType=rw\nDefaultValue=0x00000000\nPDOMapping=0\n\n[2701subB5]\nParameterName=Storage #181\nObjectType=0x7\nDataType=0x0007\nAccessType=rw\nDefaultValue=0x00000000\nPDOMapping=0\n\n[2701subB6]\nParameterName=Storage #182\nObjectType=0x7\nDataType=0x0007\nAccessType=rw\nDefaultValue=0x00000000\nPDOMapping=0\n\n[2701subB7]\nParameterName=Storage #183\nObjectType=0x7\nDataType=0x0007\nAccessType=rw\nDefaultValue=0x00000000\nPDOMapping=0\n\n[2701subB8]\nParameterName=Storage #184\nObjectType=0x7\nDataType=0x0007\nAccessType=rw\nDefaultValue=0x00000000\nPDOMapping=0\n\n[2701subB9]\nParameterName=Storage #185\nObjectType=0x7\nDataType=0x0007\nAccessType=rw\nDefaultValue=0x00000000\nPDOMapping=0\n\n[2701subBA]\nParameterName=Storage #186\nObjectType=0x7\nDataType=0x0007\nAccessType=rw\nDefaultValue=0x00000000\nPDOMapping=0\n\n[2701subBB]\nParameterName=Storage #187\nObjectType=0x7\nDataType=0x0007\nAccessType=rw\nDefaultValue=0x00000000\nPDOMapping=0\n\n[2701subBC]\nParameterName=Storage #188\nObjectType=0x7\nDataType=0x0007\nAccessType=rw\nDefaultValue=0x00000000\nPDOMapping=0\n\n[2701subBD]\nParameterName=Storage #189\nObjectType=0x7\nDataType=0x0007\nAccessType=rw\nDefaultValue=0x00000000\nPDOMapping=0\n\n[2701subBE]\nParameterName=Storage #190\nObjectType=0x7\nDataType=0x0007\nAccessType=rw\nDefaultValue=0x00000000\nPDOMapping=0\n\n[2701subBF]\nParameterName=Storage #191\nObjectType=0x7\nDataType=0x0007\nAccessType=rw\nDefaultValue=0x00000000\nPDOMapping=0\n\n[2701subC0]\nParameterName=Storage #192\nObjectType=0x7\nDataType=0x0007\nAccessType=rw\nDefaultValue=0x00000000\nPDOMapping=0\n\n[2701subC1]\nParameterName=Storage #193\nObjectType=0x7\nDataType=0x0007\nAccessType=rw\nDefaultValue=0x00000000\nPDOMapping=0\n\n[2701subC2]\nParameterName=Storage #194\nObjectType=0x7\nDataType=0x0007\nAccessType=rw\nDefaultValue=0x00000000\nPDOMapping=0\n\n[2701subC3]\nParameterName=Storage #195\nObjectType=0x7\nDataType=0x0007\nAccessType=rw\nDefaultValue=0x00000000\nPDOMapping=0\n\n[2701subC4]\nParameterName=Storage #196\nObjectType=0x7\nDataType=0x0007\nAccessType=rw\nDefaultValue=0x00000000\nPDOMapping=0\n\n[2701subC5]\nParameterName=Storage #197\nObjectType=0x7\nDataType=0x0007\nAccessType=rw\nDefaultValue=0x00000000\nPDOMapping=0\n\n[2701subC6]\nParameterName=Storage #198\nObjectType=0x7\nDataType=0x0007\nAccessType=rw\nDefaultValue=0x00000000\nPDOMapping=0\n\n[2701subC7]\nParameterName=Storage #199\nObjectType=0x7\nDataType=0x0007\nAccessType=rw\nDefaultValue=0x00000000\nPDOMapping=0\n\n[2701subC8]\nParameterName=Storage #200\nObjectType=0x7\nDataType=0x0007\nAccessType=rw\nDefaultValue=0x00000000\nPDOMapping=0\n\n[2701subC9]\nParameterName=Storage #201\nObjectType=0x7\nDataType=0x0007\nAccessType=rw\nDefaultValue=0x00000000\nPDOMapping=0\n\n[2701subCA]\nParameterName=Storage #202\nObjectType=0x7\nDataType=0x0007\nAccessType=rw\nDefaultValue=0x00000000\nPDOMapping=0\n\n[2701subCB]\nParameterName=Storage #203\nObjectType=0x7\nDataType=0x0007\nAccessType=rw\nDefaultValue=0x00000000\nPDOMapping=0\n\n[2701subCC]\nParameterName=Storage #204\nObjectType=0x7\nDataType=0x0007\nAccessType=rw\nDefaultValue=0x00000000\nPDOMapping=0\n\n[2701subCD]\nParameterName=Storage #205\nObjectType=0x7\nDataType=0x0007\nAccessType=rw\nDefaultValue=0x00000000\nPDOMapping=0\n\n[2701subCE]\nParameterName=Storage #206\nObjectType=0x7\nDataType=0x0007\nAccessType=rw\nDefaultValue=0x00000000\nPDOMapping=0\n\n[2701subCF]\nParameterName=Storage #207\nObjectType=0x7\nDataType=0x0007\nAccessType=rw\nDefaultValue=0x00000000\nPDOMapping=0\n\n[2701subD0]\nParameterName=Storage #208\nObjectType=0x7\nDataType=0x0007\nAccessType=rw\nDefaultValue=0x00000000\nPDOMapping=0\n\n[2701subD1]\nParameterName=Storage #209\nObjectType=0x7\nDataType=0x0007\nAccessType=rw\nDefaultValue=0x00000000\nPDOMapping=0\n\n[2701subD2]\nParameterName=Storage #210\nObjectType=0x7\nDataType=0x0007\nAccessType=rw\nDefaultValue=0x00000000\nPDOMapping=0\n\n[2701subD3]\nParameterName=Storage #211\nObjectType=0x7\nDataType=0x0007\nAccessType=rw\nDefaultValue=0x00000000\nPDOMapping=0\n\n[2701subD4]\nParameterName=Storage #212\nObjectType=0x7\nDataType=0x0007\nAccessType=rw\nDefaultValue=0x00000000\nPDOMapping=0\n\n[2701subD5]\nParameterName=Storage #213\nObjectType=0x7\nDataType=0x0007\nAccessType=rw\nDefaultValue=0x00000000\nPDOMapping=0\n\n[2701subD6]\nParameterName=Storage #214\nObjectType=0x7\nDataType=0x0007\nAccessType=rw\nDefaultValue=0x00000000\nPDOMapping=0\n\n[2701subD7]\nParameterName=Storage #215\nObjectType=0x7\nDataType=0x0007\nAccessType=rw\nDefaultValue=0x00000000\nPDOMapping=0\n\n[2701subD8]\nParameterName=Storage #216\nObjectType=0x7\nDataType=0x0007\nAccessType=rw\nDefaultValue=0x00000000\nPDOMapping=0\n\n[2701subD9]\nParameterName=Storage #217\nObjectType=0x7\nDataType=0x0007\nAccessType=rw\nDefaultValue=0x00000000\nPDOMapping=0\n\n[2701subDA]\nParameterName=Storage #218\nObjectType=0x7\nDataType=0x0007\nAccessType=rw\nDefaultValue=0x00000000\nPDOMapping=0\n\n[2701subDB]\nParameterName=Storage #219\nObjectType=0x7\nDataType=0x0007\nAccessType=rw\nDefaultValue=0x00000000\nPDOMapping=0\n\n[2701subDC]\nParameterName=Storage #220\nObjectType=0x7\nDataType=0x0007\nAccessType=rw\nDefaultValue=0x00000000\nPDOMapping=0\n\n[2701subDD]\nParameterName=Storage #221\nObjectType=0x7\nDataType=0x0007\nAccessType=rw\nDefaultValue=0x00000000\nPDOMapping=0\n\n[2701subDE]\nParameterName=Storage #222\nObjectType=0x7\nDataType=0x0007\nAccessType=rw\nDefaultValue=0x00000000\nPDOMapping=0\n\n[2701subDF]\nParameterName=Storage #223\nObjectType=0x7\nDataType=0x0007\nAccessType=rw\nDefaultValue=0x00000000\nPDOMapping=0\n\n[2701subE0]\nParameterName=Storage #224\nObjectType=0x7\nDataType=0x0007\nAccessType=rw\nDefaultValue=0x00000000\nPDOMapping=0\n\n[2701subE1]\nParameterName=Storage #225\nObjectType=0x7\nDataType=0x0007\nAccessType=rw\nDefaultValue=0x00000000\nPDOMapping=0\n\n[2701subE2]\nParameterName=Storage #226\nObjectType=0x7\nDataType=0x0007\nAccessType=rw\nDefaultValue=0x00000000\nPDOMapping=0\n\n[2701subE3]\nParameterName=Storage #227\nObjectType=0x7\nDataType=0x0007\nAccessType=rw\nDefaultValue=0x00000000\nPDOMapping=0\n\n[2701subE4]\nParameterName=Storage #228\nObjectType=0x7\nDataType=0x0007\nAccessType=rw\nDefaultValue=0x00000000\nPDOMapping=0\n\n[2701subE5]\nParameterName=Storage #229\nObjectType=0x7\nDataType=0x0007\nAccessType=rw\nDefaultValue=0x00000000\nPDOMapping=0\n\n[2701subE6]\nParameterName=Storage #230\nObjectType=0x7\nDataType=0x0007\nAccessType=rw\nDefaultValue=0x00000000\nPDOMapping=0\n\n[2701subE7]\nParameterName=Storage #231\nObjectType=0x7\nDataType=0x0007\nAccessType=rw\nDefaultValue=0x00000000\nPDOMapping=0\n\n[2701subE8]\nParameterName=Storage #232\nObjectType=0x7\nDataType=0x0007\nAccessType=rw\nDefaultValue=0x00000000\nPDOMapping=0\n\n[2701subE9]\nParameterName=Storage #233\nObjectType=0x7\nDataType=0x0007\nAccessType=rw\nDefaultValue=0x00000000\nPDOMapping=0\n\n[2701subEA]\nParameterName=Storage #234\nObjectType=0x7\nDataType=0x0007\nAccessType=rw\nDefaultValue=0x00000000\nPDOMapping=0\n\n[2701subEB]\nParameterName=Storage #235\nObjectType=0x7\nDataType=0x0007\nAccessType=rw\nDefaultValue=0x00000000\nPDOMapping=0\n\n[2701subEC]\nParameterName=Storage #236\nObjectType=0x7\nDataType=0x0007\nAccessType=rw\nDefaultValue=0x00000000\nPDOMapping=0\n\n[2701subED]\nParameterName=Storage #237\nObjectType=0x7\nDataType=0x0007\nAccessType=rw\nDefaultValue=0x00000000\nPDOMapping=0\n\n[2701subEE]\nParameterName=Storage #238\nObjectType=0x7\nDataType=0x0007\nAccessType=rw\nDefaultValue=0x00000000\nPDOMapping=0\n\n[2701subEF]\nParameterName=Storage #239\nObjectType=0x7\nDataType=0x0007\nAccessType=rw\nDefaultValue=0x00000000\nPDOMapping=0\n\n[2701subF0]\nParameterName=Storage #240\nObjectType=0x7\nDataType=0x0007\nAccessType=rw\nDefaultValue=0x00000000\nPDOMapping=0\n\n[2701subF1]\nParameterName=Storage #241\nObjectType=0x7\nDataType=0x0007\nAccessType=rw\nDefaultValue=0x00000000\nPDOMapping=0\n\n[2701subF2]\nParameterName=Storage #242\nObjectType=0x7\nDataType=0x0007\nAccessType=rw\nDefaultValue=0x00000000\nPDOMapping=0\n\n[2701subF3]\nParameterName=Storage #243\nObjectType=0x7\nDataType=0x0007\nAccessType=rw\nDefaultValue=0x00000000\nPDOMapping=0\n\n[2701subF4]\nParameterName=Storage #244\nObjectType=0x7\nDataType=0x0007\nAccessType=rw\nDefaultValue=0x00000000\nPDOMapping=0\n\n[2701subF5]\nParameterName=Storage #245\nObjectType=0x7\nDataType=0x0007\nAccessType=rw\nDefaultValue=0x00000000\nPDOMapping=0\n\n[2701subF6]\nParameterName=Storage #246\nObjectType=0x7\nDataType=0x0007\nAccessType=rw\nDefaultValue=0x00000000\nPDOMapping=0\n\n[2701subF7]\nParameterName=Storage #247\nObjectType=0x7\nDataType=0x0007\nAccessType=rw\nDefaultValue=0x00000000\nPDOMapping=0\n\n[2701subF8]\nParameterName=Storage #248\nObjectType=0x7\nDataType=0x0007\nAccessType=rw\nDefaultValue=0x00000000\nPDOMapping=0\n\n[2701subF9]\nParameterName=Storage #249\nObjectType=0x7\nDataType=0x0007\nAccessType=rw\nDefaultValue=0x00000000\nPDOMapping=0\n\n[2701subFA]\nParameterName=Storage #250\nObjectType=0x7\nDataType=0x0007\nAccessType=rw\nDefaultValue=0x00000000\nPDOMapping=0\n\n[2701subFB]\nParameterName=Storage #251\nObjectType=0x7\nDataType=0x0007\nAccessType=rw\nDefaultValue=0x00000000\nPDOMapping=0\n\n[2701subFC]\nParameterName=Storage #252\nObjectType=0x7\nDataType=0x0007\nAccessType=rw\nDefaultValue=0x00000000\nPDOMapping=0\n\n[2701subFD]\nParameterName=Storage #253\nObjectType=0x7\nDataType=0x0007\nAccessType=rw\nDefaultValue=0x00000000\nPDOMapping=0\n\n[2701subFE]\nParameterName=Storage #254\nObjectType=0x7\nDataType=0x0007\nAccessType=rw\nDefaultValue=0x00000000\nPDOMapping=0\n\n[2800]\nParameterName=Bootloader and reboot settings\nObjectType=0x8\nSubNumber=0x04\n\n[2800sub0]\nParameterName=Number of entries\nObjectType=0x7\nDataType=0x0005\nAccessType=const\nDefaultValue=0x03\nPDOMapping=0\n\n[2800sub1]\nParameterName=Reboot command\nObjectType=0x7\nDataType=0x0007\nAccessType=rw\nDefaultValue=\nPDOMapping=0\n\n[2800sub2]\nParameterName=Reboot delay time in ms\nObjectType=0x7\nDataType=0x0007\nAccessType=rw\nDefaultValue=\nPDOMapping=0\n\n[2800sub3]\nParameterName=Bootloader HW config\nObjectType=0x7\nDataType=0x0007\nAccessType=rw\nDefaultValue=0x00000000\nPDOMapping=0\n\n[3202]\nParameterName=Motor drive submode select\nObjectType=0x7\nDataType=0x0007\nAccessType=rww\nDefaultValue=0\nPDOMapping=1\n\n[3203]\nParameterName=Feedback selection\nObjectType=0x8\nSubNumber=0x04\n\n[3203sub0]\nParameterName=Number of entries\nObjectType=0x7\nDataType=0x0005\nAccessType=ro\nDefaultValue=0x03\nPDOMapping=1\n\n[3203sub1]\nParameterName=1st feedback interface\nObjectType=0x7\nDataType=0x0005\nAccessType=rww\nDefaultValue=\nPDOMapping=1\n\n[3203sub2]\nParameterName=2nd feedback interface\nObjectType=0x7\nDataType=0x0005\nAccessType=rww\nDefaultValue=\nPDOMapping=1\n\n[3203sub3]\nParameterName=3rd feedback interface\nObjectType=0x7\nDataType=0x0005\nAccessType=rww\nDefaultValue=\nPDOMapping=1\n\n[3204]\nParameterName=Feedback mapping\nObjectType=0x8\nSubNumber=0x04\n\n[3204sub0]\nParameterName=Number of entries\nObjectType=0x7\nDataType=0x0005\nAccessType=ro\nDefaultValue=0x03\nPDOMapping=1\nObjFlags=1\n\n[3204sub1]\nParameterName=Index of 1st feedback interface\nObjectType=0x7\nDataType=0x0006\nAccessType=ro\nDefaultValue=0x3380\nPDOMapping=1\nObjFlags=1\n\n[3204sub2]\nParameterName=Index of 2nd feedback interface\nObjectType=0x7\nDataType=0x0006\nAccessType=ro\nDefaultValue=0x3390\nPDOMapping=1\nObjFlags=1\n\n[3204sub3]\nParameterName=Index of 3rd feedback interface\nObjectType=0x7\nDataType=0x0006\nAccessType=ro\nDefaultValue=0x33A0\nPDOMapping=1\nObjFlags=1\n\n[320D]\nParameterName=Torque of inertia factor\nObjectType=0x8\nSubNumber=0x03\n\n[320Dsub0]\nParameterName=Number of entries\nObjectType=0x7\nDataType=0x0005\nAccessType=ro\nDefaultValue=2\nPDOMapping=0\n\n[320Dsub1]\nParameterName=Current\nObjectType=0x7\nDataType=0x0007\nAccessType=rw\nDefaultValue=0\nPDOMapping=0\n\n[320Dsub2]\nParameterName=Acceleration\nObjectType=0x7\nDataType=0x0007\nAccessType=rw\nDefaultValue=0\nPDOMapping=0\n\n[3210]\nParameterName=Motor drive parameter set\nObjectType=0x8\nSubNumber=0x0D\n\n[3210sub0]\nParameterName=Number of entries\nObjectType=0x7\nDataType=0x0005\nAccessType=ro\nDefaultValue=12\nPDOMapping=1\n\n[3210sub1]\nParameterName=Position loop, proportional gain (closed loop)\nObjectType=0x7\nDataType=0x0007\nAccessType=rww\nDefaultValue=2048\nPDOMapping=1\n\n[3210sub2]\nParameterName=Position loop, integral gain (closed loop)\nObjectType=0x7\nDataType=0x0007\nAccessType=rww\nDefaultValue=0\nPDOMapping=1\n\n[3210sub3]\nParameterName=Velocity loop, proportional gain (closed loop)\nObjectType=0x7\nDataType=0x0007\nAccessType=rww\nDefaultValue=12000\nPDOMapping=1\n\n[3210sub4]\nParameterName=Velocity loop, integral gain (closed loop)\nObjectType=0x7\nDataType=0x0007\nAccessType=rww\nDefaultValue=30\nPDOMapping=1\n\n[3210sub5]\nParameterName=Flux current loop, proportional gain (closed loop)\nObjectType=0x7\nDataType=0x0007\nAccessType=rww\nDefaultValue=8920800\nPDOMapping=1\n\n[3210sub6]\nParameterName=Flux current loop, integral gain (closed loop)\nObjectType=0x7\nDataType=0x0007\nAccessType=rww\nDefaultValue=509760\nPDOMapping=1\n\n[3210sub7]\nParameterName=Torque current loop, proportional gain (closed loop)\nObjectType=0x7\nDataType=0x0007\nAccessType=rww\nDefaultValue=8920800\nPDOMapping=1\n\n[3210sub8]\nParameterName=Torque current loop, integral gain (closed loop)\nObjectType=0x7\nDataType=0x0007\nAccessType=rww\nDefaultValue=509760\nPDOMapping=1\n\n[3210sub9]\nParameterName=Torque current loop, proportional gain (open loop)\nObjectType=0x7\nDataType=0x0007\nAccessType=rww\nDefaultValue=5097600\nPDOMapping=1\n\n[3210subA]\nParameterName=Torque current loop, integral gain (open loop)\nObjectType=0x7\nDataType=0x0007\nAccessType=rww\nDefaultValue=1911600\nPDOMapping=1\n\n[3210subB]\nParameterName=Velocity feed forward factor in per mille\nObjectType=0x7\nDataType=0x0007\nAccessType=rww\nDefaultValue=1000\nPDOMapping=1\n\n[3210subC]\nParameterName=Acceleration feed forward factor\nObjectType=0x7\nDataType=0x0007\nAccessType=rww\nDefaultValue=0\nPDOMapping=1\n\n[3212]\nParameterName=Motor drive flags\nObjectType=0x8\nSubNumber=0x05\n\n[3212sub0]\nParameterName=Number of entries\nObjectType=0x7\nDataType=0x0005\nAccessType=ro\nDefaultValue=4\nPDOMapping=0\n\n[3212sub1]\nParameterName=reserved\nObjectType=0x7\nDataType=0x0002\nAccessType=rw\nDefaultValue=0\nPDOMapping=0\n\n[3212sub2]\nParameterName=override field inversion\nObjectType=0x7\nDataType=0x0002\nAccessType=rw\nDefaultValue=0\nPDOMapping=0\n\n[3212sub3]\nParameterName=auto-setup with current controller parameters from the OD\nObjectType=0x7\nDataType=0x0002\nAccessType=rw\nDefaultValue=0\nPDOMapping=0\n\n[3212sub4]\nParameterName=use 321Ah, 321Bh, 321Ch, 321Dh, instead of 3210h\nObjectType=0x7\nDataType=0x0002\nAccessType=rw\nDefaultValue=0\nPDOMapping=0\n\n[321A]\nParameterName=Current controller parameters\nObjectType=0x8\nSubNumber=0x05\n\n[321Asub0]\nParameterName=Number of entries\nObjectType=0x7\nDataType=0x0005\nAccessType=ro\nDefaultValue=4\nPDOMapping=0\n\n[321Asub1]\nParameterName=Proportional gain Kp for Iq [mV/A]\nObjectType=0x7\nDataType=0x0007\nAccessType=rw\nDefaultValue=10212\nPDOMapping=0\n\n[321Asub2]\nParameterName=Integrator time Ti for Iq [?s]\nObjectType=0x7\nDataType=0x0007\nAccessType=rw\nDefaultValue=1094\nPDOMapping=0\n\n[321Asub3]\nParameterName=Proportional gain Kp for Id [mV/A]\nObjectType=0x7\nDataType=0x0007\nAccessType=rw\nDefaultValue=10212\nPDOMapping=0\n\n[321Asub4]\nParameterName=Integrator time Ti for Id [?s]\nObjectType=0x7\nDataType=0x0007\nAccessType=rw\nDefaultValue=1094\nPDOMapping=0\n\n[321B]\nParameterName=Velocity controller parameters\nObjectType=0x8\nSubNumber=0x03\n\n[321Bsub0]\nParameterName=Number of entries\nObjectType=0x7\nDataType=0x0005\nAccessType=ro\nDefaultValue=2\nPDOMapping=0\n\n[321Bsub1]\nParameterName=Proportional gain Kp [mA/Hz]\nObjectType=0x7\nDataType=0x0007\nAccessType=rw\nDefaultValue=384\nPDOMapping=0\n\n[321Bsub2]\nParameterName=Integrator time Ti [?s]\nObjectType=0x7\nDataType=0x0007\nAccessType=rw\nDefaultValue=100000\nPDOMapping=0\n\n[321C]\nParameterName=Position controller parameters\nObjectType=0x8\nSubNumber=0x03\n\n[321Csub0]\nParameterName=Number of entries\nObjectType=0x7\nDataType=0x0005\nAccessType=ro\nDefaultValue=2\nPDOMapping=0\n\n[321Csub1]\nParameterName=Proportional gain Kp [Hz]\nObjectType=0x7\nDataType=0x0007\nAccessType=rw\nDefaultValue=50\nPDOMapping=0\n\n[321Csub2]\nParameterName=Integrator time Ti [?s]\nObjectType=0x7\nDataType=0x0007\nAccessType=rw\nDefaultValue=0\nPDOMapping=0\n\n[321D]\nParameterName=Pre-control\nObjectType=0x8\nSubNumber=0x04\n\n[321Dsub0]\nParameterName=Number of entries\nObjectType=0x7\nDataType=0x0005\nAccessType=ro\nDefaultValue=3\nPDOMapping=0\n\n[321Dsub1]\nParameterName=Voltage pre-control [‰]\nObjectType=0x7\nDataType=0x0007\nAccessType=rw\nDefaultValue=1000\nPDOMapping=0\n\n[321Dsub2]\nParameterName=Acceleration pre-control [‰]\nObjectType=0x7\nDataType=0x0007\nAccessType=rw\nDefaultValue=1000\nPDOMapping=0\n\n[321Dsub3]\nParameterName=Velocity pre-control [‰]\nObjectType=0x7\nDataType=0x0007\nAccessType=rw\nDefaultValue=1000\nPDOMapping=0\n\n[321E]\nParameterName=Voltage limit\nObjectType=0x7\nDataType=0x0007\nAccessType=rw\nDefaultValue=100000\nPDOMapping=0\n\n[3220]\nParameterName=Analog input digits\nObjectType=0x8\nSubNumber=0x03\n\n[3220sub0]\nParameterName=Number of analog input digits\nObjectType=0x7\nDataType=0x0005\nAccessType=ro\nDefaultValue=2\nPDOMapping=0\nObjFlags=1\n\n[3220sub1]\nParameterName=Analog input #1 digit\nObjectType=0x7\nDataType=0x0003\nAccessType=ro\nDefaultValue=0\nPDOMapping=1\nObjFlags=1\n\n[3220sub2]\nParameterName=Analog input #2 digit\nObjectType=0x7\nDataType=0x0003\nAccessType=ro\nDefaultValue=0\nPDOMapping=1\nObjFlags=1\n\n[3221]\nParameterName=Analog inputs control\nObjectType=0x7\nDataType=0x0004\nAccessType=rw\nDefaultValue=0x00000000\nPDOMapping=0\n\n[3225]\nParameterName=Analog input switches\nObjectType=0x8\nSubNumber=0x02\n\n[3225sub0]\nParameterName=Number of entries\nObjectType=0x7\nDataType=0x0005\nAccessType=ro\nDefaultValue=1\nPDOMapping=0\nObjFlags=1\n\n[3225sub1]\nParameterName=Analog input switch #1\nObjectType=0x7\nDataType=0x0006\nAccessType=ro\nDefaultValue=\nPDOMapping=1\nObjFlags=1\n\n[3240]\nParameterName=Digital inputs control\nObjectType=0x8\nSubNumber=0x09\n\n[3240sub0]\nParameterName=Number of entries\nObjectType=0x7\nDataType=0x0005\nAccessType=ro\nDefaultValue=8\nPDOMapping=0\n\n[3240sub1]\nParameterName=Special function enable\nObjectType=0x7\nDataType=0x0007\nAccessType=rww\nDefaultValue=0\nPDOMapping=1\n\n[3240sub2]\nParameterName=Function inverted\nObjectType=0x7\nDataType=0x0007\nAccessType=rww\nDefaultValue=0\nPDOMapping=1\n\n[3240sub3]\nParameterName=Force enable\nObjectType=0x7\nDataType=0x0007\nAccessType=rww\nDefaultValue=0\nPDOMapping=1\n\n[3240sub4]\nParameterName=Force value\nObjectType=0x7\nDataType=0x0007\nAccessType=rww\nDefaultValue=0\nPDOMapping=1\n\n[3240sub5]\nParameterName=Raw value\nObjectType=0x7\nDataType=0x0007\nAccessType=rww\nDefaultValue=0\nPDOMapping=1\n\n[3240sub6]\nParameterName=Input Range Select\nObjectType=0x7\nDataType=0x0007\nAccessType=rww\nDefaultValue=0\nPDOMapping=1\n\n[3240sub7]\nParameterName=Differential Select\nObjectType=0x7\nDataType=0x0007\nAccessType=rww\nDefaultValue=0\nPDOMapping=1\n\n[3240sub8]\nParameterName=Routing Enable\nObjectType=0x7\nDataType=0x0007\nAccessType=rww\nDefaultValue=0\nPDOMapping=1\n\n[3242]\nParameterName=Digital Input Routing\nObjectType=0x8\nSubNumber=0x21\n\n[3242sub0]\nParameterName=Number of entries\nObjectType=0x7\nDataType=0x0005\nAccessType=ro\nDefaultValue=32\nPDOMapping=0\n\n[3242sub1]\nParameterName=Input Source for Bit #1 in 60FDh\nObjectType=0x7\nDataType=0x0005\nAccessType=rwr\nDefaultValue=0\nPDOMapping=1\n\n[3242sub2]\nParameterName=Input Source for Bit #2 in 60FDh\nObjectType=0x7\nDataType=0x0005\nAccessType=rwr\nDefaultValue=0\nPDOMapping=1\n\n[3242sub3]\nParameterName=Input Source for Bit #3 in 60FDh\nObjectType=0x7\nDataType=0x0005\nAccessType=rwr\nDefaultValue=0\nPDOMapping=1\n\n[3242sub4]\nParameterName=Input Source for Bit #4 in 60FDh\nObjectType=0x7\nDataType=0x0005\nAccessType=rwr\nDefaultValue=0\nPDOMapping=1\n\n[3242sub5]\nParameterName=Input Source for Bit #5 in 60FDh\nObjectType=0x7\nDataType=0x0005\nAccessType=rwr\nDefaultValue=0\nPDOMapping=1\n\n[3242sub6]\nParameterName=Input Source for Bit #6 in 60FDh\nObjectType=0x7\nDataType=0x0005\nAccessType=rwr\nDefaultValue=0\nPDOMapping=1\n\n[3242sub7]\nParameterName=Input Source for Bit #7 in 60FDh\nObjectType=0x7\nDataType=0x0005\nAccessType=rwr\nDefaultValue=0\nPDOMapping=1\n\n[3242sub8]\nParameterName=Input Source for Bit #8 in 60FDh\nObjectType=0x7\nDataType=0x0005\nAccessType=rwr\nDefaultValue=0\nPDOMapping=1\n\n[3242sub9]\nParameterName=Input Source for Bit #9 in 60FDh\nObjectType=0x7\nDataType=0x0005\nAccessType=rwr\nDefaultValue=0\nPDOMapping=1\n\n[3242subA]\nParameterName=Input Source for Bit #10 in 60FDh\nObjectType=0x7\nDataType=0x0005\nAccessType=rwr\nDefaultValue=0\nPDOMapping=1\n\n[3242subB]\nParameterName=Input Source for Bit #11 in 60FDh\nObjectType=0x7\nDataType=0x0005\nAccessType=rwr\nDefaultValue=0\nPDOMapping=1\n\n[3242subC]\nParameterName=Input Source for Bit #12 in 60FDh\nObjectType=0x7\nDataType=0x0005\nAccessType=rwr\nDefaultValue=0\nPDOMapping=1\n\n[3242subD]\nParameterName=Input Source for Bit #13 in 60FDh\nObjectType=0x7\nDataType=0x0005\nAccessType=rwr\nDefaultValue=0\nPDOMapping=1\n\n[3242subE]\nParameterName=Input Source for Bit #14 in 60FDh\nObjectType=0x7\nDataType=0x0005\nAccessType=rwr\nDefaultValue=0\nPDOMapping=1\n\n[3242subF]\nParameterName=Input Source for Bit #15 in 60FDh\nObjectType=0x7\nDataType=0x0005\nAccessType=rwr\nDefaultValue=0\nPDOMapping=1\n\n[3242sub10]\nParameterName=Input Source for Bit #16 in 60FDh\nObjectType=0x7\nDataType=0x0005\nAccessType=rwr\nDefaultValue=0\nPDOMapping=1\n\n[3242sub11]\nParameterName=Input Source for Bit #17 in 60FDh\nObjectType=0x7\nDataType=0x0005\nAccessType=rwr\nDefaultValue=0\nPDOMapping=1\n\n[3242sub12]\nParameterName=Input Source for Bit #18 in 60FDh\nObjectType=0x7\nDataType=0x0005\nAccessType=rwr\nDefaultValue=0\nPDOMapping=1\n\n[3242sub13]\nParameterName=Input Source for Bit #19 in 60FDh\nObjectType=0x7\nDataType=0x0005\nAccessType=rwr\nDefaultValue=0\nPDOMapping=1\n\n[3242sub14]\nParameterName=Input Source for Bit #20 in 60FDh\nObjectType=0x7\nDataType=0x0005\nAccessType=rwr\nDefaultValue=0\nPDOMapping=1\n\n[3242sub15]\nParameterName=Input Source for Bit #21 in 60FDh\nObjectType=0x7\nDataType=0x0005\nAccessType=rwr\nDefaultValue=0\nPDOMapping=1\n\n[3242sub16]\nParameterName=Input Source for Bit #22 in 60FDh\nObjectType=0x7\nDataType=0x0005\nAccessType=rwr\nDefaultValue=0\nPDOMapping=1\n\n[3242sub17]\nParameterName=Input Source for Bit #23 in 60FDh\nObjectType=0x7\nDataType=0x0005\nAccessType=rwr\nDefaultValue=0\nPDOMapping=1\n\n[3242sub18]\nParameterName=Input Source for Bit #24 in 60FDh\nObjectType=0x7\nDataType=0x0005\nAccessType=rwr\nDefaultValue=0\nPDOMapping=1\n\n[3242sub19]\nParameterName=Input Source for Bit #25 in 60FDh\nObjectType=0x7\nDataType=0x0005\nAccessType=rwr\nDefaultValue=0\nPDOMapping=1\n\n[3242sub1A]\nParameterName=Input Source for Bit #26 in 60FDh\nObjectType=0x7\nDataType=0x0005\nAccessType=rwr\nDefaultValue=0\nPDOMapping=1\n\n[3242sub1B]\nParameterName=Input Source for Bit #27 in 60FDh\nObjectType=0x7\nDataType=0x0005\nAccessType=rwr\nDefaultValue=0\nPDOMapping=1\n\n[3242sub1C]\nParameterName=Input Source for Bit #28 in 60FDh\nObjectType=0x7\nDataType=0x0005\nAccessType=rwr\nDefaultValue=0\nPDOMapping=1\n\n[3242sub1D]\nParameterName=Input Source for Bit #29 in 60FDh\nObjectType=0x7\nDataType=0x0005\nAccessType=rwr\nDefaultValue=0\nPDOMapping=1\n\n[3242sub1E]\nParameterName=Input Source for Bit #30 in 60FDh\nObjectType=0x7\nDataType=0x0005\nAccessType=rwr\nDefaultValue=0\nPDOMapping=1\n\n[3242sub1F]\nParameterName=Input Source for Bit #31 in 60FDh\nObjectType=0x7\nDataType=0x0005\nAccessType=rwr\nDefaultValue=0\nPDOMapping=1\n\n[3242sub20]\nParameterName=Input Source for Bit #32 in 60FDh\nObjectType=0x7\nDataType=0x0005\nAccessType=rwr\nDefaultValue=0\nPDOMapping=1\n\n[3243]\nParameterName=Digital input homing capture\nObjectType=0x8\nSubNumber=0x05\n\n[3243sub0]\nParameterName=Number of entries\nObjectType=0x7\nDataType=0x0005\nAccessType=ro\nDefaultValue=4\nPDOMapping=0\n\n[3243sub1]\nParameterName=Control\nObjectType=0x7\nDataType=0x0007\nAccessType=rww\nDefaultValue=0\nPDOMapping=1\n\n[3243sub2]\nParameterName=Capture Count\nObjectType=0x7\nDataType=0x0007\nAccessType=rww\nDefaultValue=0\nPDOMapping=1\n\n[3243sub3]\nParameterName=Value\nObjectType=0x7\nDataType=0x0007\nAccessType=rww\nDefaultValue=0\nPDOMapping=1\n\n[3243sub4]\nParameterName=Sensor Raw Value\nObjectType=0x7\nDataType=0x0007\nAccessType=rww\nDefaultValue=0\nPDOMapping=1\n\n[3250]\nParameterName=Digital outputs control\nObjectType=0x8\nSubNumber=0x0A\n\n[3250sub0]\nParameterName=Number of entries\nObjectType=0x7\nDataType=0x0005\nAccessType=ro\nDefaultValue=0x09\nPDOMapping=0\n\n[3250sub1]\nParameterName=No function\nObjectType=0x7\nDataType=0x0007\nAccessType=rww\nDefaultValue=0\nPDOMapping=1\n\n[3250sub2]\nParameterName=Function inverted\nObjectType=0x7\nDataType=0x0007\nAccessType=rww\nDefaultValue=0x00000000\nPDOMapping=1\n\n[3250sub3]\nParameterName=Force enable\nObjectType=0x7\nDataType=0x0007\nAccessType=rww\nDefaultValue=0x00000000\nPDOMapping=1\n\n[3250sub4]\nParameterName=Force value\nObjectType=0x7\nDataType=0x0007\nAccessType=rww\nDefaultValue=0x00000000\nPDOMapping=1\n\n[3250sub5]\nParameterName=Raw value\nObjectType=0x7\nDataType=0x0007\nAccessType=rww\nDefaultValue=\nPDOMapping=1\n\n[3250sub6]\nParameterName=Reserved1\nObjectType=0x7\nDataType=0x0007\nAccessType=rww\nDefaultValue=0x00000000\nPDOMapping=1\n\n[3250sub7]\nParameterName=Reserved2\nObjectType=0x7\nDataType=0x0007\nAccessType=rww\nDefaultValue=0x00000000\nPDOMapping=1\n\n[3250sub8]\nParameterName=Routing Enable\nObjectType=0x7\nDataType=0x0007\nAccessType=rww\nDefaultValue=0x00000000\nPDOMapping=1\n\n[3250sub9]\nParameterName=Enable Mask [Bit0=StatusLed, Bit1=ErrorLed]\nObjectType=0x7\nDataType=0x0007\nAccessType=rww\nDefaultValue=0xFFFFFFFF\nPDOMapping=1\n\n[3252]\nParameterName=Digital Output Routing\nObjectType=0x8\nSubNumber=0x05\n\n[3252sub0]\nParameterName=Number of entries\nObjectType=0x7\nDataType=0x0005\nAccessType=ro\nDefaultValue=0x04\nPDOMapping=0\n\n[3252sub1]\nParameterName=Control Bit of 60FEh:1h and Source for Brake Output\nObjectType=0x7\nDataType=0x0006\nAccessType=rwr\nDefaultValue=0x1080\nPDOMapping=1\n\n[3252sub2]\nParameterName=Control Bit of 60FEh:1h and Source for Output #1\nObjectType=0x7\nDataType=0x0006\nAccessType=rwr\nDefaultValue=0x0090\nPDOMapping=1\n\n[3252sub3]\nParameterName=Control Bit of 60FEh:1h and Source for Output #2\nObjectType=0x7\nDataType=0x0006\nAccessType=rwr\nDefaultValue=0x0091\nPDOMapping=1\n\n[3252sub4]\nParameterName=Control Bit of 60FEh:1h and Source for Output #3\nObjectType=0x7\nDataType=0x0006\nAccessType=rwr\nDefaultValue=0x0092\nPDOMapping=1\n\n[3320]\nParameterName=Analog input values\nObjectType=0x8\nSubNumber=0x03\n\n[3320sub0]\nParameterName=Number of analog input values\nObjectType=0x7\nDataType=0x0005\nAccessType=ro\nDefaultValue=0x02\nPDOMapping=0\nObjFlags=1\n\n[3320sub1]\nParameterName=Analog input #1 value\nObjectType=0x7\nDataType=0x0004\nAccessType=ro\nDefaultValue=\nPDOMapping=1\nObjFlags=1\n\n[3320sub2]\nParameterName=Analog input #2 value\nObjectType=0x7\nDataType=0x0004\nAccessType=ro\nDefaultValue=\nPDOMapping=1\nObjFlags=1\n\n[3321]\nParameterName=Analog input offsets\nObjectType=0x8\nSubNumber=0x03\n\n[3321sub0]\nParameterName=Number of analog input offsets\nObjectType=0x7\nDataType=0x0005\nAccessType=ro\nDefaultValue=0x02\nPDOMapping=0\n\n[3321sub1]\nParameterName=Analog input #1 offset\nObjectType=0x7\nDataType=0x0003\nAccessType=rw\nDefaultValue=0x0000\nPDOMapping=0\n\n[3321sub2]\nParameterName=Analog input #2 offset\nObjectType=0x7\nDataType=0x0003\nAccessType=rw\nDefaultValue=0x0000\nPDOMapping=0\n\n[3322]\nParameterName=Analog input numerators\nObjectType=0x8\nSubNumber=0x03\n\n[3322sub0]\nParameterName=Number of analog input numerators\nObjectType=0x7\nDataType=0x0005\nAccessType=ro\nDefaultValue=2\nPDOMapping=0\n\n[3322sub1]\nParameterName=Analog input #1 numerator\nObjectType=0x7\nDataType=0x0003\nAccessType=rw\nDefaultValue=1\nPDOMapping=0\n\n[3322sub2]\nParameterName=Analog input #2 numerator\nObjectType=0x7\nDataType=0x0003\nAccessType=rw\nDefaultValue=1\nPDOMapping=0\n\n[3323]\nParameterName=Analog input denominators\nObjectType=0x8\nSubNumber=0x03\n\n[3323sub0]\nParameterName=Number of analog input denominators\nObjectType=0x7\nDataType=0x0005\nAccessType=ro\nDefaultValue=2\nPDOMapping=0\n\n[3323sub1]\nParameterName=Analog input #1 denominator\nObjectType=0x7\nDataType=0x0003\nAccessType=rw\nDefaultValue=1\nPDOMapping=0\n\n[3323sub2]\nParameterName=Analog input #2 denominator\nObjectType=0x7\nDataType=0x0003\nAccessType=rw\nDefaultValue=1\nPDOMapping=0\n\n[3380]\nParameterName=Feedback Sensorless\nObjectType=0x8\nSubNumber=0x06\n\n[3380sub0]\nParameterName=Number of entries\nObjectType=0x7\nDataType=0x0005\nAccessType=ro\nDefaultValue=5\nPDOMapping=1\n\n[3380sub1]\nParameterName=Resistance [Ohm]\nObjectType=0x7\nDataType=0x0007\nAccessType=rww\nDefaultValue=0\nPDOMapping=1\n\n[3380sub2]\nParameterName=Inductance [H]\nObjectType=0x7\nDataType=0x0007\nAccessType=rww\nDefaultValue=0\nPDOMapping=1\n\n[3380sub3]\nParameterName=Magnetic flux [Vs]\nObjectType=0x7\nDataType=0x0007\nAccessType=rww\nDefaultValue=0\nPDOMapping=1\n\n[3380sub4]\nParameterName=Switch on speed [rpm]\nObjectType=0x7\nDataType=0x0007\nAccessType=rww\nDefaultValue=120\nPDOMapping=1\n\n[3380sub5]\nParameterName=Switch off speed [rpm]\nObjectType=0x7\nDataType=0x0007\nAccessType=rww\nDefaultValue=100\nPDOMapping=1\n\n[3390]\nParameterName=Feedback Hall\nObjectType=0x8\nSubNumber=0x0D\n\n[3390sub0]\nParameterName=Number of entries\nObjectType=0x7\nDataType=0x0005\nAccessType=ro\nDefaultValue=0x0C\nPDOMapping=1\n\n[3390sub1]\nParameterName=1st alignment\nObjectType=0x7\nDataType=0x0006\nAccessType=rww\nDefaultValue=\nPDOMapping=1\n\n[3390sub2]\nParameterName=2nd alignment\nObjectType=0x7\nDataType=0x0006\nAccessType=rww\nDefaultValue=\nPDOMapping=1\n\n[3390sub3]\nParameterName=3rd alignment\nObjectType=0x7\nDataType=0x0006\nAccessType=rww\nDefaultValue=\nPDOMapping=1\n\n[3390sub4]\nParameterName=4th alignment\nObjectType=0x7\nDataType=0x0006\nAccessType=rww\nDefaultValue=\nPDOMapping=1\n\n[3390sub5]\nParameterName=5th alignment\nObjectType=0x7\nDataType=0x0006\nAccessType=rww\nDefaultValue=\nPDOMapping=1\n\n[3390sub6]\nParameterName=6th alignment\nObjectType=0x7\nDataType=0x0006\nAccessType=rww\nDefaultValue=\nPDOMapping=1\n\n[3390sub7]\nParameterName=7th alignment\nObjectType=0x7\nDataType=0x0006\nAccessType=rww\nDefaultValue=\nPDOMapping=1\n\n[3390sub8]\nParameterName=8th alignment\nObjectType=0x7\nDataType=0x0006\nAccessType=rww\nDefaultValue=\nPDOMapping=1\n\n[3390sub9]\nParameterName=9th alignment\nObjectType=0x7\nDataType=0x0006\nAccessType=rww\nDefaultValue=\nPDOMapping=1\n\n[3390subA]\nParameterName=10th alignment\nObjectType=0x7\nDataType=0x0006\nAccessType=rww\nDefaultValue=\nPDOMapping=1\n\n[3390subB]\nParameterName=11th alignment\nObjectType=0x7\nDataType=0x0006\nAccessType=rww\nDefaultValue=\nPDOMapping=1\n\n[3390subC]\nParameterName=12th alignment\nObjectType=0x7\nDataType=0x0006\nAccessType=rww\nDefaultValue=\nPDOMapping=1\n\n[33A0]\nParameterName=Feedback Incremental A/B/I 1\nObjectType=0x8\nSubNumber=0x03\n\n[33A0sub0]\nParameterName=Number of entries\nObjectType=0x7\nDataType=0x0005\nAccessType=ro\nDefaultValue=0x02\nPDOMapping=1\n\n[33A0sub1]\nParameterName=Configuration\nObjectType=0x7\nDataType=0x0006\nAccessType=rww\nDefaultValue=0x0000\nPDOMapping=1\n\n[33A0sub2]\nParameterName=Alignment\nObjectType=0x7\nDataType=0x0006\nAccessType=rww\nDefaultValue=\nPDOMapping=1\n\n[3502]\nParameterName=MODBUS Rx PDO Mapping\nObjectType=0x8\nSubNumber=0x08\n\n[3502sub0]\nParameterName=Number of entries\nObjectType=0x7\nDataType=0x0005\nAccessType=rw\nDefaultValue=0x07\nPDOMapping=0\n\n[3502sub1]\nParameterName=1st object to be mapped\nObjectType=0x7\nDataType=0x0007\nAccessType=rw\nDefaultValue=0x60400010\nPDOMapping=0\n\n[3502sub2]\nParameterName=2nd object to be mapped\nObjectType=0x7\nDataType=0x0007\nAccessType=rw\nDefaultValue=0x00050008\nPDOMapping=0\n\n[3502sub3]\nParameterName=3rd object to be mapped\nObjectType=0x7\nDataType=0x0007\nAccessType=rw\nDefaultValue=0x60600008\nPDOMapping=0\n\n[3502sub4]\nParameterName=4th object to be mapped\nObjectType=0x7\nDataType=0x0007\nAccessType=rw\nDefaultValue=0x607A0020\nPDOMapping=0\n\n[3502sub5]\nParameterName=5th object to be mapped\nObjectType=0x7\nDataType=0x0007\nAccessType=rw\nDefaultValue=0x60810020\nPDOMapping=0\n\n[3502sub6]\nParameterName=6th object to be mapped\nObjectType=0x7\nDataType=0x0007\nAccessType=rw\nDefaultValue=0x60420010\nPDOMapping=0\n\n[3502sub7]\nParameterName=7th object to be mapped\nObjectType=0x7\nDataType=0x0007\nAccessType=rw\nDefaultValue=0x60FE0120\nPDOMapping=0\n\n[3602]\nParameterName=MODBUS Tx PDO Mapping\nObjectType=0x8\nSubNumber=0x07\n\n[3602sub0]\nParameterName=Number of entries\nObjectType=0x7\nDataType=0x0005\nAccessType=rw\nDefaultValue=0x06\nPDOMapping=0\n\n[3602sub1]\nParameterName=1st object to be mapped\nObjectType=0x7\nDataType=0x0007\nAccessType=rw\nDefaultValue=0x60410010\nPDOMapping=0\n\n[3602sub2]\nParameterName=2nd object to be mapped\nObjectType=0x7\nDataType=0x0007\nAccessType=rw\nDefaultValue=0x00050008\nPDOMapping=0\n\n[3602sub3]\nParameterName=3rd object to be mapped\nObjectType=0x7\nDataType=0x0007\nAccessType=rw\nDefaultValue=0x60610008\nPDOMapping=0\n\n[3602sub4]\nParameterName=4th object to be mapped\nObjectType=0x7\nDataType=0x0007\nAccessType=rw\nDefaultValue=0x60640020\nPDOMapping=0\n\n[3602sub5]\nParameterName=5th object to be mapped\nObjectType=0x7\nDataType=0x0007\nAccessType=rw\nDefaultValue=0x60440010\nPDOMapping=0\n\n[3602sub6]\nParameterName=6th object to be mapped\nObjectType=0x7\nDataType=0x0007\nAccessType=rw\nDefaultValue=0x60FD0020\nPDOMapping=0\n\n[3700]\nParameterName=Deviation error option code\nObjectType=0x7\nDataType=0x0003\nAccessType=rw\nDefaultValue=-1\nPDOMapping=0\n\n[3701]\nParameterName=Limit switch error option code\nObjectType=0x7\nDataType=0x0003\nAccessType=rw\nDefaultValue=-1\nPDOMapping=0\n\n[4012]\nParameterName=HW information\nObjectType=0x8\nSubNumber=0x02\n\n[4012sub0]\nParameterName=Number of entries\nObjectType=0x7\nDataType=0x0005\nAccessType=const\nDefaultValue=1\nPDOMapping=0\nObjFlags=1\n\n[4012sub1]\nParameterName=EEPROM size in bytes\nObjectType=0x7\nDataType=0x0007\nAccessType=const\nDefaultValue=\nPDOMapping=0\nObjFlags=1\n\n[4013]\nParameterName=HW configuration\nObjectType=0x8\nSubNumber=0x02\n\n[4013sub0]\nParameterName=Number of entries\nObjectType=0x7\nDataType=0x0005\nAccessType=const\nDefaultValue=1\nPDOMapping=0\n\n[4013sub1]\nParameterName=HW configuration #1\nObjectType=0x7\nDataType=0x0007\nAccessType=rw\nDefaultValue=0\nPDOMapping=0\n\n[4014]\nParameterName=Operating conditions\nObjectType=0x8\nSubNumber=0x06\n\n[4014sub0]\nParameterName=Number of entries\nObjectType=0x7\nDataType=0x0005\nAccessType=const\nDefaultValue=5\nPDOMapping=0\nObjFlags=1\n\n[4014sub1]\nParameterName=Voltage UB Power [mV]\nObjectType=0x7\nDataType=0x0004\nAccessType=ro\nDefaultValue=\nPDOMapping=1\nObjFlags=1\n\n[4014sub2]\nParameterName=Voltage UB Logic [mV]\nObjectType=0x7\nDataType=0x0004\nAccessType=ro\nDefaultValue=\nPDOMapping=1\nObjFlags=1\n\n[4014sub3]\nParameterName=Temperature PCB [Celsius * 10]\nObjectType=0x7\nDataType=0x0004\nAccessType=ro\nDefaultValue=\nPDOMapping=1\nObjFlags=1\n\n[4014sub4]\nParameterName=Temperature Motor [Celsius * 10]\nObjectType=0x7\nDataType=0x0004\nAccessType=ro\nDefaultValue=\nPDOMapping=1\nObjFlags=1\n\n[4014sub5]\nParameterName=Temperature Microcontroller Chip [Celsius * 10]\nObjectType=0x7\nDataType=0x0004\nAccessType=ro\nDefaultValue=\nPDOMapping=1\nObjFlags=1\n\n[4021]\nParameterName=Ballast Configuration\nObjectType=0x8\nSubNumber=0x04\n\n[4021sub0]\nParameterName=Number of entries\nObjectType=0x7\nDataType=0x0005\nAccessType=ro\nDefaultValue=3\nPDOMapping=0\n\n[4021sub1]\nParameterName=Settings [Bit0: On/Off]\nObjectType=0x7\nDataType=0x0007\nAccessType=rw\nDefaultValue=1\nPDOMapping=0\n\n[4021sub2]\nParameterName=UB Power limit [mV]\nObjectType=0x7\nDataType=0x0007\nAccessType=rw\nDefaultValue=49177\nPDOMapping=0\n\n[4021sub3]\nParameterName=UB Power hysteresis [mV]\nObjectType=0x7\nDataType=0x0007\nAccessType=rw\nDefaultValue=500\nPDOMapping=0\n\n[4040]\nParameterName=Drive serial number\nObjectType=0x7\nDataType=0x0009\nAccessType=ro\nDefaultValue=\nPDOMapping=0\nObjFlags=1\n\n[4041]\nParameterName=Device Id\nObjectType=0x7\nDataType=0x000A\nAccessType=ro\nDefaultValue=            \nPDOMapping=0\nObjFlags=1\n\n[4042]\nParameterName=Bootloader Infos\nObjectType=0x8\nSubNumber=0x04\n\n[4042sub0]\nParameterName=Number of entries\nObjectType=0x7\nDataType=0x0005\nAccessType=ro\nDefaultValue=0x03\nPDOMapping=0\nObjFlags=1\n\n[4042sub1]\nParameterName=Bootloader version\nObjectType=0x7\nDataType=0x0007\nAccessType=ro\nDefaultValue=\nPDOMapping=0\nObjFlags=1\n\n[4042sub2]\nParameterName=Bootloader supported fieldbus\nObjectType=0x7\nDataType=0x0007\nAccessType=ro\nDefaultValue=\nPDOMapping=0\nObjFlags=1\n\n[4042sub3]\nParameterName=Bootloader hw-group\nObjectType=0x7\nDataType=0x0007\nAccessType=ro\nDefaultValue=\nPDOMapping=0\nObjFlags=1\n\n") -> (error out=w13:errorcluster)  [unwired: 2 in, 2 out]
  n5 = call "Set EDS File Path.vi"("EDS File Path"=w12, "EDS in"=refnum<class "EDS.lvclass"> refnum ("EDS.lvlib:EDS.lvclass")) -> ("EDS out"=w17:refnum<class "EDS.lvclass">)  [unwired: 9 in]
  n6 = call "Parse.vi"("error in"=w13, "EDS in"=w17) -> ("error out"=w6:errorcluster, "EDS out"=w10:refnum<class "EDS.lvclass">)  [unwired: 8 in]
  n7 = call "Get Mandatory Objects.vi"("EDS in"=w10) -> ("Mandatory Objects"=w5:refnum<class "Mandatory Objects.lvclass">)  [unwired: 9 in, 1 out]
  n8 = property class="Generic Object Serializer"(reference=w9, "Properties:Type Name Handling"=Type_Name_Handling."None" ("Type Name Handling")) -> (reference out=w8:refnum<class "Generic Object Serializer.lvclass">)  [unwired: 1 in, 1 out]
  n9 = call "To JSON Text.vim"("LVClass Serializer"=w8, "Pretty Print?"=TRUE, "error in (no error)"=w6, "Anything"=w5) -> ("error out"=w1:errorcluster, "<JSON>"=w3:string)  [unwired: 6 in]
  n10 = call "Pass If Equal.vim"("error in (no error)"=w1, "Actual"=w3, "Expected"="{\n  \"SupportedObjects\":3,\n  \"Counts\":[1,2,3],\n  \"Targets\":[4096,4097,4120]\n}" ("<JSON>"), "LUnit Test Case In"="Test Case In") -> ("error out"=→"error out":errorcluster, "LUnit Test Case Out"=→"Test Case Out":refnum<class "test EDS.lvclass">)  [unwired: 6 in]
